vi "S4ICS 20240620.vi"() -> ()   [LabVIEW 2018]
uses:
  <vilib>/picture/picture.llb/imagedata.ctl
  MotorSim/MotorSim.lvclass
  StateManager/StateManager.lvclass
  Motor/Motor.lvclass
  StateManager/StateManager.lvclass/StateManager.ctl
  Messenger/Messenger.lvclass
  Motor/Motor.lvclass/Motor.ctl
  ICS/ICS.lvclass/ICS.ctl
  Message Queue/Message Cluster.ctl
  TCP-Server/TCP-Server.lvclass/TCP-Server.ctl
  TCP-Server/TCP-Server.lvclass
  ICS/ICS.lvclass
  Message Queue/Message Queue.lvlib
  MotorManager/MotorManager.lvclass
panel:
  out "version":string caption="vers."
  out "tab body":enum32{"Motors", "Config"}(tab)
  out "GFOC home":bool caption="Home"
  out "GFOC limit":bool caption="Limit"
  out "guider cam anime":picture
  out "gmir stat":T1
  out "ASEL Value":dbl
  out "CALW Value":dbl
  out "WPSEL Value":dbl
  out "GMIR Value":dbl
  out "WPROT Value":dbl
  out "GFOC Value":dbl
  out "calw stat":T1
  out "asel stat":T1
  out "wpsel stat":T1
  out "wprot stat":T1
  out "gfoc stat":T1
  out "asel lim on":bool caption="Limit ON"
  out "asel sec ON":bool caption="Sec. ON"
  out "asel lim off":bool caption="Limit OFF"
  out "asel sec off":bool caption="Sec. OFF"
  out "asel anime":picture
  out "asel background":picture
  out "wpsel sec/2":bool caption="Sec. L/4"
  out "wpsel sec/4":bool caption="Sec. L/2"
  out "wp home":bool caption="Home"
  out "wprot ctl":dbl(knob) scale=0.0..360.0
  out "wpsel lim/2":bool caption="Limit L/4"
  out "wpsel lim/4":bool caption="Limit L/2"
  out "wpsel anime":picture
  out "calw2":bool caption="CW 2"
  out "calw1":bool caption="CW 1"
  out "calw0":bool caption="CW 0"
  out "calw knob":cluster{dbl, dbl, dbl, dbl, dbl}(knob)={10.0, 82.0, 154.0, 226.0, 298.0} scale=0.0..360.0
  out "GMIR home":bool caption="Home"
  out "gmir knob":dbl(knob) scale=0.0..360.0
  out "asel image":T2
  in  "tips":T3(array[cluster])=[{"tip name"="login: server off", "PT"="Estado do servidor TCP/IP do S4ICS\npara clientes da rede (e.g. S4GUI).", "EN"="State of the S4ICS TCP/IP server\nfor network clients (e.g. S4GUI)."}, {"tip name"="login: exit", "PT"="Encerra a execução do programa\nS4ICS.", "EN"="Ends the execution of the S4ICS\nprogram."}, {"tip name"="login: language", "PT"="Seleciona a linguagem dos textos\nde ajuda e das dicas ou as ocultam.", "EN"="Select the language of the texts\nof help and tips or hide them."}, {"tip name"="login: user", "PT"="Nome cadastrado do usuário para\npermitir sua identificação.", "EN"="User's registered name to allow\nidentification."}, {"tip name"="login: password", "PT"="Senha cadastrada do usuário\n(digitada no 1o. acesso do usuário).", "EN"="User's registered password\n(entered on user's first login)."}, {"tip name"="login: help", "PT"="Descreve a função dos elementos\nmostrados no painel do S4ICS.", "EN"="Describes the function of elements\nshown on the S4ICS panel."}, {"tip name"="login: login", "PT"="Acesso ao S4ICS com a permissão\nestabelecida pelo administrador.", "EN"="Access to S4ICS according to\npermission set by administrator."}, {"tip name"="stopped: start srv", "PT"="Habilita o servidor TCP/IP do S4ICS\n(faz logout automaticamente).", "EN"="Enables S4ICS TCP/IP server\n(automatically logs out)."}, {"tip name"="stopped: exit", "PT"="Fecha o programa S4ICS.", "EN"="Ends S4ICS program execution."}, {"tip name"="stopped: assist", "PT"="Abre janela para testar e estacionar\nos mecanismos do instrumento.", "EN"="Opens window to test and park\ninstrument mechanisms."}, {"tip name"="stopped: setup", "PT"="Abre a janela de configuração do\ninstrumento (acesso restrito). ", "EN"="Opens the window of instrument\nconfiguration (restricted access)."}, {"tip name"="stopped: control", "PT"="Abre a janela para controlar os\nmecanismos (acesso restrito).", "EN"="Opens the window to control the\nmechanisms (restricted access)."}, {"tip name"="stopped: logout", "PT"="Libera o S4ICS para outro usuário.", "EN"="Release S4ICS for another user."}, {"tip name"="running: stop", "PT"="Desabilita o servidor\nTCP/IP doS4ICS.", "EN"="Disables S4ICS TCP/IP server."}, {"tip name"="running: logout", "PT"="Libera o S4ICS para outro usuário.", "EN"="Release S4ICS for another user."}, {"tip name"="setup: save", "PT"="Salva as alterações mantendo o\nnome do arquivo de  configuração.", "EN"="Save the changes keeping the\nname of the configuration file."}, {"tip name"="setup: save as", "PT"="Salva as alterações em um arquivo\nde  configuração com outro nome.", "EN"="Save changes to a file\nunder another name."}, {"tip name"="setup: help", "PT"="Descreve a função dos elementos\nmostrados no painel abaixo.", "EN"="Describes the function of elements\nshown on below panel."}, {"tip name"="setup: cfg file", "PT"="Nome do arquivo da\nconfiguração atual.\n", "EN"="File name of current configuration."}, {"tip name"="setup: cfg user", "PT"="Nome do usuário que salvou\na configuração atual.", "EN"="Username who saved\nthe current configuration."}, {"tip name"="setup: cfg date", "PT"="Data da configuração atual.", "EN"="Date of current configuration."}, {"tip name"="setup: return", "PT"="Retorna ao menu anterior.", "EN"="Return to previous menu."}, {"tip name"="assist: return", "PT"="Retorna ao menu anterior.", "EN"="Return to previous menu."}, {"tip name"="control: return", "PT"="Retorna ao menu anterior.", "EN"="Return to previous menu."}, {"tip name"="cfg: previous", "PT"="Mostra e seleciona\no usuário anterior.", "EN"="Show and select\nprevious user."}, {"tip name"="cfg: next", "PT"="Mostra e seleciona\no próximo usuário.", "EN"="Show and select\nthe next user."}, {"tip name"="cfg: delete", "PT"="Remove da lista o\nusuário selecionado.", "EN"="Remove from the list\nthe selected user."}, {"tip name"="cfg: name", "PT"="Nome do novo usuário\npara ser inserido na lista.", "EN"="New user name to be\ninserted into the list."}, {"tip name"="cfg: insert", "PT"="Insere na lista o novo usuário com\no nome e a permissão indicados.", "EN"="Insert the new user with the\ngiven name and permission."}, {"tip name"="cfg: permission", "PT"="Permissão do usuário. Restringir\nas atribuições Admin e Control.", "EN"="User permission. Restrict the\nAdmin and Control assignments."}, {"tip name"="cfg: change", "PT"="Atribui a atribuição ao lado\npara o usuário selecionado.", "EN"="Assign left assignment\nfor the selected user."}, {"tip name"="cfg: auto", "PT"="Tempo limite de inatividade para\nlogout automático do usuário.", "EN"="Inactivity timeout to\nautomatic user logout."}, {"tip name"="cfg: enable", "PT"="Permite o envio de e-mails\nde manutenção e configuração.", "EN"="Allows sending maintenance\nand configuration emails."}, {"tip name"="cfg: service", "PT"="Endereço IP e porta do\nservidor de e-mail.", "EN"="IP address and port\nof email server."}, {"tip name"="cfg: admin", "PT"="Endereço de e-mail que receberá\nnotificações de nova configuração.", "EN"="Email address that will receive\nnew configuration notifications."}, {"tip name"="cfg: maint", "PT"="Endereço de email que irá receber\nnotificações de erro e alarme.", "EN"="Email address that will receive\nerror and alarm notifications."}, {"tip name"="cfg: check", "PT"="Envia e-mail e confere recebimento\npara testar o servidor de e-mail.", "EN"="Send emails and check receipt\nto test the email server."}, {"tip name"="cfg: ok", "PT"="Resultado do teste do servidor de\ne-mail. Aguarde alguns segundos.", "EN"="Test result from email server test.\nPlease, wait a few seconds."}, {"tip name"="cfg: srv ip", "PT"="Endereço IP do servidor do S4ICS:\nlocalhost ou IP local (ver abaixo).", "EN"="S4ICS server IP address:\nlocalhost or local IP (see below)."}, {"tip name"="cfg: srv port", "PT"="Porta do servidor do S4ICS que\nserá usada pelos clientes (S4GUI).", "EN"="S4ICS server port used\nby clients (like S4GUI)."}, {"tip name"="cfg: srv timeout", "PT"="Tempo de espera pela conexão:\nmenor tempo exigido pelo servidor do S4ICS.", "EN"="Connection wait time: lower time\nrequired by S4ICS server."}, {"tip name"="cfg: IP1", "PT"="Porta IP ativa (com conexão)\nneste computador.", "EN"="Active IP port (with connection)\non this computer."}, {"tip name"="cfg: IP2", "PT"="Porta IP ativa (com conexão)\nneste computador.", "EN"="Active IP port (with connection)\non this computer."}]
  in  "pubTime0mq":i32=3000 caption="Pub Time*"
  in  "0mqEndpoint":string="tcp://*:54030" caption="PUB Socket (tcp://*:54030)*"
  in  "address":string="localhost" caption="Address"
  in  "runMinimized":bool
  in  "autoSS":bool
  in  "log help":bool
  in  "enabled log":string="012345" caption="LOG Enable"
  in  "WPSEL mode":string(combo)="Control" caption="Mechanism Mode"
  in  "CALW mode":string(combo)="Control" caption="Mechanism Mode"
  in  "GFOC mode":string(combo)="Control" caption="Mechanism Mode"
  in  "animation":bool
  in  "full init":bool
  in  "timeout":i32=100 caption="Timeout"
  in  "port":u16=54165 caption="Port"
  in  "pwrPM mains":bool=TRUE caption="Mains"
  in  "pwrPM password":string="ubnt" caption="Password"
  in  "pwrPM user":string="ubnt" caption="User"
  in  "pwrPM outlet":u16=5 caption="Outlet"
  in  "pwrPM port":u16=6080 caption="Port"
  in  "pwrPM ip":string="192.168.1.20" caption="IP"
  in  "pwrGD mains":bool=TRUE caption="Mains"
  in  "pwrGD password":string="ubnt" caption="Password"
  in  "pwrGD user":string="ubnt" caption="User"
  in  "pwrGD outlet":u16=6 caption="Outlet"
  in  "pwrGD port":u16=6080 caption="Port"
  in  "pwrGD ip":string="192.168.1.20" caption="IP"
  in  "GMIR disabled":bool
  in  "GMIR mode":string(combo)="Control" caption="Mechanism Mode"
  in  "GMIR ip":string="192.168.1.249" caption="ip"
  in  "GFOC positions":cluster{"pos_name":string, "pos_value":dbl}[](array[cluster])=[{"pos_name"="OFFSET", "pos_value"=0.0}] caption="GFOC" {"pos_value" min=-400.0 max=400.0 step=0.1}
  in  "GMIR positions":cluster{"pos_name":string, "pos_value":dbl}[](array[cluster])=[{"pos_name"="OFFSET", "pos_value"=0.0}] caption="GMIR" {"pos_value" min=-10.0 max=110.0 step=0.1}
  in  "WPSEL disabled":bool
  in  "WPROT disabled":bool
  in  "WPSEL ip":string="192.168.1.246" caption="ip"
  in  "WPROT mode":string(combo)="Control" caption="Mechanism Mode"
  in  "WPROT ip":string="192.168.1.245" caption="ip"
  in  "WPSEL positions":cluster{"pos_name":string, "pos_value":dbl}[](array[cluster])=[{"pos_name"="OFFSET", "pos_value"=0.0}, {"pos_name"="L/4", "pos_value"=0.0}, {"pos_name"="OFF", "pos_value"=400000.0}, {"pos_name"="L/2", "pos_value"=800000.0}] caption="WPSEL" {"pos_value" min=-400.0 max=400.0 step=0.1}
  in  "WPROT positions":cluster{"pos_name":string, "pos_value":dbl}[](array[cluster])=[{"pos_name"="OFFSET", "pos_value"=0.0}, {"pos_name"="WP1", "pos_value"=0.0}, {"pos_name"="WP2", "pos_value"=1875.0}, {"pos_name"="WP3", "pos_value"=3750.0}, {"pos_name"="WP4", "pos_value"=5625.0}, {"pos_name"="WP5", "pos_value"=7500.0}, {"pos_name"="WP6", "pos_value"=9375.0}, {"pos_name"="WP7", "pos_value"=11250.0}, {"pos_name"="WP8", "pos_value"=13125.0}, {"pos_name"="WP9", "pos_value"=15000.0}, {"pos_name"="WP10", "pos_value"=16875.0}, {"pos_name"="WP11", "pos_value"=18750.0}, {"pos_name"="WP12", "pos_value"=20625.0}, {"pos_name"="WP13", "pos_value"=22500.0}, {"pos_name"="WP14", "pos_value"=24375.0}, {"pos_name"="WP15", "pos_value"=26250.0}, {"pos_name"="WP16", "pos_value"=28125.0}] caption="WPROT" {"pos_value" min=-10.0 max=110.0 step=0.1}
  in  "CALW disabled":bool
  in  "ASEL disabled":bool
  in  "CALW ip":string="192.168.1.247" caption="ip"
  in  "ASEL mode":string(combo)="Control" caption="Mechanism Mode"
  in  "ASEL ip":string="192.168.1.248" caption="ip"
  in  "CALW positions":cluster{"pos_name":string, "pos_value":dbl}[](array[cluster])=[{"pos_name"="OFFSET", "pos_value"=0.0}, {"pos_name"="OFF", "pos_value"=0.0}, {"pos_name"="POLARIZER", "pos_value"=12000.0}, {"pos_name"="PINHOLE", "pos_value"=24000.0}, {"pos_name"="SHUTTER", "pos_value"=36000.0}, {"pos_name"="DEPOLARIZER", "pos_value"=48000.0}] caption="CALW" {"pos_value" min=-400.0 max=400.0 step=0.1}
  in  "ASEL positions":cluster{"pos_name":string, "pos_value":dbl}[](array[cluster])=[{"pos_name"="OFFSET", "pos_value"=0.0}, {"pos_name"="OFF", "pos_value"=0.0}, {"pos_name"="ON", "pos_value"=4800.0}] caption="ASEL" {"pos_value" min=-10.0 max=110.0 step=0.1}
  in  "S4ICS password":string="se4RFVgy&8"
  in  "S4ICS login":string="s4ics@lna.br"
  in  "S4ICS email":string="s4ics@lna.br" caption="S4ICS account"
  in  "auto logout":u32=200 caption="Auto Logout period" min=30 max=3000
  out "email ok":bool
  in  "check email":bool
  in  "maint. email":string="frodrigues@lna.br" caption="Maintenance"
  in  "admin email":string="nivaldo@lna.br" caption="Configuration"
  in  "email service":string="smtp.gmail.com:587" caption="Server IP:PORT"
  out "user list":T4(array[cluster]) caption="Name                 Permission        PW"
  in  "user delete":bool
  in  "user permission":string(combo)="Start / Stop" caption="Permission"
  in  "change permission":bool
  in  "user insert":bool
  in  "user name":string caption="New User"
  in  "user previous":bool
  in  "user next":bool
  in  "email enable":bool caption="Email service"
  in  "channel":T5(ring)=enum."Inner TCP/IP" caption="Channel"
  out "local IP 1":string
  out "local IP 2":string
  in  "comm help":bool
  out "tab menu":T6(tab)
  in  "login help":bool
  in  "loginPW":string caption="Password"
  in  "loginUser":string caption="User Name"
  in  "login":bool
  out "server":bool
  in  "exitLogin":bool
  in  "language":enum32{"PT", "EN", "NONE"}(radio)=enum."NONE"
  in  "stop server":bool
  in  "logout running":bool
  in  "exitStopped":bool
  in  "logout stopped":bool
  in  "start server":bool
  in  "control":bool
  in  "setup":bool
  in  "assist":bool
  in  "return assist":bool
  in  "save as":bool
  out "last cfg date":string caption="Date"
  out "last cfg user":string caption="User"
  in  "save config":bool
  in  "return setup":bool
  in  "config help":bool
  out "cfgFile":string caption="CONFIG FILE"
  out "control response":string caption="Response"
  in  "control instruction":string caption="Instruction"
  in  "control send":bool
  in  "control jump":bool caption="JUMP"
  in  "control position":dbl caption="Mech. Position"
  in  "return control":bool
  in  "control stop":bool
  in  "control motor sel":T7(radio) caption="Motor"
  # "GFOC - Guiding Focuser"
  # "GMIR - Guiding Mirror"
  # "CALW - Calibration Wheel"
  # "FOCUSER"
  # "CLEAR"
  # "GUIDING"
  # "CAMERA"
  # "POLARIZER"
  # "PINHOLE"
  # "SHUTTER"
  # "PATROL"
  # "MIRROR"
  # "DEPOLARIZER"
  # "WPROT - Waveplate Rotator"
  # "WPSEL - Waveplate Selector"
  # "ASEL - Analyser Selector"
  # "POLARIMETRIC MECHANISMS"
  # "SERVER COMMUNICATION"
  # "USER LIST"
  # "(*) Requires EXIT after SAVE\n      Exigido EXIT depois de SAVE"
  # "SIMULATION"
  # "ANIMATION"
  # "ON"
  # "FAST"
  # "FULL"
  # "OFF"
  # "s"
  # "EMAIL SETTINGS"
  # "GUIDING MECHANISMS"
  # "POWER"
  # "POWER"
  # "GMIR & GFOC"
  # "GFOC motor is driven by the GMIR cotroller."
  # "IDENTIFICATION"
  # "LAST CONFIGURATION"
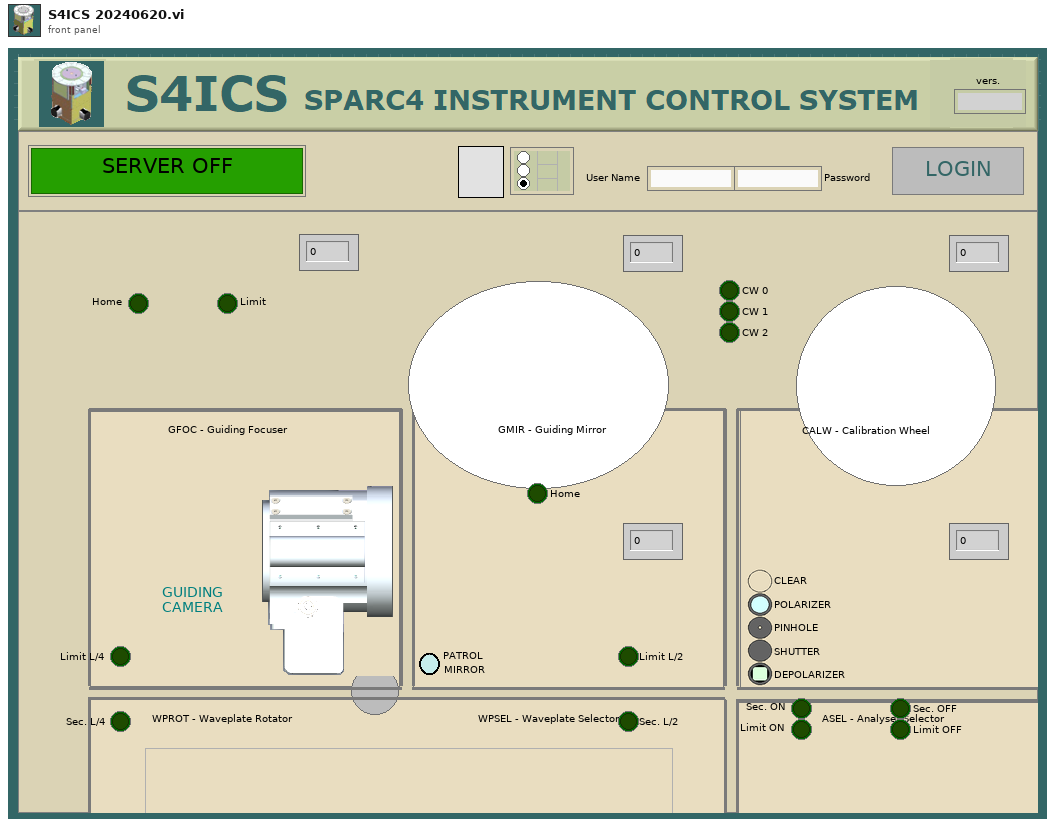
[diagram p1: front panel]
types:
  T1 = cluster{"mode":string, "condition":string, "position":string, "pos_name":string, "pos_id":string}
  T2 = typedef "imagedata.ctl" = cluster{"image type":i32, "image depth":i32, "image":u8[], "mask":u8[], "colors":u32[], "Rectangle":cluster{"left":i16, "top":i16, "right":i16, "bottom":i16}}
  T3 = cluster{"tip name":string, "PT":string, "EN":string}[]
  T4 = cluster{"name":string, "permission":string, "password":string}[]
  T5 = enum32{"Local Panel", "Inner TCP/IP", "Outer TCP/IP", "MQTT", "ZeroMQ"}
  T6 = enum32{"Login", "Running", "Stopped", "Assist", "Setup", "Control"}
  T7 = enum32{"No Selection", "control WPROT", "control WPSEL", "control ASEL", "control CALW", "control GFOC", "control GMIR"}
  T8 = cluster{"S4commandQueueName":string, "S4statusQueueName":string, "comm configuration":cluster{"channel":enum32{"Local Panel", "Inner TCP/IP", "Outer TCP/IP", "MQTT", "ZeroMQ"}, "address":string, "port":u16, "timeout":i32}}
  T9 = enum32{"Motors", "Config", "Status", "Anime", "Param"}
  T10 = cluster{"email service":string, "maint. email":string, "admin email":string, "S4ICS email":string, "S4ICS login":string, "S4ICS password":string, "email enabled":bool}
  T11 = cluster{"period":u32, "initial position (0)":i32, "translation (100)":i32, "forward":bool}[]
  T12 = enum8{"Enabled", "Disabled", "Disabled and Grayed Out"}
  T13 = enum32{"Invalid", "Standard", "Closed", "Hidden", "Minimized", "Maximized"}
  T14 = cluster{"left":i16, "top":i16, "right":i16, "bottom":i16}
  T15 = enum32{"Login", "Stopped", "Running", "Setup", "Assist", "Control"}
  T16 = enum16{"Wait", "ActiveInit", "ActiveGoto", "ActiveUpdate", "ActiveStop", "ActiveFinish", "SimInit", "SimGoto", "SimUptate", "SimFinish", "CyclicStart", "CyclicUpdate", "CyclicFinish"}
  T17 = cluster{"action":string, "param":string, "pos_name":string, "pos_idx":i32, "ack":bool, "stop":bool, "offset":bool, "immediate":bool, "instructions":string[]}
  T18 = typedef "Message Queue.lvlib/Message Cluster.ctl" = cluster{"Message":string, "Message Data":variant}
  T19 = cluster{"channel":enum32{"Local Panel", "Inner TCP/IP", "Outer TCP/IP", "MQTT", "ZeroMQ"}, "address":string, "port":u16, "timeout":i32}
  T20 = cluster{"name":string, "permission":string, "password":string}
  T21 = cluster{"[0]":dbl, "[1]":dbl, "[2]":dbl, "[3]":dbl, "[4]":dbl}
  T22 = enum32{"invalid app kind", "Development System", "Run Time System", "Student Edition", "Embedded LabVIEW", "Evaluation", "Custom"}
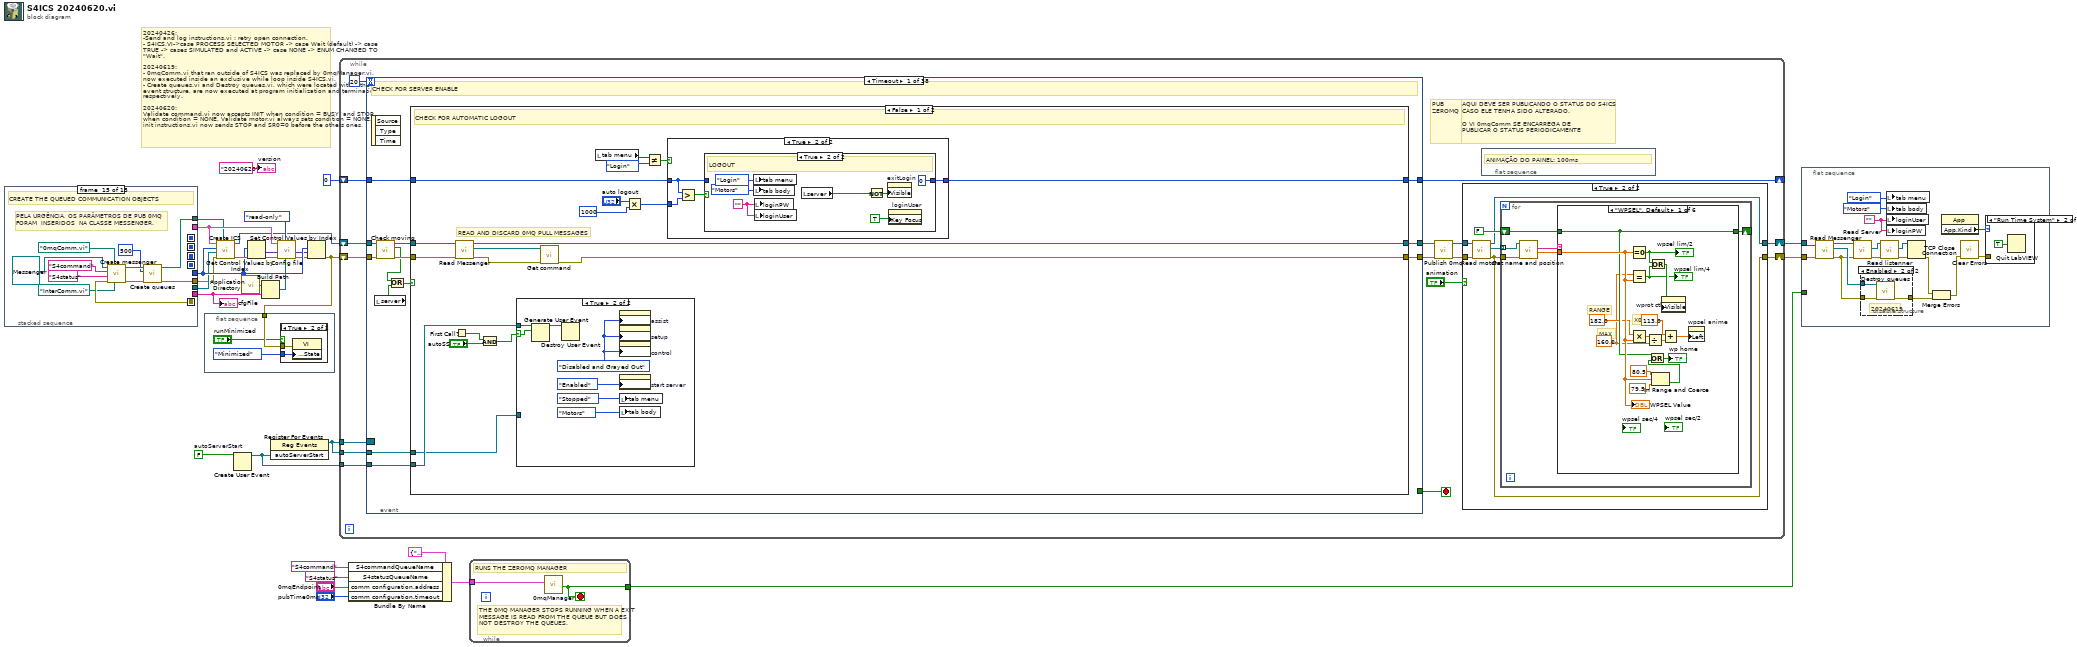
[diagram p0: block diagram]
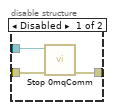
[diagram p3: hidden frame]
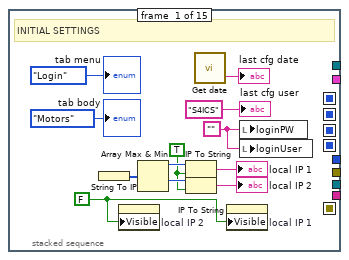
[diagram p5: hidden frame]
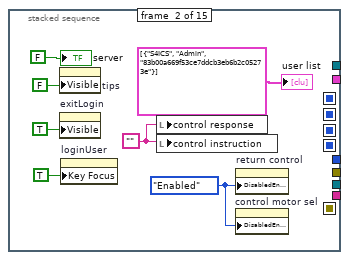
[diagram p6: hidden frame]
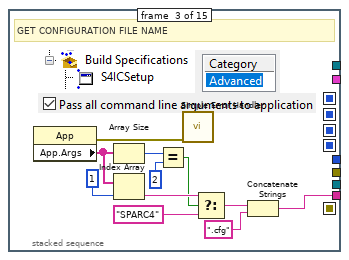
[diagram p7: hidden frame]
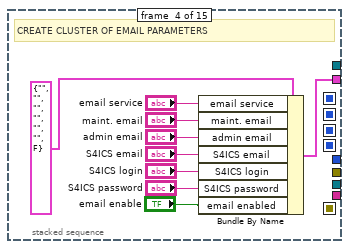
[diagram p8: hidden frame]
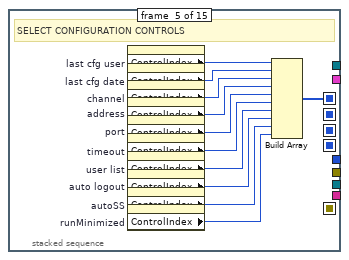
[diagram p9: hidden frame]
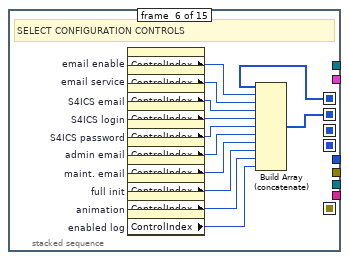
[diagram p10: hidden frame]
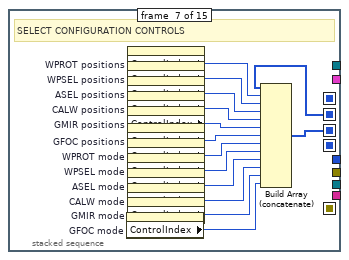
[diagram p11: hidden frame]
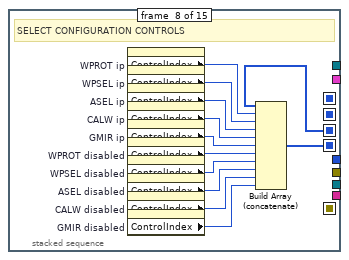
[diagram p12: hidden frame]
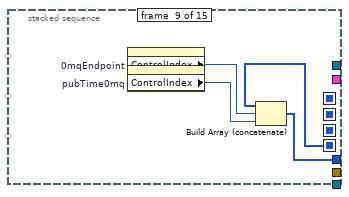
[diagram p13: hidden frame]
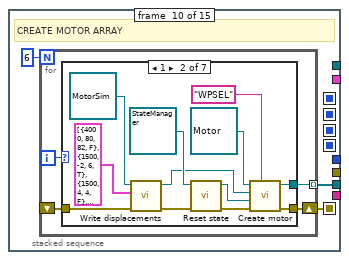
[diagram p14: hidden frame]
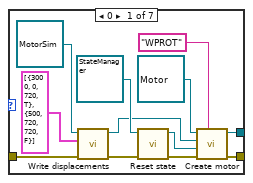
[diagram p15: hidden frame]
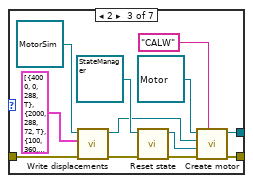
[diagram p16: hidden frame]
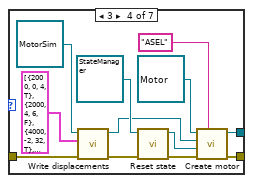
[diagram p17: hidden frame]
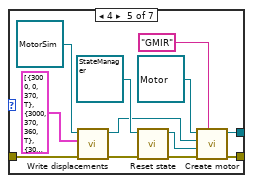
[diagram p18: hidden frame]
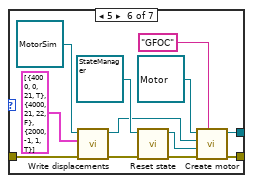
[diagram p19: hidden frame]
diagram:
  w12 = FALSE  # autoServerStart
  # "20240426:\n-Send and log instructions.vi : retry open connection.\n- S4ICS.VI->case PROCESS SELECTED MOTOR -> case Wait (default) -> case TRUE -> cases SIMULATED and ACTIVE -> case NONE -> ENUM CHANGED TO  \"Wait\".\n\n20240619:\n- 0mqComm.vi that ran outside of S4ICS was replaced by 0mqManager.vi, now executed inside an exclusive while loop inside S4ICS.vi.\n- Create queues.vi and Destroy queues.vi, which were located within the event structure, are now executed at program initialization and termination, respectively.\n\n20240620:\nValidate command.vi now accepts INIT when condition = BUSY, and STOP when condition = NONE. Validate motor.vi always sets condition = NONE. Get init instructions.vi now sends STOP and SR0=0 before the others ones."
  n1 = stacked-sequence {
    seq-local: [_ _ _ _ w78 _ _ _ _ _ _ _ _ _ _] -> [_ _ _ _ _ w92 _ _ _ _ _ _ _ _ _]
    seq-local: [_ _ _ _ _ w84 _ _ _ _ _ _ _ _ _] -> [_ _ _ _ _ _ w99 _ _ _ _ _ _ _ _]
    seq-local: [_ _ _ _ _ _ w98 _ _ _ _ _ _ _ _] -> [_ _ _ _ _ _ _ w118 _ _ _ _ _ _ _]
    seq-local: [_ _ _ _ _ _ _ _ _ w124 _ _ _ _ _] -> [_ _ _ _ _ _ _ _ _ _ _ _ _ _ w240]
    seq-local: [_ _ _ _ _ _ _ w107 _ _ _ _ _ _ _] -> [_ _ _ _ _ _ _ _ w122 _ _ _ _ _ _]
    tunnel: [_ _ w58 _ _ _ _ _ _ _ _ _ _ _ _] -> w27
    tunnel: [_ _ _ w61 _ _ _ _ _ _ _ _ _ _ _] -> w24
    tunnel: [_ _ _ _ _ _ _ _ w121 _ _ _ _ _ _] -> w26
    tunnel: [_ _ _ _ _ _ _ _ _ w125 _ _ _ _ _] -> w25
    tunnel: [_ _ _ _ _ _ _ _ _ _ _ _ _ _ w235] -> w15
    tunnel: [_ _ _ _ _ _ _ _ _ _ _ _ _ _ w234] -> w14
    frame #0 {
      w31 = FALSE
      w37 = TRUE
      w32 = ""
      # "INITIAL SETTINGS"
      n2 = String To IP() -> (0:w40:u32[])  [unwired: 1 in]
      n3 = property on="local IP 2" class="Str"("Visible"=w31) -> ()  [unwired: 2 in, 2 out]
      n4 = Array Max & Min(array=w40) -> (max value=w39:u32, min value=w38:u32)  [unwired: 2 out]
      n5 = IP To String(1:w37, 2:w39) -> (0:→"local IP 1":string)
      n6 = IP To String(1:w37, 2:w38) -> (0:→"local IP 2":string)
      n7 = call "Get date.vi"() -> ("date/time string"=→"last cfg date":string)  [unwired: 3 in]
      n8 = property on="local IP 1" class="Str"("Visible"=w31) -> ()  [unwired: 2 in, 2 out]
      n9 = local write "loginPW"(w32) -> ()
      n10 = local write "loginUser"(w32) -> ()
      "last cfg user" <- "S4ICS" ("last user")
      "tab menu" <- T6."Login" ("tab menu")
      "tab body" <- T9."Motors" ("tab body")
    }
    frame #1 {
      w43 = ""
      w44 = T12."Enabled" ("Disabled")
      n11 = property on="tips" class="Arr (strict)"("Visible"=FALSE) -> ()  [unwired: 2 in, 2 out]
      n12 = property on="exitLogin" class="Bool"("Visible"=TRUE) -> ()  [unwired: 2 in, 2 out]
      n13 = property on="loginUser" class="Str"("Key Focus"=TRUE) -> ()  [unwired: 2 in, 2 out]
      n14 = local write "control response"(w43) -> ()
      n15 = local write "control instruction"(w43) -> ()
      n16 = property on="return control" class="Bool"("DisabledEnum"=w44) -> ()  [unwired: 2 in, 2 out]
      n17 = property on="control motor sel" class="RadioBtnsControl (strict)"("DisabledEnum"=w44) -> ()  [unwired: 2 in, 2 out]
      "server" <- FALSE
      "user list" <- T4 [{"name"="S4ICS", "permission"="Admin", "password"="83b00a669f53ce7ddcb3eb6b2c05273e"}] ("users")
    }
    frame #2 {
      # "GET CONFIGURATION FILE NAME"
      n18 = property class="App"() -> (error out=w59:errorcluster, "App.Args"=w55:string[])  [unwired: 2 in, 1 out]
      n19 = Array Size(array=w55) -> (size(s)=w57:i32)
      n20 = Index Array(array=w55, index=1) -> (element=w54:string)
      n21 = Equal?(x=w57, y=2 ("x")) -> (x = y?=w50:bool)
      n22 = call <vilib>:"Simple Error Handler.vi"("error in (no error)"=w59) -> ()  [unwired: 4 in, 5 out]
      n23 = Select(t=w54, s=w50, f="SPARC4" ("string")) -> (s? t:f=w52:string)
      n24 = Concatenate Strings(w52, ".cfg" ("string")) -> (w58:string)
    }
    frame #3 {
      # "CREATE CLUSTER OF EMAIL PARAMETERS"
      n25 = Bundle By Name(cluster=T10 {"email service"="", "maint. email"="", "admin email"="", "S4ICS email"="", "S4ICS login"="", "S4ICS password"="", "email enabled"=FALSE} ("email cluster"), "email service"="email service", "maint. email"="maint. email", "admin email"="admin email", "S4ICS email"="S4ICS email", "S4ICS login"="S4ICS login", "S4ICS password"="S4ICS password", "email enabled"="email enable") -> (w61:T10)
    }
    frame #4 {
      # "SELECT CONFIGURATION CONTROLS"
      n26 = property on="last cfg user" class="Str"() -> ("ControlIndex"=w79:i32)  [unwired: 2 in, 2 out]
      n27 = property on="last cfg date" class="Str"() -> ("ControlIndex"=w80:i32)  [unwired: 2 in, 2 out]
      n28 = property on="channel" class="Enum (strict)"() -> ("ControlIndex"=w72:i32)  [unwired: 2 in, 2 out]
      n29 = property on="address" class="Str"() -> ("ControlIndex"=w73:i32)  [unwired: 2 in, 2 out]
      n30 = property on="port" class="DigNum (strict)"() -> ("ControlIndex"=w74:i32)  [unwired: 2 in, 2 out]
      n31 = property on="timeout" class="DigNum (strict)"() -> ("ControlIndex"=w75:i32)  [unwired: 2 in, 2 out]
      n32 = property on="user list" class="Arr (strict)"() -> ("ControlIndex"=w76:i32)  [unwired: 2 in, 2 out]
      n33 = property on="auto logout" class="DigNum (strict)"() -> ("ControlIndex"=w77:i32)  [unwired: 2 in, 2 out]
      n34 = property on="autoSS" class="Bool (strict)"() -> ("ControlIndex"=w71:i32)  [unwired: 2 in, 2 out]
      n35 = property on="runMinimized" class="Bool (strict)"() -> ("ControlIndex"=w70:i32)  [unwired: 2 in, 2 out]
      n36 = Build Array(w79, w80, w72, w73, w74, w75, w76, w77, w71, w70) -> (w78:i32[])
    }
    frame #5 {
      # "SELECT CONFIGURATION CONTROLS"
      n37 = property on="email enable" class="Bool (strict)"() -> ("ControlIndex"=w88:i32)  [unwired: 2 in, 2 out]
      n38 = property on="email service" class="Str"() -> ("ControlIndex"=w89:i32)  [unwired: 2 in, 2 out]
      n39 = property on="S4ICS email" class="Str"() -> ("ControlIndex"=w90:i32)  [unwired: 2 in, 2 out]
      n40 = property on="S4ICS login" class="Str"() -> ("ControlIndex"=w91:i32)  [unwired: 2 in, 2 out]
      n41 = property on="S4ICS password" class="Str"() -> ("ControlIndex"=w87:i32)  [unwired: 2 in, 2 out]
      n42 = property on="admin email" class="Str"() -> ("ControlIndex"=w86:i32)  [unwired: 2 in, 2 out]
      n43 = property on="maint. email" class="Str"() -> ("ControlIndex"=w85:i32)  [unwired: 2 in, 2 out]
      n44 = property on="full init" class="Bool (strict)"() -> ("ControlIndex"=w83:i32)  [unwired: 2 in, 2 out]
      n45 = property on="animation" class="Bool (strict)"() -> ("ControlIndex"=w82:i32)  [unwired: 2 in, 2 out]
      n46 = property on="enabled log" class="Str"() -> ("ControlIndex"=w81:i32)  [unwired: 2 in, 2 out]
      n47 = Build Array (concatenate)(w92, w88, w89, w90, w91, w87, w86, w85, w83, w82, w81) -> (w84:i32[])
    }
    frame #6 {
      # "SELECT CONFIGURATION CONTROLS"
      n48 = property on="GFOC mode" class="CmbBox"() -> ("ControlIndex"=w97:i32)  [unwired: 2 in, 2 out]
      n49 = property on="WPROT positions" class="Arr (strict)"() -> ("ControlIndex"=w102:i32)  [unwired: 2 in, 2 out]
      n50 = property on="WPSEL positions" class="Arr (strict)"() -> ("ControlIndex"=w103:i32)  [unwired: 2 in, 2 out]
      n51 = property on="ASEL positions" class="Arr (strict)"() -> ("ControlIndex"=w104:i32)  [unwired: 2 in, 2 out]
      n52 = property on="CALW positions" class="Arr (strict)"() -> ("ControlIndex"=w105:i32)  [unwired: 2 in, 2 out]
      n53 = property on="GMIR positions" class="Arr (strict)"() -> ("ControlIndex"=w106:i32)  [unwired: 2 in, 2 out]
      n54 = property on="GFOC positions" class="Arr (strict)"() -> ("ControlIndex"=w101:i32)  [unwired: 2 in, 2 out]
      n55 = property on="WPROT mode" class="CmbBox"() -> ("ControlIndex"=w100:i32)  [unwired: 2 in, 2 out]
      n56 = property on="WPSEL mode" class="CmbBox"() -> ("ControlIndex"=w93:i32)  [unwired: 2 in, 2 out]
      n57 = property on="ASEL mode" class="CmbBox"() -> ("ControlIndex"=w94:i32)  [unwired: 2 in, 2 out]
      n58 = property on="CALW mode" class="CmbBox"() -> ("ControlIndex"=w95:i32)  [unwired: 2 in, 2 out]
      n59 = property on="GMIR mode" class="CmbBox"() -> ("ControlIndex"=w96:i32)  [unwired: 2 in, 2 out]
      n60 = Build Array (concatenate)(w99, w102, w103, w104, w105, w106, w101, w100, w93, w94, w95, w96, w97) -> (w98:i32[])
    }
    frame #7 {
      # "SELECT CONFIGURATION CONTROLS"
      n61 = property on="WPROT ip" class="Str"() -> ("ControlIndex"=w117:i32)  [unwired: 2 in, 2 out]
      n62 = property on="WPSEL ip" class="Str"() -> ("ControlIndex"=w116:i32)  [unwired: 2 in, 2 out]
      n63 = property on="ASEL ip" class="Str"() -> ("ControlIndex"=w115:i32)  [unwired: 2 in, 2 out]
      n64 = property on="CALW ip" class="Str"() -> ("ControlIndex"=w114:i32)  [unwired: 2 in, 2 out]
      n65 = property on="GMIR ip" class="Str"() -> ("ControlIndex"=w113:i32)  [unwired: 2 in, 2 out]
      n66 = property on="WPROT disabled" class="Bool (strict)"() -> ("ControlIndex"=w112:i32)  [unwired: 2 in, 2 out]
      n67 = property on="WPSEL disabled" class="Bool (strict)"() -> ("ControlIndex"=w111:i32)  [unwired: 2 in, 2 out]
      n68 = property on="ASEL disabled" class="Bool (strict)"() -> ("ControlIndex"=w110:i32)  [unwired: 2 in, 2 out]
      n69 = property on="CALW disabled" class="Bool (strict)"() -> ("ControlIndex"=w109:i32)  [unwired: 2 in, 2 out]
      n70 = property on="GMIR disabled" class="Bool (strict)"() -> ("ControlIndex"=w108:i32)  [unwired: 2 in, 2 out]
      n71 = Build Array (concatenate)(w118, w117, w116, w115, w114, w113, w112, w111, w110, w109, w108) -> (w107:i32[])
    }
    frame #8 {
      n72 = property on="0mqEndpoint" class="Str"() -> ("ControlIndex"=w120:i32)  [unwired: 2 in, 2 out]
      n73 = property on="pubTime0mq" class="DigNum (strict)"() -> ("ControlIndex"=w119:i32)  [unwired: 2 in, 2 out]
      n74 = Build Array (concatenate)(w122, w120, w119) -> (w121:i32[])
    }
    frame #9 {
      # "CREATE MOTOR ARRAY"
      n75 = for {
        N: 6 -> [_]
        shift-right: [w129] -> w124
        shift-left: _ -> [w128]
        tunnel: [w127] -> w125 mode=indexing
        i -> [w126]
        n76 = case shown="1" w126 {
          tunnel: [w141 w153 w165 w177 w189 w201 w202] -> w129
          tunnel: w128 -> [w140 w152 w164 w176 w188 w200 w202]
          tunnel: [w134 w146 w158 w170 w182 w194 _] -> w127
          frame 0 {
            n77 = call-dynamic "Write displacements.vi"("error in (no error)"=w140, "displacements"=T11 [{"period"=3000, "initial position (0)"=0, "translation (100)"=720, "forward"=TRUE}, {"period"=500, "initial position (0)"=720, "translation (100)"=720, "forward"=FALSE}] ("WPROT moves"), "MotorSim in"=refnum<class "MotorSim.lvclass"> refnum ("MotorSim.lvclass")) -> ("error out"=w135:errorcluster, "MotorSim out"=w132:refnum<class "MotorSim.lvclass">)  [unwired: 7 in]
            n78 = call "Reset state.vi"("error in (no error)"=w135, "StateManager in"=refnum<class "StateManager.lvclass"> refnum ("StateManager.lvclass")) -> ("error out"=w139:errorcluster, "StateManager out"=w133:refnum<class "StateManager.lvclass">)  [unwired: 8 in]
            n79 = call-dynamic "Create motor.vi"("name"="WPROT", "error in (no error)"=w139, "StateManager"=w133, "MotorSim"=w132, "Motor in"=refnum<class "Motor.lvclass"> refnum ("Motor.lvclass")) -> ("error out"=w141:errorcluster, "Motor out"=w134:refnum<class "Motor.lvclass">)  [unwired: 5 in]
          }
          frame 1 {
            n80 = call-dynamic "Write displacements.vi"("error in (no error)"=w152, "displacements"=T11 [{"period"=4000, "initial position (0)"=80, "translation (100)"=82, "forward"=FALSE}, {"period"=1500, "initial position (0)"=-2, "translation (100)"=6, "forward"=TRUE}, {"period"=1500, "initial position (0)"=4, "translation (100)"=4, "forward"=FALSE}, {"period"=6000, "initial position (0)"=0, "translation (100)"=80, "forward"=TRUE}, {"period"=6000, "initial position (0)"=80, "translation (100)"=82, "forward"=TRUE}, {"period"=2000, "initial position (0)"=162, "translation (100)"=6, "forward"=FALSE}, {"period"=2000, "initial position (0)"=156, "translation (100)"=156, "forward"=FALSE}] ("WPSEL moves"), "MotorSim in"=refnum<class "MotorSim.lvclass"> refnum ("MotorSim.lvclass")) -> ("error out"=w147:errorcluster, "MotorSim out"=w144:refnum<class "MotorSim.lvclass">)  [unwired: 7 in]
            n81 = call "Reset state.vi"("error in (no error)"=w147, "StateManager in"=refnum<class "StateManager.lvclass"> refnum ("StateManager.lvclass")) -> ("error out"=w151:errorcluster, "StateManager out"=w145:refnum<class "StateManager.lvclass">)  [unwired: 8 in]
            n82 = call-dynamic "Create motor.vi"("name"="WPSEL", "error in (no error)"=w151, "StateManager"=w145, "MotorSim"=w144, "Motor in"=refnum<class "Motor.lvclass"> refnum ("Motor.lvclass")) -> ("error out"=w153:errorcluster, "Motor out"=w146:refnum<class "Motor.lvclass">)  [unwired: 5 in]
          }
          frame 2 {
            n83 = call-dynamic "Write displacements.vi"("error in (no error)"=w164, "displacements"=T11 [{"period"=4000, "initial position (0)"=0, "translation (100)"=288, "forward"=TRUE}, {"period"=2000, "initial position (0)"=288, "translation (100)"=72, "forward"=TRUE}, {"period"=100, "initial position (0)"=360, "translation (100)"=360, "forward"=FALSE}, {"period"=1200, "initial position (0)"=0, "translation (100)"=72, "forward"=TRUE}, {"period"=1200, "initial position (0)"=72, "translation (100)"=72, "forward"=TRUE}, {"period"=1200, "initial position (0)"=144, "translation (100)"=72, "forward"=TRUE}, {"period"=1200, "initial position (0)"=216, "translation (100)"=72, "forward"=TRUE}, {"period"=1200, "initial position (0)"=288, "translation (100)"=72, "forward"=TRUE}, {"period"=100, "initial position (0)"=360, "translation (100)"=360, "forward"=FALSE}] ("CALW moves"), "MotorSim in"=refnum<class "MotorSim.lvclass"> refnum ("MotorSim.lvclass")) -> ("error out"=w159:errorcluster, "MotorSim out"=w156:refnum<class "MotorSim.lvclass">)  [unwired: 7 in]
            n84 = call "Reset state.vi"("error in (no error)"=w159, "StateManager in"=refnum<class "StateManager.lvclass"> refnum ("StateManager.lvclass")) -> ("error out"=w163:errorcluster, "StateManager out"=w157:refnum<class "StateManager.lvclass">)  [unwired: 8 in]
            n85 = call-dynamic "Create motor.vi"("name"="CALW", "error in (no error)"=w163, "StateManager"=w157, "MotorSim"=w156, "Motor in"=refnum<class "Motor.lvclass"> refnum ("Motor.lvclass")) -> ("error out"=w165:errorcluster, "Motor out"=w158:refnum<class "Motor.lvclass">)  [unwired: 5 in]
          }
          frame 3 {
            n86 = call-dynamic "Write displacements.vi"("error in (no error)"=w176, "displacements"=T11 [{"period"=2000, "initial position (0)"=0, "translation (100)"=4, "forward"=TRUE}, {"period"=2000, "initial position (0)"=4, "translation (100)"=6, "forward"=FALSE}, {"period"=4000, "initial position (0)"=-2, "translation (100)"=32, "forward"=TRUE}, {"period"=2000, "initial position (0)"=30, "translation (100)"=2, "forward"=FALSE}, {"period"=4000, "initial position (0)"=28, "translation (100)"=28, "forward"=FALSE}] ("ASEL moves"), "MotorSim in"=refnum<class "MotorSim.lvclass"> refnum ("MotorSim.lvclass")) -> ("error out"=w171:errorcluster, "MotorSim out"=w168:refnum<class "MotorSim.lvclass">)  [unwired: 7 in]
            n87 = call "Reset state.vi"("error in (no error)"=w171, "StateManager in"=refnum<class "StateManager.lvclass"> refnum ("StateManager.lvclass")) -> ("error out"=w175:errorcluster, "StateManager out"=w169:refnum<class "StateManager.lvclass">)  [unwired: 8 in]
            n88 = call-dynamic "Create motor.vi"("name"="ASEL", "error in (no error)"=w175, "StateManager"=w169, "MotorSim"=w168, "Motor in"=refnum<class "Motor.lvclass"> refnum ("Motor.lvclass")) -> ("error out"=w177:errorcluster, "Motor out"=w170:refnum<class "Motor.lvclass">)  [unwired: 5 in]
          }
          frame 4 {
            n89 = call-dynamic "Write displacements.vi"("error in (no error)"=w188, "displacements"=T11 [{"period"=3000, "initial position (0)"=0, "translation (100)"=370, "forward"=TRUE}, {"period"=3000, "initial position (0)"=370, "translation (100)"=360, "forward"=TRUE}, {"period"=3000, "initial position (0)"=710, "translation (100)"=350, "forward"=TRUE}, {"period"=100, "initial position (0)"=0, "translation (100)"=0, "forward"=TRUE}] ("WPROT moves"), "MotorSim in"=refnum<class "MotorSim.lvclass"> refnum ("MotorSim.lvclass")) -> ("error out"=w183:errorcluster, "MotorSim out"=w180:refnum<class "MotorSim.lvclass">)  [unwired: 7 in]
            n90 = call "Reset state.vi"("error in (no error)"=w183, "StateManager in"=refnum<class "StateManager.lvclass"> refnum ("StateManager.lvclass")) -> ("error out"=w187:errorcluster, "StateManager out"=w181:refnum<class "StateManager.lvclass">)  [unwired: 8 in]
            n91 = call-dynamic "Create motor.vi"("name"="GMIR", "error in (no error)"=w187, "StateManager"=w181, "MotorSim"=w180, "Motor in"=refnum<class "Motor.lvclass"> refnum ("Motor.lvclass")) -> ("error out"=w189:errorcluster, "Motor out"=w182:refnum<class "Motor.lvclass">)  [unwired: 5 in]
          }
          frame 5 {
            n92 = call-dynamic "Write displacements.vi"("error in (no error)"=w200, "displacements"=T11 [{"period"=4000, "initial position (0)"=0, "translation (100)"=21, "forward"=TRUE}, {"period"=4000, "initial position (0)"=21, "translation (100)"=22, "forward"=FALSE}, {"period"=2000, "initial position (0)"=-1, "translation (100)"=1, "forward"=TRUE}] ("GFOC moves"), "MotorSim in"=refnum<class "MotorSim.lvclass"> refnum ("MotorSim.lvclass")) -> ("error out"=w195:errorcluster, "MotorSim out"=w192:refnum<class "MotorSim.lvclass">)  [unwired: 7 in]
            n93 = call "Reset state.vi"("error in (no error)"=w195, "StateManager in"=refnum<class "StateManager.lvclass"> refnum ("StateManager.lvclass")) -> ("error out"=w199:errorcluster, "StateManager out"=w193:refnum<class "StateManager.lvclass">)  [unwired: 8 in]
            n94 = call-dynamic "Create motor.vi"("name"="GFOC", "error in (no error)"=w199, "StateManager"=w193, "MotorSim"=w192, "Motor in"=refnum<class "Motor.lvclass"> refnum ("Motor.lvclass")) -> ("error out"=w201:errorcluster, "Motor out"=w194:refnum<class "Motor.lvclass">)  [unwired: 5 in]
          }
          frame 6, Default {
            # "Useless case: just to take \n\"Default\" from others."
          }
        }
      }
    }
    frame #10 {
      # "CONTROLS WAITING FOR IMPLEMENTATION"
    }
    frame #11 {
      w203 = sgl 0.5 ("Zoom Factor")
      # "ANIMATION: GFOC, GMIR, AND CALW"
      n95 = call <vilib>:"Application Directory.vi"() -> ("Application Directory"=w211:path)
      n96 = property on="calw knob" class="Knob (strict)"("Scale.Visible"=FALSE) -> ()  [unwired: 2 in, 2 out]
      n97 = property on="gmir knob" class="Knob (strict)"("Scale.Visible"=FALSE) -> ()  [unwired: 2 in, 2 out]
      n98 = Build Path(base path=w211, name or relative path="Custom\\Luca transparent.png") -> (appended path=w212:path)
      n99 = call <vilib>:"Read PNG File.vi"("path to PNG file"=w212) -> ("image data"=w209:T2)  [unwired: 8 in, 2 out]
      n100 = call <vilib>:"Draw Flattened Pixmap.vi"("image data"=w209, "picture"=picture data[5B]) -> ("new picture"=→"guider cam anime":picture)  [unwired: 7 in]
      n101 = property on="asel background" class="Pict"("ZoomFactor"=w203) -> ()  [unwired: 2 in, 2 out]
      n102 = property on="asel anime" class="Pict"("ZoomFactor"=w203) -> ()  [unwired: 2 in, 2 out]
      "calw knob" <- cluster{dbl, dbl, dbl, dbl, dbl} {0.0, 72.0, 144.0, 216.0, 288.0} ("Knob")
    }
    frame #12 {
      # "ANIMATION: WPROT, WPSEL, AND ASEL"
      n103 = call <vilib>:"Application Directory.vi"() -> ("Application Directory"=w228:path)
      n104 = call <vilib>:"Application Directory.vi"() -> ("Application Directory"=w218:path)
      n105 = call <vilib>:"Application Directory.vi"() -> ("Application Directory"=w222:path)
      n106 = Build Path(base path=w228, name or relative path="Custom\\wpsel transparent.png") -> (appended path=w229:path)
      n107 = Build Path(base path=w218, name or relative path="Custom\\asel transparent.png") -> (appended path=w217:path)
      n108 = Build Path(base path=w222, name or relative path="Custom\\asel background.png") -> (appended path=w223:path)
      n109 = call <vilib>:"Read PNG File.vi"("path to PNG file"=w229) -> ("image data"=w226:T2)  [unwired: 8 in, 2 out]
      n110 = call <vilib>:"Read PNG File.vi"("path to PNG file"=w223) -> ("image data"=w221:T2)  [unwired: 8 in, 2 out]
      n111 = call <vilib>:"Draw Flattened Pixmap.vi"("image data"=w226, "picture"=picture data[5B]) -> ("new picture"=→"wpsel anime":picture)  [unwired: 7 in]
      n112 = call <vilib>:"Read PNG File.vi"("path to PNG file"=w217) -> ("image data"=→"asel image":T2)  [unwired: 8 in, 2 out]
      n113 = call <vilib>:"Draw Flattened Pixmap.vi"("image data"=w221, "picture"=picture data[5B]) -> ("new picture"=→"asel background":picture)  [unwired: 7 in]
      n114 = property on="asel image" class="Clust (strict)"("Visible"=FALSE) -> ()  [unwired: 2 in, 2 out]
    }
    frame #13 {
      w230 = TRUE
      w231 = FALSE
      # "MECHANISM STATUS DISPLAY"
      n115 = property on="wprot stat" class="Clust (strict)"("Visible"=w231) -> ()  [unwired: 2 in, 2 out]
      n116 = property on="wpsel stat" class="Clust (strict)"("Visible"=w231) -> ()  [unwired: 2 in, 2 out]
      n117 = property on="GFOC Value" class="DigNum (strict)"("Visible"=w230) -> ()  [unwired: 2 in, 2 out]
      n118 = property on="WPROT Value" class="DigNum (strict)"("Visible"=w230) -> ()  [unwired: 2 in, 2 out]
      n119 = property on="asel stat" class="Clust (strict)"("Visible"=w231) -> ()  [unwired: 2 in, 2 out]
      n120 = property on="calw stat" class="Clust (strict)"("Visible"=w231) -> ()  [unwired: 2 in, 2 out]
      n121 = property on="GMIR Value" class="DigNum (strict)"("Visible"=w230) -> ()  [unwired: 2 in, 2 out]
      n122 = property on="WPSEL Value" class="DigNum (strict)"("Visible"=w230) -> ()  [unwired: 2 in, 2 out]
      n123 = property on="gmir stat" class="Clust (strict)"("Visible"=w231) -> ()  [unwired: 2 in, 2 out]
      n124 = property on="gfoc stat" class="Clust (strict)"("Visible"=w231) -> ()  [unwired: 2 in, 2 out]
      n125 = property on="CALW Value" class="DigNum (strict)"("Visible"=w230) -> ()  [unwired: 2 in, 2 out]
      n126 = property on="ASEL Value" class="DigNum (strict)"("Visible"=w230) -> ()  [unwired: 2 in, 2 out]
    }
    frame #14 {
      # "PELA URGÊNCIA, OS PARÂMETROS DE PUB 0MQ\nFORAM  INSERIDOS  NA CLASSE MESSENGER."
      # "CREATE THE QUEUED COMMUNICATION OBJECTS"
      n127 = call-dynamic "Create messenger.vi"("InterComm path"=path "InterComm.vi", "0mqComm path"=path "0mqComm.vi" ("InterComm path"), "error in (no error)"=w240, "S4statusQueueName"="S4status", "S4commandQueueName"="S4command", "Messenger in"=refnum<class "Messenger.lvclass"> refnum) -> ("error out"=w236:errorcluster, "Messenger out"=w233:refnum<class "Messenger.lvclass">)  [unwired: 4 in]
      n128 = call-dynamic "Create queues.vi"("error in (no error)"=w236, "timeout"=500, "Messenger in"=w233) -> ("error out"=w235:errorcluster, "Messenger out"=w234:refnum<class "Messenger.lvclass">)  [unwired: 7 in]
    }
  }
  "cfgFile" <- w27
  n129 = flat-sequence {
    tunnel: w9 -> [w245]
    frame #0 {
      n130 = case shown="True" "runMinimized" {
        tunnel: w245 -> [_ w247]
        tunnel: T13."Minimized" ("Front Panel Window:State") -> [_ w246]
        frame False {
        }
        frame True {
          n131 = property class="VI"(error in=w247, "Front Panel Window:State"=w246) -> ()  [unwired: 1 in, 2 out]
        }
      }
    }
  }
  n132 = call "Create ICS.vi"("Messenger"=w14, "error in (no error)"=w15, "motors"=w25, "control indices"=w26, "email settings"=w24) -> ("error out"=w29:errorcluster, "ICS out"=w16:refnum<class "ICS.lvclass">)  [unwired: 5 in]
  n133 = Create User Event(user event datatype=w12) -> (user event=w11:refnum<user-event>)  [unwired: 1 in, 1 out]
  n134 = call <vilib>:"Application Directory.vi"() -> ("Application Directory"=w23:path)
  n135 = Get Control Values by Index(1:w26, 3:w29) -> (10:w18:variant[], 11:w22:errorcluster)  [unwired: 1 in]
  n136 = Build Path(base path=w23, name or relative path=w27) -> (appended path=w20:path)
  n137 = register-events(w11) -> (reference out=w8:refnum<event-registration>)  [unwired: 2 in, 1 out]
  n138 = call "Config file.vi"("path"=w20, "access (0:read/write)"=enum16{"read/write", "read-only", "write-only"}."read-only", "error in (no error)"=w22, "data values"=w18, "email settings"=w24) -> ("error out"=w21:errorcluster, "data out"=w17:variant[])  [unwired: 5 in]
  n139 = Set Control Values by Index(1:w26, 2:w17, 3:w21) -> (11:w9:errorcluster)  [unwired: 1 in]
  n140 = while {
    shift-right: [w258] -> w30
    shift-left: w16 -> [w261]
    shift-right: [w257] -> w10
    shift-left: w9 -> [w262]
    shift-right: [w259] -> _
    shift-left: 0 -> [w260]
    tunnel: w8 -> [w255]
    tunnel: w11 -> [w254]
    tunnel: w8 -> [w253]
    stop <- w248 stop-if-true
    # "PUB\nZEROMQ"
    # "AQUI DEVE SER PUBLICANDO O STATUS DO S4ICS\nCASO ELE TENHA SIDO ALTERADO.\n\nO VI 0mqComm SE ENCARREGA DE \nPUBLICAR O STATUS PERIODICAMENTE"
    n141 = event shown="[0] Timeout" {
      selector: w255 -> [_ _ _ _ _ _ _ _ _ _ _ _ _ _ _ _ _ _ _ _ _ _ _ _ _ _ _ _ _ _ _ _ _ _ _ _ _ _]
      dyn-events: _ -> [_ _ _ _ _ _ _ _ _ _ _ _ _ _ _ _ _ _ _ _ _ _ _ _ _ _ _ _ _ _ _ _ _ _ _ _ _ _]
      timeout: 20 -> [_ _ _ _ _ _ _ _ _ _ _ _ _ _ _ _ _ _ _ _ _ _ _ _ _ _ _ _ _ _ _ _ _ _ _ _ _ _]
      tunnel: w261 -> [w391 w1628 w1686 w1697 w1699 w1774 w1782 w1823 w1898 w2063 w2089 w2093 w2097 w2102 w2131 w2194 w2256 w2258 w2259 w2262 w2264 w2266 w2267 w2276 w2285 w2303 w2351 w2393 w2436 w2452 w2458 w2480 w2495 w2506 w2523 w2556 w2605 w2628]
      tunnel: w262 -> [w401 w1627 w1685 w1696 w1698 w1773 w1781 w1822 w1897 w2062 w2088 w2092 w2098 w2101 w2132 w2195 w2255 w2257 w2260 w2261 w2263 w2265 w2268 w2275 w2284 w2304 w2352 w2392 w2433 w2451 w2457 w2468 w2494 w2505 w2524 w2553 w2602 w2629]
      tunnel: [w398 w1627 w1685 w1696 w1716 w1773 w1781 w1807 w1916 w2061 w2077 w2092 w2096 w2101 w2122 w2192 w2255 w2257 w2260 w2261 w2263 w2265 w2268 w2275 w2284 w2305 w2350 w2392 w2435 w2451 w2457 w2474 w2494 w2504 w2527 w2552 w2601 w2626] -> w251
      tunnel: [w397 w1628 w1686 w1697 w1717 w1774 w1782 w1806 w1917 w2060 w2076 w2093 w2095 w2102 w2129 w2193 w2256 w2258 w2259 w2262 w2264 w2266 w2267 w2276 w2285 w2301 w2348 w2393 w2434 w2452 w2458 w2473 w2495 w2503 w2521 w2556 w2605 w2627] -> w252
      tunnel: w260 -> [w394 _ _ _ _ _ _ _ _ _ _ _ _ _ _ _ _ _ _ _ _ _ _ _ _ _ _ _ _ _ _ _ _ _ _ _ _ _]
      tunnel: [w393 _ _ _ _ _ _ _ _ _ _ _ _ _ _ _ _ _ _ _ _ _ _ _ _ _ _ _ _ _ _ _ _ _ _ _ _ _] -> w259
      tunnel: w254 -> [w390 _ _ _ _ _ _ _ _ _ _ _ _ _ _ _ _ _ _ _ _ _ _ _ _ _ _ _ _ _ _ _ _ _ _ _ _ _]
      tunnel: w253 -> [w389 _ _ _ _ _ _ _ _ _ _ _ _ _ _ _ _ _ _ _ _ _ _ _ _ _ _ _ _ _ _ _ _ _ _ _ _ _]
      tunnel: [_ _ _ _ _ _ _ _ FALSE TRUE TRUE _ _ _ _ _ _ _ _ _ _ _ _ _ _ _ _ _ _ _ _ _ _ _ _ _ _ _] -> w248
      event Timeout {
        # "CHECK FOR SERVER ENABLE"
        n142 = event-data() -> ()  [unwired: 1 in, 3 out]
        n143 = local read "server"() -> (w396:bool)
        n144 = call-dynamic "Check moving.vi"("error in (no error)"=w401, "ICS in"=w391) -> ("error out"=w400:errorcluster, "in motion"=w392:bool, "ICS out"=w399:refnum<class "ICS.lvclass">)  [unwired: 7 in]
        n145 = Or(x=w392, y=w396) -> (x .or. y?=w395:bool)
        n146 = case shown="False" w395 {
          tunnel: w400 -> [w406 w459]
          tunnel: w399 -> [w407 w457]
          tunnel: [w403 w461] -> w398
          tunnel: [w402 w460] -> w397
          tunnel: w394 -> [w420 _]
          tunnel: [w417 _] -> w393
          tunnel: w390 -> [w412 _]
          tunnel: w389 -> [w408 w446]
          frame False {
            # "READ AND DISCARD 0MQ PULL MESSAGES"
            # "CHECK FOR AUTOMATIC LOGOUT"
            n147 = First Call?() -> (First Call?: T/F=w411:bool)
            n148 = call-dynamic "Read Messenger.vi"("error in (no error)"=w406, "ICS in"=w407) -> ("error out"=w404:errorcluster, "Messenger.lvclass"=w405:refnum<class "Messenger.lvclass">, "ICS out"=w402:refnum<class "ICS.lvclass">)  [unwired: 7 in]
            n149 = And(x=w411, y="autoSS") -> (x .and. y?=w409:bool)
            n150 = case shown="True" w409 {
              selector: w409 -> [_ w422]
              tunnel: w412 -> [_ w427]
              tunnel: w408 -> [_ _]
              frame False {
              }
              frame True {
                w426 = T12."Disabled and Grayed Out" ("Disabled")
                n151 = Generate User Event(user event=w427, event data cluster=w422) -> (user event out=w421:refnum<user-event>)  [unwired: 2 in, 1 out]
                n152 = Destroy User Event(user event=w421) -> ()  [unwired: 1 in, 1 out]
                n153 = property on="assist" class="Bool"("DisabledEnum"=w426) -> ()  [unwired: 2 in, 2 out]
                n154 = property on="setup" class="Bool"("DisabledEnum"=w426) -> ()  [unwired: 2 in, 2 out]
                n155 = property on="control" class="Bool"("DisabledEnum"=w426) -> ()  [unwired: 2 in, 2 out]
                n156 = property on="start server" class="Bool"("DisabledEnum"=T12."Enabled" ("Disabled")) -> ()  [unwired: 2 in, 2 out]
                n157 = local write "tab menu"(T6."Stopped" ("tab menu")) -> ()
                n158 = local write "tab body"(enum32{"Motors", "Config"}."Motors" ("tab body")) -> ()
              }
            }
            n159 = call-dynamic "Get command.vi"("error in (no error)"=w404, "Messenger in"=w405) -> ("error out"=w403:errorcluster)  [unwired: 6 in, 3 out]
            n160 = local read "tab menu"() -> (w418:T6)
            n161 = Multiply(x="auto logout", y=1000 ("f")) -> (x*y=w413:u32)
            n162 = Not Equal?(x=w418, y=T15."Login" ("tab menu")) -> (x != y?=w416:bool)
            n163 = case shown="True" w416 {
              tunnel: w420 -> [_ w431]
              tunnel: [0 w432] -> w417
              tunnel: w413 -> [_ w429]
              frame False {
              }
              frame True {
                n164 = Greater?(x=w431, y=w429) -> (0:w430:bool)
                n165 = case shown="True" w430 {
                  tunnel: w431 -> [w435 _]
                  tunnel: [w433 0] -> w432
                  frame False {
                    # "KEEP COUNTING"
                    n166 = Add(x=w435, y=5) -> (x+y=w433:i32)
                  }
                  frame True {
                    w441 = ""
                    # "LOGOUT"
                    n167 = local write "tab menu"(T6."Login" ("tab menu")) -> ()
                    n168 = local write "tab body"(enum32{"Motors", "Config"}."Motors" ("tab body")) -> ()
                    n169 = local write "loginPW"(w441) -> ()
                    n170 = local write "loginUser"(w441) -> ()
                    n171 = local read "server"() -> (w436:bool)
                    n172 = Not(x=w436) -> (.not. x?=w442:bool)
                    n173 = property on="exitLogin" class="Bool"("Visible"=w442) -> ()  [unwired: 2 in, 2 out]
                    n174 = property on="loginUser" class="Str"("Key Focus"=TRUE) -> ()  [unwired: 2 in, 2 out]
                  }
                }
              }
            }
          }
          frame True {
            # "CHECK FOR INCOMMING MESSAGES FROM CLIENTS"
            n175 = local read "channel"() -> (w456:T5)
            n176 = call-dynamic "Read motors.vi"("ICS in"=w457) -> ("motors"=w454:refnum<class "Motor.lvclass">[])  [unwired: 8 in, 2 out]
            n177 = First Call?() -> (First Call?: T/F=w445:bool)
            n178 = Equal?(x=w456, y=T5."Inner TCP/IP" ("channel")) -> (x = y?=w444:bool)
            n179 = case shown="True" w444 {
              tunnel: w459 -> [w479 w498]
              tunnel: [w478 w497] -> w458
              tunnel: w457 -> [w477 w499]
              tunnel: [w476 w496] -> w449
              tunnel: [w475 w495] -> w447
              tunnel: [w474 w494] -> w453
              tunnel: [FALSE w493] -> w443
              frame False {
                # "READ CLIENT COMMAND\nUSING INTERCOMM VI"
                n180 = disable-structure shown="Enabled" {
                  disable-tunnel: w479 -> [w490 w492]
                  disable-tunnel: [w483 w491] -> w478
                  disable-tunnel: w477 -> [w489 w491]
                  disable-tunnel: [w488 _] -> w476
                  disable-tunnel: [w487 _] -> w475
                  disable-tunnel: [w480 w492] -> w474
                  frame Enabled {
                    n181 = call-dynamic "Read Messenger.vi"("error in (no error)"=w490, "ICS in"=w489) -> ("error out"=w486:errorcluster, "Messenger.lvclass"=w485:refnum<class "Messenger.lvclass">, "ICS out"=w484:refnum<class "ICS.lvclass">)  [unwired: 7 in]
                    n182 = call-dynamic "Get command.vi"("error in (no error)"=w486, "Messenger in"=w485) -> ("error out"=w481:errorcluster, "isAcommand"=w487:bool, "command"=w488:string, "Messenger out"=w482:refnum<class "Messenger.lvclass">)  [unwired: 6 in]
                    n183 = call-dynamic "Write Messenger.vi"("error in (no error)"=w481, "Messenger.lvclass"=w482, "ICS in"=w484) -> ("error out"=w480:errorcluster, "ICS out"=w483:refnum<class "ICS.lvclass">)  [unwired: 7 in]
                  }
                  frame Disabled {
                  }
                }
              }
              frame True {
                # "READ CLIENT COMMAND\nUSING INNER TCP/IP CONNECTION\nAND/OR ZEROMQ PULL"
                n184 = disable-structure shown="Enabled" {
                  disable-tunnel: w499 -> [w510 w525]
                  disable-tunnel: w498 -> [w509 w526]
                  disable-tunnel: [w506 w524] -> w497
                  disable-tunnel: [w502 w523] -> w496
                  disable-tunnel: [w501 w522] -> w495
                  disable-tunnel: [w500 w527] -> w494
                  disable-tunnel: [_ w521] -> w493
                  frame Disabled {
                    n185 = call "Read Server.vi"("error in (no error)"=w509, "ICS in"=w510) -> ("error out"=w508:errorcluster, "Server"=w511:refnum<class "TCP-Server.lvclass">, "ICS out"=w507:refnum<class "ICS.lvclass">)  [unwired: 7 in]
                    n186 = call-dynamic "Wait on listenner.vi"("error in (no error)"=w508, "Server in"=w511) -> ("error out"=w504:errorcluster, "Server out"=w505:refnum<class "TCP-Server.lvclass">)  [unwired: 8 in]
                    n187 = call "Write Server.vi"("error in (no error)"=w504, "Server"=w505, "ICS in"=w507) -> ("error out"=w503:errorcluster, "ICS out"=w506:refnum<class "ICS.lvclass">)  [unwired: 7 in]
                    n188 = case shown="Error" w503 {
                      selector: w503 -> [w516 w519]
                      tunnel: w505 -> [w512 _]
                      tunnel: [w515 w518] -> w500
                      tunnel: [w513 FALSE] -> w501
                      tunnel: [w514 _] -> w502
                      frame No Error {
                        n189 = call-dynamic "Receive message.vi"("error in (no error)"=w516, "Server in"=w512) -> ("error out"=w515:errorcluster, "isAcommand"=w513:bool, "message"=w514:string)  [unwired: 6 in, 1 out]
                      }
                      frame Error {
                        n190 = call <vilib>:"Clear Errors.vi"("error in (no error)"=w519, "specific error code to clear (0: all)"=56) -> ("error out"=w518:errorcluster)  [unwired: 4 in, 1 out]
                      }
                    }
                  }
                  frame Enabled {
                    n191 = call-dynamic "Read 0mq-Tcp command.vi"("error in (no error)"=w526, "ICS in"=w525) -> ("error out"=w527:errorcluster, "isAcommand"=w522:bool, "command"=w523:string, "ICS out"=w524:refnum<class "ICS.lvclass">, "rec0mq"=w521:bool)  [unwired: 5 in]
                  }
                }
              }
            }
            n192 = for {
              tunnel: w454 -> [w464] mode=indexing
              # "UPDATE STATUS DISPLAY"
              n193 = call-dynamic "Read status.vi"("Motor in"=w464) -> ("name"=w466:string, "status"=w465:T1)  [unwired: 7 in, 2 out]
              n194 = case shown="\"ASEL\"" w466 {
                tunnel: w465 -> [w467 w468 w469 w470 w471 w472]
                frame "Default", Default {
                  "gfoc stat" <- w467
                }
                frame "WPROT" {
                  "wprot stat" <- w468
                }
                frame "WPSEL" {
                  "wpsel stat" <- w469
                }
                frame "ASEL" {
                  "asel stat" <- w470
                }
                frame "CALW" {
                  "calw stat" <- w471
                }
                frame "GMIR" {
                  "gmir stat" <- w472
                }
              }
            }
            n195 = case shown="True" w445 {
              tunnel: w446 -> [_ w463]
              frame False {
              }
              frame True {
                n196 = Unregister For Events(event registration refnum=w463) -> (error out=w462:errorcluster)  [unwired: 1 in]
                n197 = call <vilib>:"Clear Errors.vi"("error in (no error)"=w462) -> ()  [unwired: 5 in, 2 out]
              }
            }
            n198 = call "Check message.vi"("error in (no error)"=w453, "isAcommand"=w447, "message in"=w449) -> ("error out"=w452:errorcluster, "valid"=w451:bool, "message"=w450:string, "not empty"=w448:bool)  [unwired: 5 in]
            n199 = case shown="True" w451 {
              tunnel: [w529 w1492] -> w461
              tunnel: w458 -> [w535 w1499]
              tunnel: [w530 w1493] -> w460
              tunnel: w450 -> [_ w1473]
              tunnel: w452 -> [w528 w1500]
              tunnel: w448 -> [_ w1495]
              tunnel: w444 -> [_ w1461]
              tunnel: w443 -> [_ w1460]
              frame False {
                # "NO CLIENT CONNECTION: TAKE CARE OF MECHANISMS"
                n200 = call-dynamic "Select motor.vi"("error in (no error)"=w528, "ICS in"=w535) -> ("error out"=w531:errorcluster, "valid"=w534:bool, "selected motor"=w533:refnum<class "Motor.lvclass">, "ICS out"=w532:refnum<class "ICS.lvclass">)  [unwired: 6 in]
                n201 = case shown="True" w534 {
                  tunnel: w533 -> [_ w613]
                  tunnel: [w537 w601] -> w529
                  tunnel: w532 -> [w538 w593]
                  tunnel: w531 -> [w539 w612]
                  tunnel: [w536 w604] -> w530
                  frame False {
                    # "NO MOTOR SELECTED, GET UPDATED MOTOR INFORMATION"
                    n202 = disable-structure shown="Disabled" {
                      disable-tunnel: w539 -> [w559 w590]
                      disable-tunnel: w538 -> [w558 w589]
                      disable-tunnel: [w542 w590] -> w537
                      disable-tunnel: [w541 w589] -> w536
                      frame Disabled {
                        # "DEPOIS DE TESTAR O FUNCIONAMENTO,\nCRIAR UM VI PARA SELECIONAR UM MOTOR\nQUE ESTEJA HABILITADO E NO MODO CONTROL"
                        n203 = call-dynamic "Read motors.vi"("error in (no error)"=w559, "ICS in"=w558) -> ("error out"=w556:errorcluster, "motors"=w543:refnum<class "Motor.lvclass">[], "ICS out"=w557:refnum<class "ICS.lvclass">)  [unwired: 7 in]
                        n204 = call-dynamic "Read MotorManager.vi"("error in (no error)"=w556, "ICS in"=w557) -> ("error out"=w561:errorcluster, "MotorManager.lvclass"=w560:refnum<class "MotorManager.lvclass">, "ICS out"=w544:refnum<class "ICS.lvclass">)  [unwired: 7 in]
                        n205 = Build Array("GS0", "V31") -> (w551:string[])
                        n206 = call-dynamic "Read current state.vi"("error in (no error)"=w561, "StateManager in"=w560) -> ("error out"=w555:errorcluster, "currentState"=w545:u32, "StateManager out"=w546:refnum<class "MotorManager.lvclass">)  [unwired: 7 in]
                        n207 = Index Array(array=w543, index=w545) -> (element=w554:refnum<class "Motor.lvclass">)
                        n208 = Wait (ms)(milliseconds to wait=u32 50) -> ()  [unwired: 1 out]
                        n209 = call-dynamic "Send instructions.vi"("error in (no error)"=w555, "instructions"=w551, "Motor in"=w554) -> ("error out"=w548:errorcluster, "error"=w549:bool, "replies"=w550:string[], "Motor out"=w547:refnum<class "Motor.lvclass">)  [unwired: 4 in, 1 out]
                        n210 = case shown="False" w549 {
                          tunnel: w550 -> [w586 _]
                          tunnel: w548 -> [w585 w588]
                          tunnel: w547 -> [w584 _]
                          tunnel: w546 -> [w567 _]
                          tunnel: w545 -> [w574 _]
                          tunnel: w544 -> [w570 w587]
                          tunnel: w543 -> [w575 _]
                          tunnel: [w563 w588] -> w542
                          tunnel: [w562 w587] -> w541
                          frame False {
                            # "STORE MOTOR INFO AND SELECT ANOTHER MOTOR FOR NEXT READING"
                            n211 = Increment(x=w574) -> (x+1=w577:u32)
                            n212 = Index Array(array=w586, index=1) -> (element=w583:string)
                            n213 = Decimal String To Number(string=w583, default (0L)=u32 0 ("default (0 I32)")) -> (number=w582:u32)  [unwired: 1 in, 1 out]
                            n214 = Greater Or Equal?(x=w577, y=u32 5) -> (x >= y?=w578:bool)
                            n215 = call-dynamic "Write motor info.vi"("error in (no error)"=w585, "motor info"=w582, "Motor in"=w584) -> ("error out"=w572:errorcluster, "Motor out"=w573:refnum<class "Motor.lvclass">)  [unwired: 7 in]
                            n216 = Select(t=u32 0 ("y"), s=w578, f=w577) -> (s? t:f=w568:u32)
                            n217 = Replace Array Subset(array=w575, new element=w573, index=w574) -> (w571:refnum<class "Motor.lvclass">[])
                            n218 = call-dynamic "Write motors.vi"("error in (no error)"=w572, "motors"=w571, "ICS in"=w570) -> ("error out"=w569:errorcluster, "ICS out"=w565:refnum<class "ICS.lvclass">)  [unwired: 7 in]
                            n219 = call-dynamic "Write current state.vi"("error in (no error)"=w569, "currentState"=w568, "StateManager in"=w567) -> ("error out"=w566:errorcluster, "StateManager out"=w564:refnum<class "MotorManager.lvclass">)  [unwired: 7 in]
                            n220 = call-dynamic "Write MotorManager.vi"("error in (no error)"=w566, "MotorManager.lvclass"=w564, "ICS in"=w565) -> ("error out"=w563:errorcluster, "ICS out"=w562:refnum<class "ICS.lvclass">)  [unwired: 7 in]
                          }
                          frame True {
                            # "NO RESPONSE FROM MOTOR"
                          }
                        }
                      }
                      frame Enabled {
                      }
                    }
                  }
                  frame True {
                    # "PROCESS SELECTED MOTOR"
                    n221 = call-dynamic "Read StateManager.vi"("error in (no error)"=w612, "Motor in"=w613) -> ("error out"=w610:errorcluster, "StateManager"=w611:refnum<class "StateManager.lvclass">, "Motor out"=w598:refnum<class "Motor.lvclass">, "stateEnum"=w607:T16)  [unwired: 5 in, 1 out]
                    n222 = call-dynamic "Read current state.vi"("error in (no error)"=w610, "StateManager in"=w611) -> ("error out"=w609:errorcluster, "currentState"=w608:u32, "StateManager out"=w592:refnum<class "StateManager.lvclass">)  [unwired: 7 in]
                    n223 = Variant To Data(error in=w609, type=w607, Variant=w608) -> (data=w600:T16, error out=w599:errorcluster)
                    n224 = case shown="\"Wait\", Default" w600 {
                      tunnel: w599 -> [w617 w671 w724 w787 w817 w911 w979 w1062 w1110 w1215 w1286 w1336 w1389]
                      tunnel: w598 -> [w619 w670 w725 w788 w818 w910 w978 w1061 w1109 w1214 w1287 w1337 w1390]
                      tunnel: [w620 w678 w734 w790 w811 w882 w974 w1057 w1103 w1193 w1289 w1340 w1375] -> w597
                      tunnel: [w615 w674 w729 w784 w803 w881 w975 w1059 w1107 w1212 w1271 w1330 w1391] -> w596
                      tunnel: [w618 w677 w733 w789 w810 w909 w973 w1056 w1102 w1211 w1288 w1339 w1374] -> w595
                      tunnel: [w616 w675 w730 w781 w804 w877 w976 w1060 w1108 w1213 w1270 w1329 w1373] -> w594
                      tunnel: w593 -> [w620 w678 w734 w790 w811 w899 w974 w1057 w1103 w1194 w1289 w1340 w1375]
                      tunnel: w592 -> [w618 w677 w733 w789 w810 w909 w973 w1056 w1102 w1211 w1288 w1339 w1374]
                      tunnel: [w614 w673 w728 T16."ActiveFinish" ("stateEnum") w802 T16."Wait" ("stateEnum") T16."SimUptate" ("stateEnum") T16."SimUptate" ("stateEnum") w1106 T16."Wait" ("stateEnum") w1290 w1318 w1371] -> w591
                      frame "Wait", Default {
                        # "CHECK FOR RECEIVED COMMAND (ACK = TRUE) - MOTOR STATE MACHINE"
                        n225 = call-dynamic "Read ack flag.vi"("error in (no error)"=w617, "Motor in"=w619) -> ("error out"=w626:errorcluster, "ack"=w629:bool, "Motor out"=w627:refnum<class "Motor.lvclass">)  [unwired: 6 in, 1 out]
                        n226 = call "Read mode.vi"("error in (no error)"=w626, "Motor in"=w627) -> ("error out"=w624:errorcluster, "mode"=w628:string, "Motor out"=w625:refnum<class "Motor.lvclass">)  [unwired: 7 in]
                        n227 = call-dynamic "Read action-param.vi"("error in (no error)"=w624, "Motor in"=w625) -> ("error out"=w621:errorcluster, "action"=w623:string, "Motor out"=w622:refnum<class "Motor.lvclass">)  [unwired: 6 in, 1 out]
                        n228 = case shown="True" w629 {
                          tunnel: w628 -> [_ w641]
                          tunnel: w623 -> [_ w640]
                          tunnel: [T16."Wait" ("stateEnum") w634] -> w614
                          tunnel: w622 -> [w631 w638]
                          tunnel: w621 -> [w632 w637]
                          tunnel: [w631 w636] -> w615
                          tunnel: [w632 w635] -> w616
                          frame False {
                            # "NO COMMAND WAS RECEIVED"
                          }
                          frame True {
                            # "COMMAND RECEIVED, SET NEXT STATE"
                            n229 = case shown="\"SIMULATED\"" w641 {
                              tunnel: w640 -> [_ w650 w657]
                              tunnel: [T16."Wait" ("stateEnum") w649 w656] -> w634
                              frame "NONE", Default {
                              }
                              frame "ACTIVE" {
                                n230 = case shown="\"NONE\", Default" w650 {
                                tunnel: [T16."ActiveInit" ("stateEnum") T16."ActiveGoto" ("stateEnum") T16."CyclicStart" ("stateEnum") T16."ActiveStop" ("stateEnum") T16."Wait" ("stateEnum")] -> w649
                                frame "INIT" {
                                }
                                frame "GOTO" {
                                }
                                frame "CYCLIC" {
                                }
                                frame "STOP" {
                                }
                                frame "NONE", Default {
                                }
                                }
                              }
                              frame "SIMULATED" {
                                n231 = case shown="\"NONE\", Default" w657 {
                                tunnel: [T16."SimInit" ("stateEnum") T16."SimGoto" ("stateEnum") T16."SimFinish" ("stateEnum") T16."Wait" ("stateEnum")] -> w656
                                frame "INIT" {
                                }
                                frame "GOTO" {
                                }
                                frame "STOP" {
                                }
                                frame "NONE", Default {
                                }
                                }
                              }
                            }
                            n232 = Equal?(x=T16."Wait" ("stateEnum"), y=w634) -> (x = y?=w639:bool)
                            n233 = case shown="True" w639 {
                              tunnel: w638 -> [w643 w647]
                              tunnel: w637 -> [w642 w646]
                              tunnel: [w642 w645] -> w635
                              tunnel: [w643 w644] -> w636
                              frame False {
                              }
                              frame True {
                                n234 = call-dynamic "Clear ack flag.vi"("error in (no error)"=w646, "Motor in"=w647) -> ("error out"=w645:errorcluster, "Motor out"=w644:refnum<class "Motor.lvclass">)  [unwired: 8 in]
                              }
                            }
                          }
                        }
                      }
                      frame "ActiveInit" {
                        # "SEND INIT INSTRUCTIONS TO MOTOR"
                        n235 = call-dynamic "Get init instructions.vi"("error in (no error)"=w671, "Motor in"=w670) -> ("error out"=w672:errorcluster, "name"=w664:string, "init instructions"=w665:string[], "Motor out"=w669:refnum<class "Motor.lvclass">)  [unwired: 6 in]
                        n236 = local read "enabled log"() -> (w663:string)
                        n237 = call-dynamic "Send and log instructions.vi"("prefix"=w664, "current code"="2" ("current priority"), "enabled codes"=w663, "error in (no error)"=w672, "instructions"=w665, "Motor in"=w669) -> ("error out"=w667:errorcluster, "replies"=w666:string[], "Motor out"=w668:refnum<class "Motor.lvclass">, "ok"=w676:bool)  [unwired: 1 in, 1 out]
                        n238 = case shown="True" w676 {
                          tunnel: w667 -> [w687 w711]
                          tunnel: w668 -> [w688 w710]
                          tunnel: [w699 w705] -> w674
                          tunnel: [w698 w707] -> w675
                          tunnel: [T16."Wait" ("stateEnum") T16."ActiveUpdate" ("stateEnum")] -> w673
                          tunnel: w666 -> [w684 _]
                          tunnel: w665 -> [w683 _]
                          tunnel: w663 -> [w682 _]
                          frame False {
                            w681 = "TIMEOUT" ("x")
                            w694 = ""
                            # "ERROR: CLEAR ACK FLAG IN ORDER TO ENABLE COMMANDS"
                            n239 = call-dynamic "Read name.vi"("error in (no error)"=w687, "Motor in"=w688) -> ("error out"=w693:errorcluster, "name"=w690:string, "Motor out"=w685:refnum<class "Motor.lvclass">)  [unwired: 7 in]
                            n240 = Concatenate Strings("ActiveInit ", w690, ": ", w681) -> (w689:string)
                            n241 = call "Write log to file.vi"("current priority"="2", "enabled priority"=w682, "error in"=w693, "resp array"=w684, "send array"=w683, "prefix"=w689) -> ("error out"=w686:errorcluster)  [unwired: 3 in, 2 out]
                            n242 = Bundle By Name(cluster=T1 {"mode"="", "condition"="", "position"="", "pos_name"="", "pos_id"=""} ("status"), "mode"=w694, "condition"=w681, "position"=w694, "pos_name"=w694, "pos_id"=w694) -> (w695:T1)
                            n243 = call-dynamic "Write command in.vi"("error in (no error)"=w686, "command in"=T17 {"action"="", "param"="", "pos_name"="", "pos_idx"=0, "ack"=FALSE, "stop"=FALSE, "offset"=FALSE, "immediate"=FALSE, "instructions"=[]}, "Motor in"=w685) -> ("error out"=w696:errorcluster, "Motor out"=w697:refnum<class "Motor.lvclass">)  [unwired: 7 in]
                            n244 = call-dynamic "Write status.vi"("hold if empty"=TRUE, "error in (no error)"=w696, "status"=w695, "Motor in"=w697) -> ("error out"=w698:errorcluster, "Motor out"=w699:refnum<class "Motor.lvclass">)  [unwired: 6 in]
                          }
                          frame True {
                            w713 = ""
                            # "MOTOR RECEIVED INSTRUCTIONS: SET BUSY CONDITION"
                            n245 = Bundle By Name(cluster=T1 {"mode"="", "condition"="", "position"="", "pos_name"="", "pos_id"=""} ("status"), "mode"=w713, "condition"="BUSY" ("string"), "position"=w713, "pos_name"="NONE", "pos_id"="-1") -> (w714:T1)
                            n246 = call-dynamic "Write status.vi"("hold if empty"=TRUE, "error in (no error)"=w711, "status"=w714, "Motor in"=w710) -> ("error out"=w708:errorcluster, "Motor out"=w706:refnum<class "Motor.lvclass">)  [unwired: 6 in]
                            n247 = call-dynamic "Write moving flag.vi"("error in (no error)"=w708, "moving"=TRUE, "Motor in"=w706) -> ("error out"=w707:errorcluster, "Motor out"=w705:refnum<class "Motor.lvclass">)  [unwired: 7 in]
                          }
                        }
                      }
                      frame "ActiveGoto" {
                        # "SEND GOTO INSTRUCTIONS TO MOTOR"
                        n248 = call-dynamic "Get goto instructions.vi"("error in (no error)"=w724, "Motor in"=w725) -> ("error out"=w726:errorcluster, "name"=w719:string, "goto instructions"=w721:string[], "Motor out"=w727:refnum<class "Motor.lvclass">)  [unwired: 6 in]
                        n249 = local read "enabled log"() -> (w718:string)
                        n250 = call-dynamic "Send and log instructions.vi"("prefix"=w719, "current code"="2" ("current priority"), "enabled codes"=w718, "error in (no error)"=w726, "instructions"=w721, "Motor in"=w727) -> ("error out"=w723:errorcluster, "replies"=w722:string[], "Motor out"=w731:refnum<class "Motor.lvclass">, "ok"=w732:bool)  [unwired: 1 in, 1 out]
                        n251 = case shown="False" w732 {
                          tunnel: w723 -> [w749 w760]
                          tunnel: w731 -> [w748 w761]
                          tunnel: [w751 w765] -> w729
                          tunnel: [w750 w764] -> w730
                          tunnel: [T16."Wait" ("stateEnum") T16."ActiveUpdate" ("stateEnum")] -> w728
                          tunnel: w718 -> [w744 _]
                          tunnel: w722 -> [w742 _]
                          tunnel: w721 -> [w741 _]
                          frame False {
                            w736 = "TIMEOUT" ("x")
                            w753 = ""
                            # "ERROR: CLEAR ACK FLAG IN ORDER TO ENABLE COMMANDS"
                            n252 = call-dynamic "Read name.vi"("error in (no error)"=w749, "Motor in"=w748) -> ("error out"=w746:errorcluster, "name"=w739:string, "Motor out"=w747:refnum<class "Motor.lvclass">)  [unwired: 7 in]
                            n253 = Concatenate Strings("ActiveGoto ", w739, ": ", w736) -> (w738:string)
                            n254 = call "Write log to file.vi"("current priority"="0", "enabled priority"=w744, "error in"=w746, "resp array"=w742, "send array"=w741, "prefix"=w738) -> ("error out"=w745:errorcluster)  [unwired: 3 in, 2 out]
                            n255 = Bundle By Name(cluster=T1 {"mode"="", "condition"="", "position"="", "pos_name"="", "pos_id"=""} ("status"), "mode"=w753, "condition"=w736, "position"=w753, "pos_name"=w753, "pos_id"=w753) -> (w754:T1)
                            n256 = call-dynamic "Write command in.vi"("error in (no error)"=w745, "command in"=T17 {"action"="", "param"="", "pos_name"="", "pos_idx"=0, "ack"=FALSE, "stop"=FALSE, "offset"=FALSE, "immediate"=FALSE, "instructions"=[]}, "Motor in"=w747) -> ("error out"=w755:errorcluster, "Motor out"=w756:refnum<class "Motor.lvclass">)  [unwired: 7 in]
                            n257 = call-dynamic "Write status.vi"("hold if empty"=TRUE, "error in (no error)"=w755, "status"=w754, "Motor in"=w756) -> ("error out"=w750:errorcluster, "Motor out"=w751:refnum<class "Motor.lvclass">)  [unwired: 6 in]
                          }
                          frame True {
                            w762 = TRUE ("hold if empty")
                            w768 = ""
                            # "MOTOR RECEIVED INSTRUCTIONS: SET BUSY CONDITION"
                            n258 = Bundle By Name(cluster=T1 {"mode"="", "condition"="", "position"="", "pos_name"="", "pos_id"=""} ("status"), "mode"=w768, "condition"="BUSY" ("string"), "position"=w768, "pos_name"="NONE", "pos_id"="-1") -> (w769:T1)
                            n259 = call-dynamic "Write status.vi"("hold if empty"=w762, "error in (no error)"=w760, "status"=w769, "Motor in"=w761) -> ("error out"=w763:errorcluster, "Motor out"=w766:refnum<class "Motor.lvclass">)  [unwired: 6 in]
                            n260 = call-dynamic "Write moving flag.vi"("error in (no error)"=w763, "moving"=w762, "Motor in"=w766) -> ("error out"=w764:errorcluster, "Motor out"=w765:refnum<class "Motor.lvclass">)  [unwired: 7 in]
                          }
                        }
                      }
                      frame "ActiveStop" {
                        n261 = call-dynamic "Read stop flag.vi"("error in (no error)"=w787, "Motor in"=w788) -> ("error out"=w777:errorcluster, "stop"=w786:bool, "Motor out"=w779:refnum<class "Motor.lvclass">)  [unwired: 7 in]
                        n262 = case shown="True" w786 {
                          tunnel: string[] ["STOP", "SR0=0"] ("instructions") -> [w793 w794]
                          tunnel: [w792 w794] -> w780
                          tunnel: "V46=251" -> [w791 _]
                          frame False {
                            # "STOP CMD WHILE\nMOTOR MOVING"
                            n263 = Insert Into Array(array=w793, new element=w791) -> (w792:string[])  [unwired: 1 in]
                          }
                          frame True {
                            # "STOP CMD WHILE\nMOTOR STATIC"
                          }
                        }
                        n264 = local read "enabled log"() -> (w774:string)
                        n265 = call-dynamic "Read name.vi"("error in (no error)"=w777, "Motor in"=w779) -> ("error out"=w776:errorcluster, "name"=w773:string, "Motor out"=w778:refnum<class "Motor.lvclass">)  [unwired: 7 in]
                        n266 = call-dynamic "Send and log instructions.vi"("prefix"=w773, "current code"="2" ("current priority"), "enabled codes"=w774, "error in (no error)"=w776, "instructions"=w780, "Motor in"=w778) -> ("error out"=w781:errorcluster, "Motor out"=w784:refnum<class "Motor.lvclass">)  [unwired: 1 in, 3 out]
                      }
                      frame "ActiveUpdate" {
                        n267 = call-dynamic "Get update instructions.vi"("error in (no error)"=w817, "only position"=FALSE, "Motor in"=w818) -> ("error out"=w813:errorcluster, "name"=w797:string, "read instructions"=w798:string[], "Motor out"=w812:refnum<class "Motor.lvclass">)  [unwired: 5 in]
                        n268 = local read "enabled log"() -> (w795:string)
                        n269 = call-dynamic "Send and log instructions.vi"("prefix"=w797, "current code"="5" ("current priority"), "enabled codes"=w795, "error in (no error)"=w813, "instructions"=w798, "Motor in"=w812) -> ("error out"=w814:errorcluster, "error"=w809:bool, "replies"=w816:string[], "Motor out"=w815:refnum<class "Motor.lvclass">)  [unwired: 1 in, 1 out]
                        n270 = case shown="False" w809 {
                          tunnel: w816 -> [w833 w864]
                          tunnel: w815 -> [w840 w867]
                          tunnel: w814 -> [w842 w863]
                          tunnel: [w847 w862] -> w808
                          tunnel: [w846 T16."ActiveUpdate" ("stateEnum")] -> w801
                          tunnel: [w843 w867] -> w800
                          tunnel: w798 -> [w832 w865]
                          tunnel: w797 -> [w831 w859]
                          tunnel: w795 -> [w827 _]
                          frame False {
                            # "PROCESS MOTOR RESPONSES"
                            n271 = Index Array(array=w833, index=1) -> (element=w841:string)
                            n272 = Index Array(array=w833, index=0) -> (element=w845:string)
                            n273 = call-dynamic "Encoder to mechanism position.vi"("error in (no error)"=w842, "motor position"=w841, "Motor in"=w840) -> ("error out"=w838:errorcluster, "mechanism position"=w830:string, "Motor out"=w839:refnum<class "Motor.lvclass">)  [unwired: 6 in]
                            n274 = call-dynamic "Write status position.vi"("error in (no error)"=w838, "status position"=w830, "Motor in"=w839) -> ("error out"=w851:errorcluster, "Motor out"=w850:refnum<class "Motor.lvclass">)  [unwired: 7 in]
                            n275 = Concatenate Strings(w831, "=" ("current priority"), w830) -> (w828:string)
                            n276 = call-dynamic "Track movement.vi"("error in (no error)"=w851, "tracking code"=w845, "Motor in"=w850) -> ("error out"=w847:errorcluster, "error"=w835:bool, "moving"=w844:bool, "Motor out"=w843:refnum<class "Motor.lvclass">)  [unwired: 5 in]
                            n277 = call "Write log to file.vi"("current priority"="5", "enabled priority"=w827, "prefix"=w828) -> ()  [unwired: 6 in, 3 out]
                            n278 = Select(t=T16."ActiveUpdate" ("stateEnum"), s=w844, f=T16."ActiveFinish" ("stateEnum")) -> (s? t:f=w846:T16)
                            n279 = case shown="False" w835 {
                              tunnel: w827 -> [_ w856]
                              tunnel: w831 -> [_ w855]
                              tunnel: w832 -> [_ w854]
                              tunnel: w833 -> [_ w853]
                              frame False {
                              }
                              frame True {
                                n280 = call "Write log to file.vi"("current priority"="0", "enabled priority"=w856, "resp array"=w853, "send array"=w854, "prefix"=w855) -> ()  [unwired: 4 in, 3 out]
                              }
                            }
                          }
                          frame True {
                            # "ERROR ON COMMUNICATION: TRY AGAIN"
                            n281 = local read "enabled log"() -> (w861:string)
                            n282 = Concatenate Strings("ActiveUpdate: ", w859) -> (w857:string)
                            n283 = call "Write log to file.vi"("current priority"="2", "enabled priority"=w861, "error in"=w863, "resp array"=w864, "send array"=w865, "prefix"=w857) -> ("error out"=w862:errorcluster)  [unwired: 3 in, 2 out]
                          }
                        }
                        n284 = call-dynamic "Read stop flag.vi"("error in (no error)"=w808, "Motor in"=w800) -> ("error out"=w805:errorcluster, "stop"=w807:bool, "Motor out"=w806:refnum<class "Motor.lvclass">)  [unwired: 7 in]
                        n285 = case shown="False" w807 {
                          tunnel: w806 -> [w821 w825]
                          tunnel: w805 -> [w820 w826]
                          tunnel: [w820 w824] -> w804
                          tunnel: [w821 w823] -> w803
                          tunnel: [w819 T16."ActiveStop" ("stateEnum")] -> w802
                          tunnel: w801 -> [w819 _]
                          frame False {
                          }
                          frame True {
                            n286 = call-dynamic "Clear stop flag.vi"("error in (no error)"=w826, "Motor in"=w825) -> ("error out"=w824:errorcluster, "Motor out"=w823:refnum<class "Motor.lvclass">)  [unwired: 8 in]
                          }
                        }
                      }
                      frame "ActiveFinish" {
                        w918 = ""
                        # "TODO O CASE DEDERIA SER UM VI DA CLASSE MOTOR"
                        n287 = call-dynamic "Read command in.vi"("error in (no error)"=w911, "Motor in"=w910) -> ("error out"=w874:errorcluster, "command in"=w920:T17, "Motor out"=w875:refnum<class "Motor.lvclass">)  [unwired: 6 in, 1 out]
                        n288 = call-dynamic "Read name.vi"("error in (no error)"=w874, "Motor in"=w875) -> ("error out"=w872:errorcluster, "name"=w889:string, "Motor out"=w873:refnum<class "Motor.lvclass">)  [unwired: 7 in]
                        n289 = call-dynamic "Read tracking code.vi"("error in (no error)"=w872, "Motor in"=w873) -> ("error out"=w870:errorcluster, "tracking code"=w871:string, "Motor out"=w868:refnum<class "Motor.lvclass">)  [unwired: 7 in]
                        n290 = Unbundle By Name(w920) -> ("action"=w907:string, "pos_name"=w897:string, "pos_idx"=w917:i32, "stop"=w919:bool)  [unwired: 2 out]
                        n291 = Equal?(x="INIT", y=w907) -> (x = y?=w905:bool)
                        n292 = Search and Replace String(input string=w897, search string="L/" ("replace string (\"\")")) -> (offset past replacement=w896:i32)  [unwired: 6 in, 3 out]
                        n293 = Equal?(x=w889, y="WPSEL" ("x")) -> (x = y?=w894:bool)
                        n294 = Greater Or Equal To 0?(x=w896) -> (x >= 0?=w895:bool)
                        n295 = Number To Decimal String(number=w917) -> (decimal integer string=w916:string)  [unwired: 1 in]
                        n296 = Not Equal?(x="0", y=w871) -> (x != y?=w887:bool)
                        n297 = Select(t="NONE" ("condition"), s=w905, f="TIMEOUT" ("condition")) -> (s? t:f=w901:string)
                        n298 = And(x=w894, y=w895) -> (x .and. y?=w893:bool)
                        n299 = case shown="True" w919 {
                          tunnel: [w942 "-1"] -> w921
                          tunnel: [w941 "NONE" ("pos_name")] -> w922
                          tunnel: w897 -> [w944 _]
                          tunnel: [w945 w967] -> w884
                          tunnel: w916 -> [w943 _]
                          tunnel: w887 -> [w940 _]
                          tunnel: w901 -> [w939 w967]
                          tunnel: [w938 w969] -> w886
                          tunnel: w899 -> [w937 w969]
                          tunnel: w870 -> [w936 w968]
                          tunnel: [w935 w968] -> w885
                          tunnel: w893 -> [w934 _]
                          frame False {
                            # "END OF MOVEMENT"
                            n300 = case shown="True" w940 {
                              tunnel: [w946 w966] -> w945
                              tunnel: w944 -> [w952 _]
                              tunnel: w943 -> [w953 _]
                              tunnel: [w953 "-1" ("t")] -> w942
                              tunnel: [w952 "NONE" ("condition")] -> w941
                              tunnel: w939 -> [_ w966]
                              tunnel: [w948 w963] -> w938
                              tunnel: w937 -> [w951 w963]
                              tunnel: w936 -> [w950 w962]
                              tunnel: [w947 w962] -> w935
                              tunnel: w934 -> [w949 _]
                              frame False {
                                # "NORMAL END"
                                n301 = case shown="True" w949 {
                                tunnel: [w956 w961] -> w948
                                tunnel: w951 -> [w956 w960]
                                tunnel: w950 -> [w955 w959]
                                tunnel: [w955 w958] -> w947
                                tunnel: ["READY" ("condition") ""] -> w946
                                frame False {
                                }
                                frame True {
                                n302 = call-dynamic "Add wprot init.vi"("error in (no error)"=w959, "ICS in"=w960) -> ("error out"=w958:errorcluster, "ICS out"=w961:refnum<class "ICS.lvclass">)  [unwired: 8 in]
                                }
                                }
                              }
                              frame True {
                                # "END WITH ERROR"
                              }
                            }
                          }
                          frame True {
                            # "FINISHED BY STOP COMMAND"
                          }
                        }
                        n303 = Equal?(x=w889, y="WPROT" ("x")) -> (x = y?=w883:bool)
                        n304 = case shown="True" w883 {
                          tunnel: [w928 w933] -> w882
                          tunnel: w886 -> [w928 w932]
                          tunnel: w885 -> [w927 w931]
                          tunnel: w884 -> [w926 w929]
                          tunnel: [w927 w930] -> w869
                          tunnel: [w926 w929] -> w880
                          frame False {
                          }
                          frame True {
                            n305 = call-dynamic "Set wpsel ready.vi"("error in (no error)"=w931, "ICS in"=w932) -> ("error out"=w930:errorcluster, "ICS out"=w933:refnum<class "ICS.lvclass">)  [unwired: 8 in]
                          }
                        }
                        n306 = call-dynamic "Write commPriority.vi"("error in (no error)"=w869, "commPriority"=FALSE ("moving"), "Motor in"=w868) -> ("error out"=w891:errorcluster, "Motor out"=w892:refnum<class "Motor.lvclass">)  [unwired: 7 in]
                        n307 = call-dynamic "Write moving flag.vi"("error in (no error)"=w891, "moving"=FALSE, "Motor in"=w892) -> ("error out"=w878:errorcluster, "Motor out"=w879:refnum<class "Motor.lvclass">)  [unwired: 7 in]
                        n308 = call-dynamic "Write command in.vi"("error in (no error)"=w878, "Motor in"=w879) -> ("error out"=w924:errorcluster, "Motor out"=w923:refnum<class "Motor.lvclass">)  [unwired: 8 in]
                        n309 = call-dynamic "Clear ack flag.vi"("error in (no error)"=w924, "Motor in"=w923) -> ("error out"=w914:errorcluster, "Motor out"=w915:refnum<class "Motor.lvclass">)  [unwired: 8 in]
                        n310 = Bundle By Name(cluster=T1 {"mode"="", "condition"="", "position"="", "pos_name"="", "pos_id"=""} ("status"), "mode"=w918, "condition"=w880, "position"=w918, "pos_name"=w922, "pos_id"=w921) -> (w913:T1)
                        n311 = call-dynamic "Write status.vi"("hold if empty"=TRUE, "error in (no error)"=w914, "status"=w913, "Motor in"=w915) -> ("error out"=w877:errorcluster, "Motor out"=w881:refnum<class "Motor.lvclass">)  [unwired: 6 in]
                      }
                      frame "SimInit" {
                        w986 = ""
                        n312 = local read "full init"() -> (w977:bool)
                        n313 = case shown="False" w977 {
                          tunnel: w978 -> [w1006 w1034]
                          tunnel: w979 -> [w1007 w1033]
                          tunnel: [w1011 w1027] -> w991
                          tunnel: [w1010 w1026] -> w990
                          tunnel: [w1009 w1024] -> w989
                          frame True {
                            w996 = 0 ("move index")
                            # "FULL INIT: SIMULATE ALL MOVEMENTS OF MECHANISM"
                            n314 = call-dynamic "Write moving flag.vi"("error in (no error)"=w1007, "moving"=TRUE, "Motor in"=w1006) -> ("error out"=w1005:errorcluster, "Motor out"=w1004:refnum<class "Motor.lvclass">)  [unwired: 7 in]
                            n315 = call <vilib>:"Space Constant.vi"() -> ("String"=w1014:string)
                            n316 = call-dynamic "Read MotorSim.vi"("error in (no error)"=w1005, "Motor in"=w1004) -> ("error out"=w999:errorcluster, "MotorSim"=w1002:refnum<class "MotorSim.lvclass">, "Motor out"=w1011:refnum<class "Motor.lvclass">)  [unwired: 7 in]
                            n317 = Concatenate Strings("INIT" ("string"), w1014, "NONE" ("string")) -> (w1003:string)
                            n318 = call-dynamic "Write move index.vi"("error in (no error)"=w999, "move index"=w996, "MotorSim in"=w1002) -> ("error out"=w998:errorcluster, "MotorSim out"=w1001:refnum<class "MotorSim.lvclass">)  [unwired: 7 in]
                            n319 = call-dynamic "Read movements.vi"("error in (no error)"=w998, "index"=w996, "MotorSim in"=w1001) -> ("error out"=w997:errorcluster, "period"=w994:u32, "initial position (0)"=w995:i32, "MotorSim out"=w1000:refnum<class "MotorSim.lvclass">, "translation (100)"=w993:i32, "forward"=w992:bool)  [unwired: 3 in]
                            n320 = call-dynamic "Start movement.vi"("motor instructions"=w1003, "translation (100)"=w993, "forward"=w992, "error in (no error)"=w997, "period"=w994, "initial position (0)"=w995, "MotorSim in"=w1000) -> ("error out"=w1009:errorcluster, "MotorSim out"=w1010:refnum<class "MotorSim.lvclass">)  [unwired: 3 in]
                          }
                          frame False {
                            # "FAST INIT: ONE DELAY ONLY IS DONE"
                            n321 = call-dynamic "Read max value.vi"("error in (no error)"=w1033, "Motor in"=w1034) -> ("error out"=w1022:errorcluster, "max value"=w1030:string, "Motor out"=w1021:refnum<class "Motor.lvclass">)  [unwired: 6 in, 1 out]
                            n322 = call <vilib>:"Space Constant.vi"() -> ("String"=w1035:string)
                            n323 = Fract/Exp String To Number(string=w1030) -> (number=w1015:dbl)  [unwired: 3 in, 1 out]
                            n324 = Random Number (0-1)() -> (number: 0 to 1=w1042:dbl)
                            n325 = Concatenate Strings("INIT" ("string"), w1035, "NONE" ("string")) -> (w1016:string)
                            n326 = call-dynamic "Write moving flag.vi"("error in (no error)"=w1022, "moving"=TRUE, "Motor in"=w1021) -> ("error out"=w1020:errorcluster, "Motor out"=w1019:refnum<class "Motor.lvclass">)  [unwired: 7 in]
                            n327 = Add(x=w1042, y=0.3) -> (x+y=w1040:dbl)
                            n328 = Divide(x=w1040, y=2.0) -> (x/y=w1036:dbl)
                            n329 = call-dynamic "Read MotorSim.vi"("error in (no error)"=w1020, "Motor in"=w1019) -> ("error out"=w1025:errorcluster, "MotorSim"=w1028:refnum<class "MotorSim.lvclass">, "Motor out"=w1027:refnum<class "Motor.lvclass">)  [unwired: 7 in]
                            n330 = Multiply(x=w1036, y=u32 12000 ("loopLimite")) -> (x*y=w1038:dbl)
                            n331 = Multiply(x=w1015, y=w1036) -> (x*y=w1043:dbl)
                            n332 = To Unsigned Long Integer(number=w1038) -> (unsigned 32bit integer=w1018:u32)
                            n333 = To Long Integer(number=w1043) -> (32bit integer=w1017:i32)
                            n334 = call-dynamic "Start movement.vi"("motor instructions"=w1016, "translation (100)"=w1017, "forward"=FALSE, "error in (no error)"=w1025, "period"=w1018, "initial position (0)"=w1017, "MotorSim in"=w1028) -> ("error out"=w1024:errorcluster, "MotorSim out"=w1026:refnum<class "MotorSim.lvclass">)  [unwired: 3 in]
                          }
                        }
                        n335 = call-dynamic "Write MotorSim.vi"("error in (no error)"=w989, "MotorSim"=w990, "Motor in"=w991) -> ("error out"=w985:errorcluster, "Motor out"=w983:refnum<class "Motor.lvclass">)  [unwired: 7 in]
                        n336 = Bundle By Name(cluster=T1 {"mode"="", "condition"="", "position"="", "pos_name"="", "pos_id"=""} ("status"), "mode"=w986, "condition"="BUSY" ("string"), "position"=w986, "pos_name"="NONE", "pos_id"="-1") -> (w981:T1)
                        n337 = call-dynamic "Write status.vi"("hold if empty"=TRUE, "error in (no error)"=w985, "status"=w981, "Motor in"=w983) -> ("error out"=w976:errorcluster, "Motor out"=w975:refnum<class "Motor.lvclass">)  [unwired: 6 in]
                      }
                      frame "SimGoto" {
                        w1065 = ""
                        n338 = call-dynamic "Read command in.vi"("error in (no error)"=w1062, "Motor in"=w1061) -> ("error out"=w1052:errorcluster, "command in"=w1084:T17, "Motor out"=w1055:refnum<class "Motor.lvclass">)  [unwired: 6 in, 1 out]
                        n339 = Unbundle By Name(w1084) -> ("action"=w1083:string, "param"=w1051:string)
                        n340 = Fract/Exp String To Number(string=w1051) -> (number=w1050:dbl)  [unwired: 3 in, 1 out]
                        n341 = call-dynamic "Unit conversion.vi"("error in (no error)"=w1052, "To(T) or From(F) Encoder"=FALSE ("hold if empty"), "value in"=w1050, "Motor in"=w1055) -> ("error out"=w1053:errorcluster, "value out"=w1049:dbl, "Motor out"=w1054:refnum<class "Motor.lvclass">)  [unwired: 5 in]
                        n342 = call-dynamic "Read max value.vi"("error in (no error)"=w1053, "Motor in"=w1054) -> ("error out"=w1069:errorcluster, "max value"=w1098:string, "position"=w1082:string, "Motor out"=w1068:refnum<class "Motor.lvclass">)  [unwired: 6 in]
                        n343 = Fract/Exp String To Number(string=w1082, default (0 dbl)=0 ("default (0 DBL)")) -> (number=w1047:i32)  [unwired: 2 in, 1 out]
                        n344 = Fract/Exp String To Number(string=w1082) -> (number=w1080:dbl)  [unwired: 3 in, 1 out]
                        n345 = Fract/Exp String To Number(string=w1098) -> (number=w1079:dbl)  [unwired: 3 in, 1 out]
                        n346 = call <vilib>:"Space Constant.vi"() -> ("String"=w1087:string)
                        n347 = Subtract(x=w1080, y=w1049) -> (x-y=w1097:dbl)
                        n348 = Concatenate Strings(w1083, w1087, w1051) -> (w1075:string)
                        n349 = Divide(x=w1097, y=w1079) -> (x/y=w1096:dbl)
                        n350 = call-dynamic "Write moving flag.vi"("error in (no error)"=w1069, "moving"=TRUE, "Motor in"=w1068) -> ("error out"=w1067:errorcluster, "Motor out"=w1066:refnum<class "Motor.lvclass">)  [unwired: 7 in]
                        n351 = Absolute Value(x=w1097) -> (abs(x)=w1090:dbl)
                        n352 = Less Than 0?(x=w1097) -> (x < 0?=w1078:bool)
                        n353 = Multiply(x=w1096, y=u32 12000 ("loopLimite")) -> (x*y=w1093:dbl)
                        n354 = Absolute Value(x=w1093) -> (abs(x)=w1091:dbl)
                        n355 = To Long Integer(number=w1090) -> (32bit integer=w1046:i32)
                        n356 = call-dynamic "Read MotorSim.vi"("error in (no error)"=w1067, "Motor in"=w1066) -> ("error out"=w1076:errorcluster, "MotorSim"=w1077:refnum<class "MotorSim.lvclass">, "Motor out"=w1074:refnum<class "Motor.lvclass">)  [unwired: 7 in]
                        n357 = To Unsigned Long Integer(number=w1091) -> (unsigned 32bit integer=w1092:u32)
                        n358 = Add(x=u32 1000 ("loopLimite"), y=w1092) -> (x+y=w1045:u32)
                        n359 = call-dynamic "Start movement.vi"("motor instructions"=w1075, "translation (100)"=w1046, "forward"=w1078, "error in (no error)"=w1076, "period"=w1045, "initial position (0)"=w1047, "MotorSim in"=w1077) -> ("error out"=w1072:errorcluster, "MotorSim out"=w1073:refnum<class "MotorSim.lvclass">)  [unwired: 3 in]
                        n360 = call-dynamic "Write MotorSim.vi"("error in (no error)"=w1072, "MotorSim"=w1073, "Motor in"=w1074) -> ("error out"=w1085:errorcluster, "Motor out"=w1086:refnum<class "Motor.lvclass">)  [unwired: 7 in]
                        n361 = Bundle By Name(cluster=T1 {"mode"="", "condition"="", "position"="", "pos_name"="", "pos_id"=""} ("status"), "mode"=w1065, "condition"="BUSY" ("string"), "position"=w1065, "pos_name"="NONE", "pos_id"="-1") -> (w1071:T1)
                        n362 = call-dynamic "Write status.vi"("hold if empty"=TRUE, "error in (no error)"=w1085, "status"=w1071, "Motor in"=w1086) -> ("error out"=w1060:errorcluster, "Motor out"=w1059:refnum<class "Motor.lvclass">)  [unwired: 6 in]
                      }
                      frame "SimUptate" {
                        w1100 = T16."SimFinish" ("stateEnum")
                        n363 = call-dynamic "Read command in.vi"("error in (no error)"=w1110, "Motor in"=w1109) -> ("error out"=w1122:errorcluster, "command in"=w1121:T17, "Motor out"=w1123:refnum<class "Motor.lvclass">)  [unwired: 6 in, 1 out]
                        n364 = Unbundle By Name(w1121) -> ("stop"=w1120:bool)
                        n365 = call-dynamic "Read MotorSim.vi"("error in (no error)"=w1122, "Motor in"=w1123) -> ("error out"=w1127:errorcluster, "MotorSim"=w1128:refnum<class "MotorSim.lvclass">, "Motor out"=w1119:refnum<class "Motor.lvclass">)  [unwired: 7 in]
                        n366 = Select(t=w1100, s=w1120, f=T16."SimUptate" ("stateEnum")) -> (s? t:f=w1112:T16)
                        n367 = local read "full init"() -> (w1101:bool)
                        n368 = call-dynamic "Get position.vi"("error in (no error)"=w1127, "MotorSim in"=w1128) -> ("error out"=w1115:errorcluster, "end"=w1118:bool, "MotorSim out"=w1117:refnum<class "MotorSim.lvclass">, "current position"=w1116:string)  [unwired: 5 in, 1 out]
                        n369 = case shown="True" w1118 {
                          tunnel: w1117 -> [w1132 w1142]
                          tunnel: w1116 -> [w1130 w1140]
                          tunnel: w1115 -> [w1131 w1141]
                          tunnel: w1100 -> [_ w1137]
                          tunnel: [w1129 w1135] -> w1106
                          tunnel: [w1130 w1139] -> w1114
                          tunnel: [w1132 w1138] -> w1113
                          tunnel: [w1131 w1134] -> w1111
                          tunnel: w1112 -> [w1129 w1136]
                          tunnel: w1101 -> [_ w1133]
                          frame False {
                          }
                          frame True {
                            n370 = case shown="True" w1133 {
                              tunnel: w1142 -> [w1144 w1163]
                              tunnel: w1141 -> [w1145 w1150]
                              tunnel: w1140 -> [w1146 w1153]
                              tunnel: [w1146 w1152] -> w1139
                              tunnel: [w1145 w1147] -> w1134
                              tunnel: [w1144 w1154] -> w1138
                              tunnel: w1137 -> [w1143 w1151]
                              tunnel: w1136 -> [_ w1155]
                              tunnel: [w1143 w1156] -> w1135
                              frame False {
                              }
                              frame True {
                                n371 = call-dynamic "Read displacements.vi"("error in (no error)"=w1150, "MotorSim in"=w1163) -> ("error out"=w1149:errorcluster, "displacements"=w1161:T11, "MotorSim out"=w1162:refnum<class "MotorSim.lvclass">)  [unwired: 7 in]
                                n372 = call-dynamic "Read move index.vi"("error in (no error)"=w1149, "MotorSim in"=w1162) -> ("error out"=w1148:errorcluster, "move index"=w1160:i32, "MotorSim out"=w1164:refnum<class "MotorSim.lvclass">)  [unwired: 7 in]
                                n373 = Increment(x=w1160) -> (x+1=w1158:i32)
                                n374 = Array Size(array=w1161) -> (size(s)=w1159:i32)
                                n375 = Equal?(x=w1158, y=w1159) -> (x = y?=w1157:bool)
                                n376 = case shown="False" w1157 {
                                tunnel: w1148 -> [w1167 w1183]
                                tunnel: w1164 -> [w1180 w1184]
                                tunnel: w1158 -> [w1177 _]
                                tunnel: [T16."SimUptate" ("stateEnum") w1181] -> w1156
                                tunnel: w1155 -> [_ _]
                                tunnel: [w1173 w1184] -> w1154
                                tunnel: [w1175 w1183] -> w1147
                                tunnel: w1153 -> [_ w1182]
                                tunnel: [w1168 w1182] -> w1152
                                tunnel: w1151 -> [_ w1181]
                                frame False {
                                n377 = call-dynamic "Write move index.vi"("error in (no error)"=w1167, "move index"=w1177, "MotorSim in"=w1180) -> ("error out"=w1178:errorcluster, "MotorSim out"=w1179:refnum<class "MotorSim.lvclass">)  [unwired: 7 in]
                                n378 = call-dynamic "Read movements.vi"("error in (no error)"=w1178, "index"=w1177, "MotorSim in"=w1179) -> ("error out"=w1176:errorcluster, "period"=w1171:u32, "initial position (0)"=w1169:i32, "MotorSim out"=w1174:refnum<class "MotorSim.lvclass">, "translation (100)"=w1170:i32, "forward"=w1172:bool)  [unwired: 3 in]
                                n379 = call-dynamic "Start movement.vi"("translation (100)"=w1170, "forward"=w1172, "error in (no error)"=w1176, "period"=w1171, "initial position (0)"=w1169, "MotorSim in"=w1174) -> ("error out"=w1175:errorcluster, "MotorSim out"=w1173:refnum<class "MotorSim.lvclass">)  [unwired: 4 in]
                                n380 = Number To Fractional String(number=w1169, precision (6)=i16 3) -> (F-format string=w1168:string)  [unwired: 2 in]
                                }
                                frame True {
                                }
                                }
                              }
                            }
                          }
                        }
                        n381 = Bundle By Name(cluster=T1 {"mode"="", "condition"="", "position"="", "pos_name"="", "pos_id"=""} ("status"), "position"=w1114) -> (w1124:T1)
                        n382 = call-dynamic "Write MotorSim.vi"("error in (no error)"=w1111, "MotorSim"=w1113, "Motor in"=w1119) -> ("error out"=w1125:errorcluster, "Motor out"=w1126:refnum<class "Motor.lvclass">)  [unwired: 7 in]
                        n383 = call-dynamic "Write status.vi"("hold if empty"=TRUE, "error in (no error)"=w1125, "status"=w1124, "Motor in"=w1126) -> ("error out"=w1108:errorcluster, "Motor out"=w1107:refnum<class "Motor.lvclass">)  [unwired: 6 in]
                      }
                      frame "SimFinish" {
                        n384 = call-dynamic "Read command in.vi"("error in (no error)"=w1215, "Motor in"=w1214) -> ("error out"=w1198:errorcluster, "command in"=w1229:T17, "Motor out"=w1200:refnum<class "Motor.lvclass">)  [unwired: 6 in, 1 out]
                        n385 = Unbundle By Name(w1229) -> ("param"=w1202:string, "pos_name"=w1191:string, "pos_idx"=w1209:i32, "stop"=w1216:bool)  [unwired: 2 out]
                        n386 = call-dynamic "Read name.vi"("error in (no error)"=w1198, "Motor in"=w1200) -> ("error out"=w1189:errorcluster, "name"=w1197:string, "Motor out"=w1199:refnum<class "Motor.lvclass">)  [unwired: 7 in]
                        n387 = Equal?(x=w1197, y="WPSEL") -> (x = y?=w1195:bool)
                        n388 = call-dynamic "Encoder to mechanism position.vi"("error in (no error)"=w1189, "motor position"=w1202, "Motor in"=w1199) -> ("error out"=w1204:errorcluster, "mechanism position"=w1201:string, "Motor out"=w1203:refnum<class "Motor.lvclass">)  [unwired: 6 in]
                        n389 = Search and Replace String(input string=w1191, search string="L/" ("replace string (\"\")")) -> (offset past replacement=w1190:i32)  [unwired: 6 in, 3 out]
                        n390 = case shown="False" w1216 {
                          tunnel: [w1248 "-1"] -> w1221
                          tunnel: [w1242 "NONE" ("pos_name")] -> w1207
                          tunnel: w1209 -> [w1247 _]
                          tunnel: w1191 -> [w1242 _]
                          tunnel: [w1244 ""] -> w1206
                          tunnel: ["READY" ("condition") "TIMEOUT" ("pos_name")] -> w1205
                          tunnel: w1201 -> [w1245 _]
                          tunnel: w1195 -> [w1241 _]
                          tunnel: w1194 -> [w1237 w1256]
                          tunnel: [w1236 w1256] -> w1193
                          tunnel: w1190 -> [w1239 _]
                          tunnel: [w1235 w1255] -> w1188
                          tunnel: w1189 -> [w1234 w1255]
                          frame False {
                            # "END OF MOVEMENT"
                            n391 = Greater Or Equal To 0?(x=w1239) -> (x >= 0?=w1240:bool)
                            n392 = Search and Replace String(input string=w1245, search string="-") -> (result string=w1244:string)  [unwired: 6 in, 3 out]
                            n393 = Number To Decimal String(number=w1247) -> (decimal integer string=w1248:string)  [unwired: 1 in]
                            n394 = And(x=w1241, y=w1240) -> (x .and. y?=w1238:bool)
                            n395 = case shown="True" w1238 {
                              tunnel: w1237 -> [w1250 w1254]
                              tunnel: [w1250 w1253] -> w1236
                              tunnel: w1234 -> [w1249 w1252]
                              tunnel: [w1249 w1251] -> w1235
                              frame False {
                              }
                              frame True {
                                n396 = call-dynamic "Add wprot init.vi"("error in (no error)"=w1252, "ICS in"=w1254) -> ("error out"=w1251:errorcluster, "ICS out"=w1253:refnum<class "ICS.lvclass">)  [unwired: 8 in]
                              }
                            }
                          }
                          frame True {
                            # "FINISHED BY STOP COMMAND"
                          }
                        }
                        n397 = call-dynamic "Write moving flag.vi"("error in (no error)"=w1204, "moving"=FALSE, "Motor in"=w1203) -> ("error out"=w1223:errorcluster, "Motor out"=w1226:refnum<class "Motor.lvclass">)  [unwired: 7 in]
                        n398 = call-dynamic "Write command in.vi"("error in (no error)"=w1223, "Motor in"=w1226) -> ("error out"=w1224:errorcluster, "Motor out"=w1225:refnum<class "Motor.lvclass">)  [unwired: 8 in]
                        n399 = call-dynamic "Read MotorSim.vi"("error in (no error)"=w1224, "Motor in"=w1225) -> ("error out"=w1187:errorcluster, "MotorSim"=w1233:refnum<class "MotorSim.lvclass">, "Motor out"=w1232:refnum<class "Motor.lvclass">)  [unwired: 7 in]
                        n400 = Merge Errors(w1187, w1188) -> (w1186:errorcluster)
                        n401 = call-dynamic "Get position.vi"("error in (no error)"=w1186, "MotorSim in"=w1233) -> ("error out"=w1230:errorcluster, "MotorSim out"=w1231:refnum<class "MotorSim.lvclass">)  [unwired: 5 in, 3 out]
                        n402 = Bundle By Name(cluster=T1 {"mode"="", "condition"="", "position"="", "pos_name"="", "pos_id"=""} ("status"), "mode"="", "condition"=w1205, "position"=w1206, "pos_name"=w1207, "pos_id"=w1221) -> (w1228:T1)
                        n403 = call-dynamic "Write MotorSim.vi"("error in (no error)"=w1230, "MotorSim"=w1231, "Motor in"=w1232) -> ("error out"=w1220:errorcluster, "Motor out"=w1217:refnum<class "Motor.lvclass">)  [unwired: 7 in]
                        n404 = call-dynamic "Clear ack flag.vi"("error in (no error)"=w1220, "Motor in"=w1217) -> ("error out"=w1219:errorcluster, "Motor out"=w1218:refnum<class "Motor.lvclass">)  [unwired: 8 in]
                        n405 = call-dynamic "Write status.vi"("hold if empty"=TRUE, "error in (no error)"=w1219, "status"=w1228, "Motor in"=w1218) -> ("error out"=w1213:errorcluster, "Motor out"=w1212:refnum<class "Motor.lvclass">)  [unwired: 6 in]
                      }
                      frame "CyclicStart" {
                        w1277 = ""
                        n406 = call-dynamic "Read action-param.vi"("error in (no error)"=w1286, "Motor in"=w1287) -> ("error out"=w1285:errorcluster, "param"=w1283:string, "Motor out"=w1284:refnum<class "Motor.lvclass">)  [unwired: 6 in, 1 out]
                        n407 = local read "enabled log"() -> (w1263:string)
                        n408 = call-dynamic "Get cyclic instructions.vi"("error in (no error)"=w1285, "cyclic parameter"=w1283, "Motor in"=w1284) -> ("error out"=w1291:errorcluster, "start"=w1279:bool, "cyclic instructions"=w1265:string[], "Motor out"=w1292:refnum<class "Motor.lvclass">)  [unwired: 5 in]
                        n409 = Select(t=T16."CyclicUpdate" ("stateEnum"), s=w1279, f=T16."CyclicFinish" ("stateEnum")) -> (s? t:f=w1282:T16)
                        n410 = call-dynamic "Send instructions.vi"("error in (no error)"=w1291, "instructions"=w1265, "Motor in"=w1292) -> ("error out"=w1268:errorcluster, "replies"=w1266:string[], "Motor out"=w1293:refnum<class "Motor.lvclass">, "ok"=w1294:bool)  [unwired: 4 in, 1 out]
                        n411 = call "Write log to file.vi"("current priority"="1", "enabled priority"=w1263, "error in"=w1268, "resp array"=w1266, "send array"=w1265, "prefix"="<Cyclic Start> ") -> ("error out"=w1267:errorcluster)  [unwired: 3 in, 2 out]
                        n412 = case shown="True" w1294 {
                          tunnel: w1267 -> [w1301 w1310]
                          tunnel: w1293 -> [w1302 w1311]
                          tunnel: [w1298 w1314] -> w1273
                          tunnel: [w1297 w1313] -> w1272
                          tunnel: [T16."Wait" ("stateEnum") w1307] -> w1290
                          tunnel: w1282 -> [_ w1307]
                          tunnel: w1279 -> [_ w1306]
                          tunnel: [w1295 w1305] -> w1276
                          tunnel: [w1295 w1304] -> w1275
                          tunnel: ["TIMEOUT" ("string") "BUSY"] -> w1274
                          frame False {
                            w1295 = ""
                            # "ERROR: CLEAR COMMAND INPUT"
                            n413 = call-dynamic "Write command in.vi"("error in (no error)"=w1301, "command in"=T17 {"action"="", "param"="", "pos_name"="", "pos_idx"=0, "ack"=FALSE, "stop"=FALSE, "offset"=FALSE, "immediate"=FALSE, "instructions"=[]}, "Motor in"=w1302) -> ("error out"=w1297:errorcluster, "Motor out"=w1298:refnum<class "Motor.lvclass">)  [unwired: 7 in]
                          }
                          frame True {
                            # "MOTOR RECEIVED INSTRUCTIONS: SET BUSY CONDITION"
                            n414 = case shown="False" w1306 {
                              tunnel: [w1315 "NONE"] -> w1305
                              tunnel: [w1315 "-1"] -> w1304
                              frame False {
                                w1315 = ""
                              }
                              frame True {
                              }
                            }
                            n415 = call-dynamic "Write cyclic flag.vi"("error in (no error)"=w1310, "cyclic"=w1306, "Motor in"=w1311) -> ("error out"=w1308:errorcluster, "Motor out"=w1309:refnum<class "Motor.lvclass">)  [unwired: 7 in]
                            n416 = call-dynamic "Write moving flag.vi"("error in (no error)"=w1308, "moving"=TRUE ("hold if empty"), "Motor in"=w1309) -> ("error out"=w1313:errorcluster, "Motor out"=w1314:refnum<class "Motor.lvclass">)  [unwired: 7 in]
                          }
                        }
                        n417 = Bundle By Name(cluster=T1 {"mode"="", "condition"="", "position"="", "pos_name"="", "pos_id"=""} ("status"), "mode"=w1277, "condition"=w1274, "position"=w1277, "pos_name"=w1276, "pos_id"=w1275) -> (w1269:T1)
                        n418 = call-dynamic "Write status.vi"("hold if empty"=TRUE, "error in (no error)"=w1272, "status"=w1269, "Motor in"=w1273) -> ("error out"=w1270:errorcluster, "Motor out"=w1271:refnum<class "Motor.lvclass">)  [unwired: 6 in]
                      }
                      frame "CyclicUpdate" {
                        # "TO STOP PRG1 WITHOUT ANY WP MOVEMENT, ICS MUST WRITE V42=0 AND THEN INVERT AND RESTORE THE POLARITY OF DI2 INPUT (POL=2064 / POL=16)."
                        n419 = call-dynamic "Read stop flag.vi"("error in (no error)"=w1336, "Motor in"=w1337) -> ("error out"=w1326:errorcluster, "stop"=w1324:bool, "Motor out"=w1327:refnum<class "Motor.lvclass">)  [unwired: 7 in]
                        n420 = call-dynamic "Clear stop flag.vi"("error in (no error)"=w1326, "Motor in"=w1327) -> ("error out"=w1325:errorcluster, "Motor out"=w1328:refnum<class "Motor.lvclass">)  [unwired: 8 in]
                        n421 = disable-structure shown="Enabled" {
                          disable-tunnel: ["LTEX" "V31"] -> w1338
                          frame Disabled {
                          }
                          frame Enabled {
                          }
                        }
                        n422 = Build Array("V42=0", "POL=2064", "POL=16") -> (w1331:string[])
                        n423 = Build Array(w1338) -> (w1335:string[])
                        n424 = Select(t=w1331, s=w1324, f=w1335) -> (s? t:f=w1320:string[])
                        n425 = Select(t=T16."CyclicFinish" ("stateEnum"), s=w1324, f=T16."CyclicUpdate" ("stateEnum")) -> (s? t:f=w1319:T16)
                        n426 = call-dynamic "Send instructions.vi"("error in (no error)"=w1325, "instructions"=w1320, "Motor in"=w1328) -> ("error out"=w1341:errorcluster, "replies"=w1343:string[], "Motor out"=w1342:refnum<class "Motor.lvclass">, "ok"=w1321:bool)  [unwired: 4 in, 1 out]
                        n427 = case shown="True" w1321 {
                          tunnel: w1343 -> [w1348 _]
                          tunnel: w1342 -> [w1354 w1367]
                          tunnel: w1341 -> [w1352 w1366]
                          tunnel: [w1353 w1357] -> w1329
                          tunnel: [w1354 w1356] -> w1330
                          tunnel: w1320 -> [w1349 w1369]
                          tunnel: w1319 -> [_ w1355]
                          tunnel: [T16."CyclicUpdate" ("stateEnum") w1355] -> w1318
                          frame False {
                            # "COMMUNICATION ERROR"
                            n428 = local read "enabled log"() -> (w1351:string)
                            n429 = call "Write log to file.vi"("current priority"="1", "enabled priority"=w1351, "error in"=w1352, "resp array"=w1348, "send array"=w1349, "prefix"="<Cyclic Update> ") -> ("error out"=w1353:errorcluster)  [unwired: 3 in, 2 out]
                          }
                          frame True {
                            w1362 = ""
                            # "CORRECTION HAS NOT YET BEEN IMPLEMENTED."
                            # "CHECK AND CORRECT CYCLIC POSITION"
                            n430 = Index Array(array=w1369, index=0) -> (element=w1365:string)
                            n431 = call-dynamic "Read predef by index.vi"("error in (no error)"=w1366, "index"=w1365, "Motor in"=w1367) -> ("error out"=w1359:errorcluster, "pos_name"=w1364:string, "pos_value"=w1363:string, "Motor out"=w1360:refnum<class "Motor.lvclass">)  [unwired: 5 in]
                            n432 = Bundle By Name(cluster=T1 {"mode"="", "condition"="", "position"="", "pos_name"="", "pos_id"=""} ("status"), "mode"=w1362, "condition"=w1362, "position"=w1363, "pos_name"=w1364, "pos_id"=w1365) -> (w1358:T1)
                            n433 = call-dynamic "Write status.vi"("hold if empty"=TRUE, "error in (no error)"=w1359, "status"=w1358, "Motor in"=w1360) -> ("error out"=w1357:errorcluster, "Motor out"=w1356:refnum<class "Motor.lvclass">)  [unwired: 6 in]
                          }
                        }
                      }
                      frame "CyclicFinish" {
                        n434 = call-dynamic "Read cyclic flag.vi"("error in (no error)"=w1389, "Motor in"=w1390) -> ("error out"=w1387:errorcluster, "cyclic"=w1386:bool, "Motor out"=w1388:refnum<class "Motor.lvclass">)  [unwired: 7 in]
                        n435 = Build Array("V31", "SR1=0") -> (w1392:string[])
                        n436 = case shown="True" w1386 {
                          tunnel: w1392 -> [_ w1409]
                          tunnel: w1388 -> [w1399 w1414]
                          tunnel: w1387 -> [w1398 w1413]
                          tunnel: [w1399 w1412] -> w1378
                          tunnel: [w1398 w1407] -> w1377
                          tunnel: [w1397 w1411] -> w1376
                          tunnel: [T16."Wait" ("stateEnum") w1401] -> w1371
                          frame False {
                            w1396 = ""
                            # "SINGLE OR SEVERAL OR U16 CYCLIC COMMAND WAS EXECUTED"
                            n437 = Bundle By Name(cluster=T1 {"mode"="", "condition"="", "position"="", "pos_name"="", "pos_id"=""} ("status"), "mode"=w1396, "condition"="READY", "position"=w1396, "pos_name"=w1396, "pos_id"=w1396) -> (w1397:T1)
                          }
                          frame True {
                            # "CYCLE ENABLED"
                            n438 = local read "enabled log"() -> (w1406:string)
                            n439 = call-dynamic "Send instructions.vi"("error in (no error)"=w1413, "instructions"=w1409, "Motor in"=w1414) -> ("error out"=w1404:errorcluster, "error"=w1410:bool, "replies"=w1408:string[], "Motor out"=w1415:refnum<class "Motor.lvclass">)  [unwired: 4 in, 1 out]
                            n440 = call "Write log to file.vi"("current priority"="1", "enabled priority"=w1406, "error in"=w1404, "resp array"=w1408, "send array"=w1409, "prefix"="<Cyclic Finish> ") -> ("error out"=w1403:errorcluster)  [unwired: 3 in, 2 out]
                            n441 = case shown="False" w1410 {
                              tunnel: w1415 -> [w1432 w1457]
                              tunnel: w1403 -> [w1431 w1458]
                              tunnel: [w1418 w1458] -> w1407
                              tunnel: [w1417 w1457] -> w1412
                              tunnel: w1408 -> [w1429 _]
                              tunnel: [w1430 w1456] -> w1411
                              tunnel: [T16."Wait" ("stateEnum") T16."CyclicFinish" ("stateEnum")] -> w1401
                              frame False {
                                # "UPDATE WPROT STATUS"
                                n442 = Index Array(array=w1429, index=0) -> (element=w1423:string)
                                n443 = call-dynamic "Read predef by index.vi"("error in (no error)"=w1431, "index"=w1423, "Motor in"=w1432) -> ("error out"=w1419:errorcluster, "pos_name"=w1422:string, "pos_value"=w1427:string, "Motor out"=w1420:refnum<class "Motor.lvclass">)  [unwired: 5 in]
                                n444 = disable-structure shown="Enabled" {
                                disable-tunnel: [w1441 "READY" ("condition")] -> w1428
                                disable-tunnel: w1427 -> [w1436 w1452]
                                disable-tunnel: [_ w1452] -> w1426
                                disable-tunnel: [w1440 w1451] -> w1425
                                disable-tunnel: [w1439 w1450] -> w1424
                                disable-tunnel: w1423 -> [w1438 w1450]
                                disable-tunnel: w1422 -> [w1437 w1451]
                                frame Disabled {
                                n445 = case shown="False" {
                                selector: _ -> [_ _]
                                tunnel: w1436 -> [_ w1448]
                                tunnel: w1437 -> [_ w1449]
                                tunnel: ["NONE" ("x") w1449] -> w1440
                                tunnel: ["" w1448] -> _
                                tunnel: ["-1" ("x") w1447] -> w1439
                                tunnel: w1438 -> [_ w1447]
                                tunnel: ["TIMEOUT" ("x") "READY" ("condition")] -> w1441
                                frame False {
                                # "FAIL"
                                }
                                frame True {
                                # "OK"
                                }
                                }
                                }
                                frame Enabled {
                                }
                                }
                                n446 = Bundle By Name(cluster=T1 {"mode"="", "condition"="", "position"="", "pos_name"="", "pos_id"=""} ("status"), "mode"="", "condition"=w1428, "position"=w1426, "pos_name"=w1425, "pos_id"=w1424) -> (w1430:T1)
                                n447 = call-dynamic "Write cyclic flag.vi"("error in (no error)"=w1419, "cyclic"=FALSE, "Motor in"=w1420) -> ("error out"=w1418:errorcluster, "Motor out"=w1417:refnum<class "Motor.lvclass">)  [unwired: 7 in]
                              }
                              frame True {
                                w1454 = ""
                                # "RETRY"
                                n448 = Bundle By Name(cluster=T1 {"mode"="", "condition"="", "position"="", "pos_name"="", "pos_id"=""} ("status"), "mode"=w1454, "condition"=w1454, "position"=w1454, "pos_name"=w1454, "pos_id"=w1454) -> (w1456:T1)
                              }
                            }
                          }
                        }
                        n449 = call-dynamic "Write status.vi"("hold if empty"=TRUE, "error in (no error)"=w1377, "status"=w1376, "Motor in"=w1378) -> ("error out"=w1385:errorcluster, "Motor out"=w1384:refnum<class "Motor.lvclass">)  [unwired: 6 in]
                        n450 = call-dynamic "Write moving flag.vi"("error in (no error)"=w1385, "moving"=FALSE, "Motor in"=w1384) -> ("error out"=w1380:errorcluster, "Motor out"=w1381:refnum<class "Motor.lvclass">)  [unwired: 7 in]
                        n451 = call-dynamic "Write command in.vi"("error in (no error)"=w1380, "command in"=T17 {"action"="", "param"="", "pos_name"="", "pos_idx"=0, "ack"=FALSE, "stop"=FALSE, "offset"=FALSE, "immediate"=FALSE, "instructions"=[]}, "Motor in"=w1381) -> ("error out"=w1373:errorcluster, "Motor out"=w1391:refnum<class "Motor.lvclass">)  [unwired: 7 in]
                      }
                    }
                    n452 = call-dynamic "Write current state.vi"("error in (no error)"=w594, "currentState"=w591, "StateManager in"=w595) -> ("error out"=w605:errorcluster, "StateManager out"=w606:refnum<class "StateManager.lvclass">)  [unwired: 7 in]
                    n453 = call-dynamic "Write StateManager.vi"("error in (no error)"=w605, "StateManager"=w606, "Motor in"=w596) -> ("error out"=w603:errorcluster, "Motor out"=w602:refnum<class "Motor.lvclass">)  [unwired: 7 in]
                    n454 = call-dynamic "Write selected motor.vi"("error in (no error)"=w603, "Motor.lvclass"=w602, "ICS in"=w597) -> ("error out"=w601:errorcluster, "ICS out"=w604:refnum<class "ICS.lvclass">)  [unwired: 7 in]
                  }
                }
              }
              frame True {
                w1479 = "WPROT"
                # "VALID MESSAGE RECEIVED FROM CLIENT: VALIDATE & REPLY COMMAND"
                n455 = call-dynamic "Read motors.vi"("error in (no error)"=w1500, "ICS in"=w1499) -> ("error out"=w1497:errorcluster, "motors"=w1496:refnum<class "Motor.lvclass">[], "ICS out"=w1498:refnum<class "ICS.lvclass">)  [unwired: 7 in]
                n456 = case shown="True" w1495 {
                  tunnel: [w1598 w1607] -> w1501
                  tunnel: [w1599 w1606] -> w1490
                  tunnel: w1498 -> [w1599 w1606]
                  tunnel: w1497 -> [w1598 w1603]
                  tunnel: w1496 -> [w1600 w1604]
                  tunnel: [w1600 w1605] -> w1494
                  tunnel: [bool[] [] w1602] -> w1475
                  tunnel: w1473 -> [_ w1601]
                  frame False {
                  }
                  frame True {
                    n457 = for {
                      tunnel: w1604 -> [w1612] mode=indexing
                      tunnel: w1601 -> [w1611]
                      tunnel: w1603 -> [w1613]
                      tunnel: [w1610] -> w1607
                      tunnel: [w1609] -> w1605 mode=indexing
                      tunnel: [w1608] -> w1602 mode=indexing
                      n458 = call-dynamic "Validate command.vi"("error in (no error)"=w1613, "message"=w1611, "Motor in"=w1612) -> ("error out"=w1610:errorcluster, "ack"=w1608:bool, "Motor out"=w1609:refnum<class "Motor.lvclass">)  [unwired: 6 in]
                    }
                  }
                }
                n459 = for {
                  tunnel: w1494 -> [w1625] mode=indexing
                  shift-right: [w1617] -> w1469
                  shift-left: "" -> [w1616]
                  shift-right: [w1615] -> w1491
                  shift-left: w1501 -> [w1626]
                  tunnel: [w1614] -> w1489 mode=indexing
                  i -> [w1624]
                  # "CREATE STATUS MESSAGE"
                  n460 = Equal?(x=5, y=w1624) -> (x = y?=w1622:bool)
                  n461 = call-dynamic "Get status.vi"("error in (no error)"=w1626, "Motor in"=w1625) -> ("error out"=w1615:errorcluster, "status string"=w1618:string, "Motor out"=w1614:refnum<class "Motor.lvclass">)  [unwired: 7 in]
                  n462 = Select(t="\r\n", s=w1622, f=", ") -> (s? t:f=w1619:string)
                  n463 = Concatenate Strings(w1616, w1618, w1619) -> (w1617:string)
                }
                n464 = Boolean Array To Number(Boolean array=w1475) -> (number=w1474:u32)
                n465 = Not Equal To 0?(x=w1474) -> (x != 0?=w1468:bool)
                n466 = call-dynamic "Write motors.vi"("error in (no error)"=w1491, "motors"=w1489, "ICS in"=w1490) -> ("error out"=w1464:errorcluster, "ICS out"=w1462:refnum<class "ICS.lvclass">)  [unwired: 7 in]
                n467 = case shown="False" w1460 {
                  tunnel: [w1508 w1539] -> w1488
                  tunnel: [w1507 w1538] -> w1471
                  tunnel: w1469 -> [w1506 _]
                  tunnel: w1464 -> [w1505 w1538]
                  tunnel: w1462 -> [w1504 w1539]
                  tunnel: w1461 -> [w1503 _]
                  frame False {
                    # "NO COMMAND AT 0MQ PULL"
                    n468 = case shown="False" w1503 {
                      tunnel: [w1513 w1533] -> w1507
                      tunnel: w1505 -> [w1512 w1529]
                      tunnel: w1506 -> [w1511 w1537]
                      tunnel: [w1510 w1531] -> w1508
                      tunnel: w1504 -> [w1509 w1527]
                      frame False {
                        # "SEND STATUS TO CLIENT\nUSING INTERCOMM VI"
                        n469 = disable-structure shown="Enabled" {
                          disable-tunnel: [w1523 w1524] -> w1513
                          disable-tunnel: w1512 -> [w1518 w1524]
                          disable-tunnel: w1511 -> [w1522 _]
                          disable-tunnel: [w1521 w1525] -> w1510
                          disable-tunnel: w1509 -> [w1516 w1525]
                          frame Enabled {
                            n470 = call-dynamic "Read Messenger.vi"("error in (no error)"=w1518, "ICS in"=w1516) -> ("error out"=w1517:errorcluster, "Messenger.lvclass"=w1515:refnum<class "Messenger.lvclass">, "ICS out"=w1514:refnum<class "ICS.lvclass">)  [unwired: 7 in]
                            n471 = call-dynamic "Send status.vi"("error in (no error)"=w1517, "status"=w1522, "Messenger in"=w1515) -> ("error out"=w1520:errorcluster, "Messenger out"=w1519:refnum<class "Messenger.lvclass">)  [unwired: 7 in]
                            n472 = call-dynamic "Write Messenger.vi"("error in (no error)"=w1520, "Messenger.lvclass"=w1519, "ICS in"=w1514) -> ("error out"=w1523:errorcluster, "ICS out"=w1521:refnum<class "ICS.lvclass">)  [unwired: 7 in]
                          }
                          frame Disabled {
                          }
                        }
                      }
                      frame True {
                        # "SEND STATUS TO CLIENT\nUSING INNER TCP/IP CONNECTION"
                        n473 = call "Read Server.vi"("error in (no error)"=w1529, "ICS in"=w1527) -> ("error out"=w1528:errorcluster, "Server"=w1530:refnum<class "TCP-Server.lvclass">, "ICS out"=w1526:refnum<class "ICS.lvclass">)  [unwired: 7 in]
                        n474 = call-dynamic "Send message.vi"("error in (no error)"=w1528, "message"=w1537, "Server in"=w1530) -> ("error out"=w1536:errorcluster, "Server out"=w1535:refnum<class "TCP-Server.lvclass">)  [unwired: 7 in]
                        n475 = call-dynamic "Close connection.vi"("error in (no error)"=w1536, "Server in"=w1535) -> ("error out"=w1534:errorcluster, "Server out"=w1532:refnum<class "TCP-Server.lvclass">)  [unwired: 8 in]
                        n476 = call "Write Server.vi"("error in (no error)"=w1534, "Server"=w1532, "ICS in"=w1526) -> ("error out"=w1533:errorcluster, "ICS out"=w1531:refnum<class "ICS.lvclass">)  [unwired: 7 in]
                      }
                    }
                  }
                  frame True {
                    # "DO NOT SEND STATUS TO\nCLIENTS CONNECTED USING\nTCP/IP OR INTERCOMM.VI\n(NO CONNECTION TO THEM)"
                    # "THE COMMAND COMES FROM 0MQ PULL"
                  }
                }
                n477 = case shown="True" w1468 {
                  tunnel: w1469 -> [_ w1547]
                  tunnel: w1473 -> [_ w1548]
                  tunnel: w1464 -> [w1540 w1543]
                  tunnel: [w1540 w1541] -> w1463
                  frame False {
                  }
                  frame True {
                    # "WRITE STATUS  & LOG CMD"
                    n478 = call "Write log to file.vi"("current priority"="3", "enabled priority"="enabled log", "error in"=w1543, "prefix"=w1548) -> ("error out"=w1542:errorcluster)  [unwired: 5 in, 2 out]
                    n479 = call "Write log to file.vi"("current priority"="4", "enabled priority"="enabled log", "error in"=w1542, "prefix"=w1547) -> ("error out"=w1541:errorcluster)  [unwired: 5 in, 2 out]
                  }
                }
                n480 = call-dynamic "Read motor by name.vi"("error in (no error)"=w1471, "motor name"=w1479, "ICS in"=w1488) -> ("error out"=w1487:errorcluster, "Motor.lvclass"=w1486:refnum<class "Motor.lvclass">, "ICS out"=w1470:refnum<class "ICS.lvclass">)  [unwired: 5 in, 1 out]
                n481 = local read "enabled log"() -> (w1466:string)
                n482 = call-dynamic "Read command in.vi"("error in (no error)"=w1487, "Motor in"=w1486) -> ("error out"=w1482:errorcluster, "command in"=w1485:T17, "Motor out"=w1481:refnum<class "Motor.lvclass">)  [unwired: 6 in, 1 out]
                n483 = Unbundle By Name(w1485) -> ("immediate"=w1484:bool, "instructions"=w1483:string[], "action"=w1478:string)
                n484 = Equal?(x=w1478, y="CYCLIC") -> (x = y?=w1476:bool)
                n485 = case shown="True" w1484 {
                  tunnel: w1483 -> [_ w1558]
                  tunnel: w1482 -> [w1549 w1568]
                  tunnel: w1481 -> [w1551 w1569]
                  tunnel: [w1549 w1557] -> w1465
                  tunnel: [w1551 w1564] -> w1480
                  tunnel: w1476 -> [_ w1559]
                  tunnel: [w1550 w1556] -> w1472
                  tunnel: w1470 -> [w1550 w1556]
                  tunnel: "<Immediate> " ("current priority") -> [_ w1553]
                  tunnel: w1466 -> [_ w1552]
                  tunnel: w1463 -> [_ _]
                  frame False {
                  }
                  frame True {
                    n486 = call-dynamic "Send and log instructions.vi"("prefix"=w1553, "current code"="2" ("current priority"), "enabled codes"=w1552, "error in (no error)"=w1568, "instructions"=w1558, "Motor in"=w1569) -> ("error out"=w1555:errorcluster, "error"=w1567:bool, "Motor out"=w1566:refnum<class "Motor.lvclass">)  [unwired: 1 in, 2 out]
                    n487 = Select(t=T16."CyclicUpdate" ("stateEnum"), s=w1559, f=T16."ActiveUpdate" ("stateEnum")) -> (s? t:f=w1560:T16)
                    n488 = case shown="False" w1567 {
                      tunnel: w1555 -> [w1590 w1596]
                      tunnel: w1566 -> [w1589 w1595]
                      tunnel: [w1572 w1596] -> w1565
                      tunnel: [w1574 w1595] -> w1563
                      tunnel: w1560 -> [w1576 _]
                      tunnel: w1559 -> [w1571 _]
                      frame False {
                        w1586 = ""
                        # "MANTER POS_NAME\nE POS_ID EM CYCLIC?"
                        n489 = call-dynamic "Read StateManager.vi"("error in (no error)"=w1590, "Motor in"=w1589) -> ("error out"=w1592:errorcluster, "StateManager"=w1591:refnum<class "StateManager.lvclass">, "Motor out"=w1588:refnum<class "Motor.lvclass">)  [unwired: 5 in, 2 out]
                        n490 = Bundle By Name(cluster=T1 {"mode"="", "condition"="", "position"="", "pos_name"="", "pos_id"=""} ("status"), "mode"=w1586, "condition"="BUSY" ("string"), "position"=w1586, "pos_name"="NONE", "pos_id"="-1") -> (w1579:T1)
                        n491 = call-dynamic "Write current state.vi"("error in (no error)"=w1592, "currentState"=w1576, "StateManager in"=w1591) -> ("error out"=w1593:errorcluster, "StateManager out"=w1594:refnum<class "StateManager.lvclass">)  [unwired: 7 in]
                        n492 = call-dynamic "Write StateManager.vi"("error in (no error)"=w1593, "StateManager"=w1594, "Motor in"=w1588) -> ("error out"=w1577:errorcluster, "Motor out"=w1578:refnum<class "Motor.lvclass">)  [unwired: 7 in]
                        n493 = call-dynamic "Write status.vi"("hold if empty"=TRUE, "error in (no error)"=w1577, "status"=w1579, "Motor in"=w1578) -> ("error out"=w1583:errorcluster, "Motor out"=w1582:refnum<class "Motor.lvclass">)  [unwired: 6 in]
                        n494 = call-dynamic "Write moving flag.vi"("error in (no error)"=w1583, "moving"=TRUE, "Motor in"=w1582) -> ("error out"=w1573:errorcluster, "Motor out"=w1575:refnum<class "Motor.lvclass">)  [unwired: 7 in]
                        n495 = call-dynamic "Write cyclic flag.vi"("error in (no error)"=w1573, "cyclic"=w1571, "Motor in"=w1575) -> ("error out"=w1572:errorcluster, "Motor out"=w1574:refnum<class "Motor.lvclass">)  [unwired: 7 in]
                      }
                      frame True {
                      }
                    }
                    n496 = call-dynamic "Clear immediate flag.vi"("error in (no error)"=w1565, "Motor in"=w1563) -> ("error out"=w1557:errorcluster, "Motor out"=w1564:refnum<class "Motor.lvclass">)  [unwired: 8 in]
                  }
                }
                n497 = call-dynamic "Write motor by name.vi"("error in (no error)"=w1465, "name"=w1479, "motor"=w1480, "ICS in"=w1472) -> ("error out"=w1492:errorcluster, "ICS out"=w1493:refnum<class "ICS.lvclass">)  [unwired: 6 in]
              }
            }
          }
        }
      }
      event "login help": Value Change {
        n498 = event-data() -> ()  [unwired: 1 in, 6 out]
        n499 = call "Help login.vi"() -> ()  [unwired: 12 in]
      }
      event "language": Value Change {
        n500 = event-data() -> ()  [unwired: 1 in, 6 out]
        n501 = control-ref of="check email"() -> (w1639:refnum<vi>)
        n502 = control-ref of="email ok"() -> (w1638:refnum<vi>)
        n503 = control-ref of="port"() -> (w1642:refnum<vi>)
        n504 = control-ref of="timeout"() -> (w1629:refnum<vi>)
        n505 = control-ref of="address"() -> (w1637:refnum<vi>)
        n506 = control-ref of="local IP 1"() -> (w1636:refnum<vi>)
        n507 = control-ref of="local IP 2"() -> (w1635:refnum<vi>)
        n508 = control-ref of="language"() -> (w1682:refnum<vi>)
        n509 = Build Array(w1639, w1638, w1637, w1642, w1629, w1636, w1635) -> (w1643:refnum<vi>[])
        n510 = control-ref of="server"() -> (w1684:refnum<vi>)
        n511 = control-ref of="exitLogin"() -> (w1683:refnum<vi>)
        n512 = control-ref of="login help"() -> (w1679:refnum<vi>)
        n513 = control-ref of="login"() -> (w1678:refnum<vi>)
        n514 = control-ref of="start server"() -> (w1675:refnum<vi>)
        n515 = control-ref of="exitStopped"() -> (w1674:refnum<vi>)
        n516 = control-ref of="assist"() -> (w1673:refnum<vi>)
        n517 = control-ref of="setup"() -> (w1672:refnum<vi>)
        n518 = control-ref of="control"() -> (w1671:refnum<vi>)
        n519 = control-ref of="loginUser"() -> (w1681:refnum<vi>)
        n520 = control-ref of="loginPW"() -> (w1680:refnum<vi>)
        n521 = Build Array(w1684, w1683, w1682, w1681, w1680, w1679, w1678, w1675, w1674, w1673, w1672, w1671) -> (w1677:refnum<vi>[])
        n522 = control-ref of="return assist"() -> (w1659:refnum<vi>)
        n523 = control-ref of="return control"() -> (w1658:refnum<vi>)
        n524 = control-ref of="logout stopped"() -> (w1670:refnum<vi>)
        n525 = control-ref of="stop server"() -> (w1669:refnum<vi>)
        n526 = control-ref of="logout running"() -> (w1668:refnum<vi>)
        n527 = control-ref of="save config"() -> (w1667:refnum<vi>)
        n528 = control-ref of="save as"() -> (w1666:refnum<vi>)
        n529 = control-ref of="config help"() -> (w1665:refnum<vi>)
        n530 = control-ref of="return setup"() -> (w1661:refnum<vi>)
        n531 = control-ref of="cfgFile"() -> (w1664:refnum<vi>)
        n532 = control-ref of="last cfg user"() -> (w1663:refnum<vi>)
        n533 = control-ref of="last cfg date"() -> (w1662:refnum<vi>)
        n534 = Build Array(w1670, w1669, w1668, w1667, w1666, w1665, w1664, w1663, w1662, w1661, w1659, w1658) -> (w1660:refnum<vi>[])
        n535 = Insert Into Array(array=w1677, new element=w1660) -> (w1644:refnum<vi>[])  [unwired: 1 in]
        n536 = Equal?(x="language", y=enum32{"PT", "EN", "NONE"}."NONE" ("language")) -> (x = y?=w1631:bool)
        n537 = Equal?(x="language", y=enum32{"PT", "EN", "NONE"}."PT" ("language")) -> (x = y?=w1630:bool)
        n538 = control-ref of="user permission"() -> (w1649:refnum<vi>)
        n539 = control-ref of="user previous"() -> (w1656:refnum<vi>)
        n540 = control-ref of="user next"() -> (w1645:refnum<vi>)
        n541 = control-ref of="user delete"() -> (w1646:refnum<vi>)
        n542 = control-ref of="user insert"() -> (w1648:refnum<vi>)
        n543 = control-ref of="change permission"() -> (w1650:refnum<vi>)
        n544 = control-ref of="email enable"() -> (w1652:refnum<vi>)
        n545 = control-ref of="auto logout"() -> (w1651:refnum<vi>)
        n546 = control-ref of="user name"() -> (w1647:refnum<vi>)
        n547 = control-ref of="email service"() -> (w1653:refnum<vi>)
        n548 = control-ref of="admin email"() -> (w1654:refnum<vi>)
        n549 = control-ref of="maint. email"() -> (w1655:refnum<vi>)
        n550 = Build Array(w1656, w1645, w1646, w1647, w1648, w1649, w1650, w1651, w1652, w1653, w1654, w1655) -> (w1657:refnum<vi>[])
        n551 = Insert Into Array(array=w1644, new element=w1657) -> (w1641:refnum<vi>[])  [unwired: 1 in]
        n552 = Insert Into Array(array=w1641, new element=w1643) -> (w1640:refnum<vi>[])  [unwired: 1 in]
        n553 = for {
          tunnel: w1640 -> [w1695] mode=indexing
          tunnel: "tips" -> [w1694] mode=indexing
          tunnel: w1630 -> [w1692]
          tunnel: w1631 -> [w1689]
          n554 = Unbundle By Name(w1694) -> ("PT"=w1691:string, "EN"=w1693:string)
          n555 = Select(t=w1691, s=w1692, f=w1693) -> (s? t:f=w1687:string)
          n556 = Select(t="", s=w1689, f=w1687) -> (s? t:f=w1690:string)
          n557 = property class="Ctl"(reference=w1695, "TipStrip"=w1690) -> ()  [unwired: 1 in, 2 out]
        }
      }
      event "comm help": Value Change {
        n558 = event-data() -> ()  [unwired: 1 in, 6 out]
        n559 = call "Help communication.vi"() -> ()  [unwired: 12 in]
      }
      event "login": Value Change {
        # "DO NOT OPEN\nPOPUP WHEN\nSERVER IS ON."
        n560 = event-data() -> ()  [unwired: 1 in, 3 out]
        n561 = local read "user list"() -> (w1707:T4)
        n562 = local read "server"() -> (w1704:bool)
        n563 = Not(x=w1704) -> (.not. x?=w1703:bool)
        n564 = call "Check id.vi"("password"="loginPW", "user name"="loginUser", "users in"=w1707) -> ("id ok"=w1711:bool, "first access"=w1702:bool, "users out"=w1700:T4, "permission"=w1715:string)  [unwired: 5 in]
        n565 = And(x=w1702, y=w1703) -> (x .and. y?=w1701:bool)
        n566 = case shown="False" w1701 {
          selector: w1701 -> [w1735 _]
          tunnel: "CONTINUE?" -> [_ w1739]
          tunnel: "Esta será sua senha\npermanente.\n\nYour password will\nbecome permanent." -> [_ w1738]
          tunnel: [w1736 w1737] -> w1710
          tunnel: w1711 -> [w1736 _]
          tunnel: [w1735 w1737] -> w1709
          frame False {
          }
          frame True {
            n567 = Two Button Dialog(message=w1738, 2:w1739) -> (T button?=w1737:bool)  [unwired: 1 in]
          }
        }
        n568 = case shown="True" w1709 {
          tunnel: w1699 -> [w1719 w1731]
          tunnel: [w1719 w1728] -> w1713
          tunnel: [w1718 w1727] -> w1712
          tunnel: w1698 -> [w1718 w1723]
          tunnel: w1700 -> [_ w1720]
          frame False {
            # "USER ALREADY HAS PASSWORD"
          }
          frame True {
            # "1st USER ACCESS: SAVE PASSWORD"
            n569 = local read "cfgFile"() -> (w1725:string)
            n570 = local write "user list"(w1720) -> ()
            n571 = call "Get attributes.vi"("error in (no error)"=w1723, "ICS in"=w1731) -> ("error out"=w1729:errorcluster, "email settings"=w1722:T10, "control indices"=w1730:i32[], "ICS out"=w1728:refnum<class "ICS.lvclass">)  [unwired: 6 in]
            n572 = call "Get date.vi"() -> ("date/time string"=w1721:string)  [unwired: 3 in]
            n573 = call <vilib>:"Application Directory.vi"() -> ("Application Directory"=w1726:path)
            n574 = Get Control Values by Index(1:w1730, 3:w1729) -> (10:w1732:variant[], 11:w1734:errorcluster)  [unwired: 1 in]
            n575 = Build Path(base path=w1726, name or relative path=w1725) -> (appended path=w1724:path)
            n576 = local write "last cfg date"(w1721) -> ()
            n577 = call "Config file.vi"("path"=w1724, "access (0:read/write)"=enum16{"read/write", "read-only", "write-only"}."write-only", "error in (no error)"=w1734, "data values"=w1732, "email settings"=w1722) -> ("error out"=w1727:errorcluster)  [unwired: 5 in, 1 out]
          }
        }
        n578 = case shown="True" w1710 {
          tunnel: w1715 -> [_ w1751]
          tunnel: w1713 -> [w1740 w1743]
          tunnel: [w1741 w1745] -> w1716
          tunnel: w1712 -> [w1741 w1746]
          tunnel: [w1740 w1744] -> w1717
          tunnel: "loginUser" -> [_ w1742]
          frame False {
            n579 = call <vilib>:"Beep.vi"() -> ()  [unwired: 12 in]
          }
          frame True {
            w1753 = T12."Disabled and Grayed Out" ("Disabled")
            w1754 = T12."Enabled" ("Disabled")
            # "USER CREDENTIALS ARE CORRECT"
            n580 = local read "server"() -> (w1764:bool)
            n581 = Equal?(x="Control", y=w1751) -> (x = y?=w1757:bool)
            n582 = Not Equal?(x=w1742, y="S4ICS") -> (x != y?=w1756:bool)
            n583 = Select(t=T6."Running" ("tab menu"), s=w1764, f=T6."Stopped" ("tab menu")) -> (s? t:f=w1761:T6)
            n584 = Equal?(x="Admin", y=w1751) -> (x = y?=w1765:bool)
            n585 = And(x=w1757, y=w1756) -> (x .and. y?=w1755:bool)
            n586 = call "Write current user.vi"("error in (no error)"=w1746, "current user"=w1742, "ICS in"=w1743) -> ("error out"=w1745:errorcluster, "ICS out"=w1744:refnum<class "ICS.lvclass">)  [unwired: 7 in]
            n587 = local write "tab menu"(w1761) -> ()
            n588 = local write "tab body"(enum32{"Motors", "Config"}."Motors" ("tab body")) -> ()
            n589 = Select(t=w1754, s=w1755, f=w1753) -> (s? t:f=w1766:T12)
            n590 = Select(t=w1754, s=w1765, f=w1753) -> (s? t:f=w1759:T12)
            n591 = Select(t=w1754, s=w1756, f=w1753) -> (s? t:f=w1758:T12)
            n592 = Build Array(0) -> (w1762:i32[])
            n593 = property on="setup" class="Bool"("DisabledEnum"=w1759) -> ()  [unwired: 2 in, 2 out]
            n594 = property on="control" class="Bool"("DisabledEnum"=w1766) -> ()  [unwired: 2 in, 2 out]
            n595 = property on="start server" class="Bool"("DisabledEnum"=w1758) -> ()  [unwired: 2 in, 2 out]
            n596 = property on="assist" class="Bool"("DisabledEnum"=w1758) -> ()  [unwired: 2 in, 2 out]
            n597 = property on="user list" class="Arr (strict)"("Index Values"=w1762) -> ()  [unwired: 2 in, 2 out]
          }
        }
      }
      event "logout running": Value Change {
        w1772 = ""
        n598 = event-data() -> ()  [unwired: 1 in, 6 out]
        n599 = local read "server"() -> (w1767:bool)
        n600 = local write "tab menu"(T6."Login" ("tab menu")) -> ()
        n601 = local write "tab body"(enum32{"Motors", "Config"}."Motors" ("tab body")) -> ()
        n602 = local write "loginPW"(w1772) -> ()
        n603 = local write "loginUser"(w1772) -> ()
        n604 = Not(x=w1767) -> (.not. x?=w1771:bool)
        n605 = property on="exitLogin" class="Bool"("Visible"=w1771) -> ()  [unwired: 2 in, 2 out]
        n606 = property on="loginUser" class="Str"("Key Focus"=TRUE) -> ()  [unwired: 2 in, 2 out]
      }
      event "logout stopped": Value Change {
        w1780 = ""
        n607 = event-data() -> ()  [unwired: 1 in, 6 out]
        n608 = local read "server"() -> (w1775:bool)
        n609 = local write "tab menu"(T6."Login" ("tab menu")) -> ()
        n610 = local write "tab body"(enum32{"Motors", "Config"}."Motors" ("tab body")) -> ()
        n611 = local write "loginPW"(w1780) -> ()
        n612 = local write "loginUser"(w1780) -> ()
        n613 = Not(x=w1775) -> (.not. x?=w1779:bool)
        n614 = property on="exitLogin" class="Bool"("Visible"=w1779) -> ()  [unwired: 2 in, 2 out]
        n615 = property on="loginUser" class="Str"("Key Focus"=TRUE) -> ()  [unwired: 2 in, 2 out]
      }
      event "stop server": Value Change {
        w1814 = FALSE
        w1813 = TRUE
        # "IF FIRST USER ACCESS (NO PASSWORD), RETURN TO LOGIN INSTEAD OF STOPPED MENU PAGE."
        n616 = event-data() -> ()  [unwired: 1 in, 1 out]
        n617 = local read "user list"() -> (w1821:T4)
        n618 = call "Read current user.vi"("error in (no error)"=w1822, "ICS in"=w1823) -> ("error out"=w1797:errorcluster, "current user"=w1820:string, "ICS out"=w1796:refnum<class "ICS.lvclass">)  [unwired: 7 in]
        n619 = property on="GFOC Value" class="DigNum (strict)"("Visible"=w1813) -> ()  [unwired: 2 in, 2 out]
        n620 = property on="WPROT Value" class="DigNum (strict)"("Visible"=w1813) -> ()  [unwired: 2 in, 2 out]
        n621 = property on="wprot stat" class="Clust (strict)"("Visible"=w1814) -> ()  [unwired: 2 in, 2 out]
        n622 = property on="wpsel stat" class="Clust (strict)"("Visible"=w1814) -> ()  [unwired: 2 in, 2 out]
        n623 = for {
          tunnel: w1821 -> [w1878] mode=indexing
          tunnel: w1820 -> [w1876]
          tunnel: [w1873] -> w1818
          stop <- w1872 stop-if-true
          n624 = Unbundle By Name(w1878) -> ("name"=w1877:string, "password"=w1875:string)  [unwired: 1 out]
          n625 = Equal?(x=w1877, y=w1876) -> (x = y?=w1872:bool)
          n626 = Empty String/Path?(string/path=w1875) -> (empty?=w1874:bool)
          n627 = And(x=w1874, y=w1872) -> (x .and. y?=w1873:bool)
        }
        n628 = property on="asel stat" class="Clust (strict)"("Visible"=w1814) -> ()  [unwired: 2 in, 2 out]
        n629 = property on="calw stat" class="Clust (strict)"("Visible"=w1814) -> ()  [unwired: 2 in, 2 out]
        n630 = property on="GMIR Value" class="DigNum (strict)"("Visible"=w1813) -> ()  [unwired: 2 in, 2 out]
        n631 = property on="WPSEL Value" class="DigNum (strict)"("Visible"=w1813) -> ()  [unwired: 2 in, 2 out]
        n632 = property on="gmir stat" class="Clust (strict)"("Visible"=w1814) -> ()  [unwired: 2 in, 2 out]
        n633 = property on="gfoc stat" class="Clust (strict)"("Visible"=w1814) -> ()  [unwired: 2 in, 2 out]
        n634 = property on="CALW Value" class="DigNum (strict)"("Visible"=w1813) -> ()  [unwired: 2 in, 2 out]
        n635 = property on="ASEL Value" class="DigNum (strict)"("Visible"=w1813) -> ()  [unwired: 2 in, 2 out]
        n636 = call-dynamic "Read Messenger.vi"("error in (no error)"=w1797, "ICS in"=w1796) -> ("error out"=w1791:errorcluster, "Messenger.lvclass"=w1792:refnum<class "Messenger.lvclass">, "ICS out"=w1793:refnum<class "ICS.lvclass">)  [unwired: 7 in]
        n637 = Select(t=T6."Login" ("tab menu"), s=w1818, f=T6."Stopped" ("tab menu")) -> (s? t:f=w1815:T6)
        n638 = flat-sequence {
          tunnel: w1793 -> [w1836]
          tunnel: w1792 -> [w1840]
          tunnel: w1791 -> [w1839]
          tunnel: T18 {"Message"="exit", "Message Data"=variant} ("message") -> [w1835]
          tunnel: [w1838] -> w1788
          tunnel: [w1837] -> w1787
          tunnel: [w1836] -> w1786
          tunnel: [u32 250 ("milliseconds to wait")] -> w1785
          tunnel: [w1842] -> w1790
          tunnel: [w1843] -> w1784
          tunnel: [w1844] -> w1783
          tunnel: w1788 -> [w1844]
          tunnel: w1787 -> [w1843]
          tunnel: w1786 -> [w1842]
          tunnel: w1785 -> [w1841]
          frame #0 {
            n639 = call-dynamic "Send message.vi"("error in (no error)"=w1839, "message"=w1835, "Messenger in"=w1840) -> ("error out"=w1838:errorcluster, "Messenger out"=w1837:refnum<class "Messenger.lvclass">)  [unwired: 7 in]
          }
          frame #1 {
            n640 = Wait (ms)(milliseconds to wait=w1841) -> ()  [unwired: 1 out]
          }
        }
        n641 = local write "tab menu"(w1815) -> ()
        n642 = local write "tab body"(enum32{"Motors", "Config"}."Motors" ("tab body")) -> ()
        n643 = local write "server"(FALSE) -> ()
        n644 = property on="login help" class="Bool"("DisabledEnum"=T12."Enabled" ("Disabled")) -> ()  [unwired: 2 in, 2 out]
        n645 = disable-structure shown="Disabled" {
          disable-tunnel: [w1831 w1833] -> w1795
          disable-tunnel: [w1830 w1832] -> w1794
          disable-tunnel: w1784 -> [w1829 w1832]
          disable-tunnel: w1783 -> [w1826 w1833]
          frame Disabled {
            n646 = call-dynamic "Destroy queues.vi"("error in (no error)"=w1826, "Messenger in"=w1829) -> ("error out"=w1827:errorcluster, "Messenger out"=w1828:refnum<class "Messenger.lvclass">)  [unwired: 8 in]
            n647 = call-dynamic "Stop 0mqComm.vi"("error in (no error)"=w1827, "Messenger in"=w1828) -> ("error out"=w1831:errorcluster, "Messenger out"=w1830:refnum<class "Messenger.lvclass">)  [unwired: 8 in]
          }
          frame Enabled {
            # "20240619"
          }
        }
        n648 = local read "channel"() -> (w1805:T5)
        n649 = Equal?(x=w1805, y=T5."Inner TCP/IP" ("channel")) -> (x = y?=w1804:bool)
        n650 = case shown="False" w1804 {
          tunnel: w1795 -> [w1850 w1863]
          tunnel: [w1849 w1861] -> w1801
          tunnel: [w1848 w1860] -> w1802
          tunnel: w1790 -> [w1847 w1862]
          tunnel: w1794 -> [w1846 w1859]
          tunnel: [w1845 w1859] -> w1798
          frame False {
            # "CLOSE INTERCOMM VI"
            n651 = disable-structure shown="Enabled" {
              disable-tunnel: w1850 -> [w1851 w1857]
              disable-tunnel: [w1854 w1857] -> w1849
              disable-tunnel: [w1855 w1858] -> w1848
              disable-tunnel: w1847 -> [w1855 w1858]
              disable-tunnel: w1846 -> [w1853 w1856]
              disable-tunnel: [w1852 w1856] -> w1845
              frame Enabled {
                n652 = call-dynamic "Stop InterComm.vi"("error in (no error)"=w1851, "Messenger in"=w1853) -> ("error out"=w1854:errorcluster, "Messenger out"=w1852:refnum<class "Messenger.lvclass">)  [unwired: 8 in]
              }
              frame Disabled {
              }
            }
          }
          frame True {
            # "CLOSE INNER TCP/IP CONNECTION"
            n653 = call "Read Server.vi"("error in (no error)"=w1863, "ICS in"=w1862) -> ("error out"=w1864:errorcluster, "Server"=w1866:refnum<class "TCP-Server.lvclass">, "ICS out"=w1860:refnum<class "ICS.lvclass">)  [unwired: 7 in]
            n654 = call "Read listenner.vi"("error in (no error)"=w1864, "Server in"=w1866) -> ("error out"=w1865:errorcluster, "listenner ID"=w1867:refnum<k5>)  [unwired: 7 in, 1 out]
            n655 = TCP Close Connection(connection ID=w1867, error in (no error)=w1865) -> (error out=w1861:errorcluster)  [unwired: 1 in, 1 out]
          }
        }
        n656 = call-dynamic "Write Messenger.vi"("error in (no error)"=w1801, "Messenger.lvclass"=w1798, "ICS in"=w1802) -> ("error out"=w1800:errorcluster, "ICS out"=w1799:refnum<class "ICS.lvclass">)  [unwired: 7 in]
        n657 = call-dynamic "Read motors.vi"("error in (no error)"=w1800, "ICS in"=w1799) -> ("error out"=w1812:errorcluster, "motors"=w1811:refnum<class "Motor.lvclass">[], "ICS out"=w1810:refnum<class "ICS.lvclass">)  [unwired: 7 in]
        n658 = for {
          tunnel: w1811 -> [w1868] mode=indexing
          tunnel: [w1869] -> w1808 mode=indexing
          shift-right: [w1870] -> w1809
          shift-left: w1812 -> [w1871]
          n659 = call-dynamic "Condition disabled to none.vi"("error in (no error)"=w1871, "Motor in"=w1868) -> ("error out"=w1870:errorcluster, "Motor out"=w1869:refnum<class "Motor.lvclass">)  [unwired: 8 in]
        }
        n660 = call-dynamic "Write motors.vi"("error in (no error)"=w1809, "motors"=w1808, "ICS in"=w1810) -> ("error out"=w1807:errorcluster, "ICS out"=w1806:refnum<class "ICS.lvclass">)  [unwired: 7 in]
      }
      event "start server": Value Change; User Event {
        n661 = event-data() -> ()  [unwired: 1 in, 3 out]
        n662 = local read "0mqEndpoint"() -> (w1880:string)
        n663 = local read "pubTime0mq"() -> (w1881:i32)
        n664 = call-dynamic "Read Messenger.vi"("error in (no error)"=w1897, "ICS in"=w1898) -> ("error out"=w1894:errorcluster, "Messenger.lvclass"=w1895:refnum<class "Messenger.lvclass">, "ICS out"=w1896:refnum<class "ICS.lvclass">)  [unwired: 7 in]
        n665 = Equal?(x="channel", y=T5."Inner TCP/IP" ("channel")) -> (x = y?=w1920:bool)
        n666 = Bundle(cluster=T19 {"channel"=enum."Local Panel", "address"="", "port"=0, "timeout"=0} ("channel configuration"), "channel"="channel", "address"=w1880, "port"=u16 0, "timeout"=w1881) -> (w1882:T19)
        n667 = disable-structure shown="Enabled" {
          disable-tunnel: w1895 -> [w1951 w1953]
          disable-tunnel: w1894 -> [w1950 w1952]
          disable-tunnel: "timeout" -> [w1949 _]
          disable-tunnel: [w1947 w1953] -> w1884
          disable-tunnel: [w1946 w1952] -> w1883
          disable-tunnel: w1882 -> [w1944 _]
          frame Disabled {
            n668 = call-dynamic "Create queues.vi"("error in (no error)"=w1950, "timeout"=w1949, "Messenger in"=w1951) -> ("error out"=w1945:errorcluster, "Messenger out"=w1948:refnum<class "Messenger.lvclass">)  [unwired: 7 in]
            n669 = call-dynamic "Run 0mqComm.vi"("error in (no error)"=w1945, "show FP"=FALSE, "channel configuration"=w1944, "Messenger in"=w1948) -> ("error out"=w1946:errorcluster, "Messenger out"=w1947:refnum<class "Messenger.lvclass">)  [unwired: 6 in]
          }
          frame Enabled {
            # "20240619"
          }
        }
        n670 = case shown="True" w1920 {
          tunnel: w1896 -> [w1976 w1998]
          tunnel: w1883 -> [w1975 w1999]
          tunnel: [w1974 w1997] -> w1892
          tunnel: [w1973 w2000] -> w1891
          tunnel: "address" -> [w1972 w1996]
          tunnel: "port" -> [w1971 w1995]
          tunnel: "timeout" -> [w1970 w1994]
          tunnel: "channel" -> [w1969 _]
          tunnel: w1884 -> [w1968 w1993]
          tunnel: [w1967 w1993] -> w1888
          frame False {
            # "START (RUN) INTERCOMM VI"
            n671 = disable-structure shown="Enabled" {
              disable-tunnel: w1976 -> [w1986 w1992]
              disable-tunnel: w1975 -> [w1984 w1991]
              disable-tunnel: [w1986 w1992] -> w1974
              disable-tunnel: [w1978 w1991] -> w1973
              disable-tunnel: w1972 -> [w1989 _]
              disable-tunnel: w1971 -> [w1988 _]
              disable-tunnel: w1970 -> [w1987 _]
              disable-tunnel: w1969 -> [w1982 _]
              disable-tunnel: w1968 -> [w1979 w1990]
              disable-tunnel: [w1977 w1990] -> w1967
              frame Enabled {
                n672 = Bundle(cluster=T19 {"channel"=enum."Local Panel", "address"="", "port"=0, "timeout"=0} ("channel configuration"), "channel"=w1982, "address"=w1989, "port"=w1988, "timeout"=w1987) -> (w1985:T19)
                n673 = Equal?(x=w1982, y=T5."Local Panel" ("channel")) -> (x = y?=w1980:bool)
                n674 = call-dynamic "Run InterComm.vi"("error in (no error)"=w1984, "show FP"=w1980, "channel configuration"=w1985, "Messenger in"=w1979) -> ("error out"=w1978:errorcluster, "Messenger out"=w1977:refnum<class "Messenger.lvclass">)  [unwired: 6 in]
              }
              frame Disabled {
              }
            }
          }
          frame True {
            # "CREATE LISTENNER FOR INNER TCP/IP CONNECTION"
            n675 = call "Read Server.vi"("error in (no error)"=w1999, "ICS in"=w1998) -> ("error out"=w2012:errorcluster, "Server"=w2013:refnum<class "TCP-Server.lvclass">, "ICS out"=w2011:refnum<class "ICS.lvclass">)  [unwired: 7 in]
            n676 = call "Write socket.vi"("ms timeout listening"=w1994, "error in (no error)"=w2012, "port"=w1995, "ip"=w1996, "Server in"=w2013) -> ("error out"=w2005:errorcluster, "Server out"=w2006:refnum<class "TCP-Server.lvclass">)  [unwired: 5 in]
            n677 = String To IP(1:w1996) -> (0:w2001:u32)
            n678 = call "Read timeouts.vi"("error in (no error)"=w2005, "Server in"=w2006) -> ("error out"=w2003:errorcluster, "ms create listener"=w2002:i32, "Server out"=w2004:refnum<class "TCP-Server.lvclass">)  [unwired: 4 in, 3 out]
            n679 = TCP Create Listener(7:w2001, 8:w2003, 9:w2002, 10:w1995) -> (0:w2010:errorcluster, 3:w2009:refnum<k5>)  [unwired: 1 in, 1 out]
            n680 = call "Write listenner.vi"("error in (no error)"=w2010, "listenner ID"=w2009, "Server in"=w2004) -> ("error out"=w2007:errorcluster, "Server out"=w2008:refnum<class "TCP-Server.lvclass">)  [unwired: 7 in]
            n681 = call "Write Server.vi"("error in (no error)"=w2007, "Server"=w2008, "ICS in"=w2011) -> ("error out"=w2000:errorcluster, "ICS out"=w1997:refnum<class "ICS.lvclass">)  [unwired: 7 in]
          }
        }
        n682 = local read "S4ICS password"() -> (w1938:string)
        n683 = local read "email service"() -> (w1936:string)
        n684 = local read "email enable"() -> (w1937:bool)
        n685 = local read "maint. email"() -> (w1942:string)
        n686 = local read "admin email"() -> (w1941:string)
        n687 = local read "S4ICS email"() -> (w1940:string)
        n688 = local read "S4ICS login"() -> (w1939:string)
        n689 = call-dynamic "Write Messenger.vi"("error in (no error)"=w1891, "Messenger.lvclass"=w1888, "ICS in"=w1892) -> ("error out"=w1889:errorcluster, "ICS out"=w1890:refnum<class "ICS.lvclass">)  [unwired: 7 in]
        n690 = local read "WPROT disabled"() -> (w1927:bool)
        n691 = local read "WPSEL disabled"() -> (w1928:bool)
        n692 = local read "CALW disabled"() -> (w1909:bool)
        n693 = local read "GMIR disabled"() -> (w1926:bool)
        n694 = local read "ASEL disabled"() -> (w1908:bool)
        n695 = Bundle By Name(cluster=T10 {"email service"="", "maint. email"="", "admin email"="", "S4ICS email"="", "S4ICS login"="", "S4ICS password"="", "email enabled"=FALSE} ("email cluster"), "email service"=w1936, "maint. email"=w1942, "admin email"=w1941, "S4ICS email"=w1940, "S4ICS login"=w1939, "S4ICS password"=w1938, "email enabled"=w1937) -> (w1915:T10)
        n696 = Build Array("WPROT mode", "WPSEL mode", "CALW mode", "ASEL mode", "GMIR mode", "GFOC mode") -> (w1912:string[])
        n697 = Build Array("WPROT ip", "WPSEL ip", "CALW ip", "ASEL ip", "GMIR ip", "GMIR ip") -> (w1913:string[])
        n698 = Build Array(w1927, w1928, w1909, w1908, w1926, w1926) -> (w1914:bool[])
        n699 = call-dynamic "Write configuration.vi"("disabled flags"=w1914, "email settings"=w1915, "error in (no error)"=w1889, "setup ips"=w1913, "setup modes"=w1912, "ICS in"=w1890) -> ("error out"=w1904:errorcluster, "ICS out"=w1903:refnum<class "ICS.lvclass">)  [unwired: 4 in]
        n700 = case shown="No Error" w1904 {
          selector: w1904 -> [w1964 w1965]
          tunnel: [w1964 w1965] -> w1901
          tunnel: w1903 -> [w1954 w1966]
          tunnel: [w1954 w1966] -> w1902
          frame No Error {
            w1955 = T1 {"mode"="", "condition"="", "position"="", "pos_name"="", "pos_id"=""} ("status")
            w1956 = ""
            w1959 = FALSE
            w1960 = TRUE
            n701 = local write "wprot stat"(w1955) -> ()
            n702 = local write "wpsel stat"(w1955) -> ()
            n703 = property on="GFOC Value" class="DigNum (strict)"("Visible"=w1959) -> ()  [unwired: 2 in, 2 out]
            n704 = property on="WPROT Value" class="DigNum (strict)"("Visible"=w1959) -> ()  [unwired: 2 in, 2 out]
            n705 = property on="wprot stat" class="Clust (strict)"("Visible"=w1960) -> ()  [unwired: 2 in, 2 out]
            n706 = property on="wpsel stat" class="Clust (strict)"("Visible"=w1960) -> ()  [unwired: 2 in, 2 out]
            n707 = local write "loginPW"(w1956) -> ()
            n708 = local write "loginUser"(w1956) -> ()
            n709 = local write "tab menu"(T6."Login" ("tab menu")) -> ()
            n710 = local write "tab body"(enum32{"Motors", "Config"}."Motors" ("tab body")) -> ()
            n711 = local write "asel stat"(w1955) -> ()
            n712 = local write "calw stat"(w1955) -> ()
            n713 = property on="GMIR Value" class="DigNum (strict)"("Visible"=w1959) -> ()  [unwired: 2 in, 2 out]
            n714 = property on="WPSEL Value" class="DigNum (strict)"("Visible"=w1959) -> ()  [unwired: 2 in, 2 out]
            n715 = property on="asel stat" class="Clust (strict)"("Visible"=w1960) -> ()  [unwired: 2 in, 2 out]
            n716 = property on="calw stat" class="Clust (strict)"("Visible"=w1960) -> ()  [unwired: 2 in, 2 out]
            n717 = local write "gfoc stat"(w1955) -> ()
            n718 = local write "gmir stat"(w1955) -> ()
            n719 = property on="loginUser" class="Str"("Key Focus"=TRUE) -> ()  [unwired: 2 in, 2 out]
            n720 = property on="CALW Value" class="DigNum (strict)"("Visible"=w1959) -> ()  [unwired: 2 in, 2 out]
            n721 = property on="ASEL Value" class="DigNum (strict)"("Visible"=w1959) -> ()  [unwired: 2 in, 2 out]
            n722 = property on="login help" class="Bool"("DisabledEnum"=T12."Disabled" ("Disabled")) -> ()  [unwired: 2 in, 2 out]
            n723 = property on="gmir stat" class="Clust (strict)"("Visible"=w1960) -> ()  [unwired: 2 in, 2 out]
            n724 = property on="gfoc stat" class="Clust (strict)"("Visible"=w1960) -> ()  [unwired: 2 in, 2 out]
            n725 = property on="exitLogin" class="Bool"("Visible"=FALSE) -> ()  [unwired: 2 in, 2 out]
          }
          frame Error {
          }
        }
        n726 = call-dynamic "Read motors.vi"("error in (no error)"=w1901, "ICS in"=w1902) -> ("error out"=w1925:errorcluster, "motors"=w1899:refnum<class "Motor.lvclass">[], "ICS out"=w1918:refnum<class "ICS.lvclass">)  [unwired: 7 in]
        n727 = for {
          tunnel: w1899 -> [w2023] mode=indexing
          shift-right: [w2016] -> w1924
          shift-left: w1925 -> [w2022]
          tunnel: [w2018] -> w1923 mode=indexing
          tunnel: [TRUE ("server enabled")] -> w1900
          w2014 = "2" ("current code")
          # "CHECK COMMUNICATION AND STORE\nPREDEFINED POSITIONS OF EACH MOTOR"
          n728 = call-dynamic "Read status.vi"("error in (no error)"=w2022, "Motor in"=w2023) -> ("error out"=w2028:errorcluster, "name"=w2026:string, "status"=w2025:T1, "Motor out"=w2027:refnum<class "Motor.lvclass">)  [unwired: 6 in]
          n729 = case shown="\"WPROT\"" w2026 {
            tunnel: [w2033 w2036 w2041 w2043 w2049 w2052 w2057] -> w2031
            tunnel: [w2032 w2037 w2040 w2044 w2048 w2051 w2055] -> w2030
            tunnel: w2028 -> [w2032 w2037 w2040 w2044 w2048 w2051 w2055]
            tunnel: w2027 -> [w2033 w2036 w2041 w2043 w2049 w2052 w2057]
            tunnel: [_ "WPROT positions" "WPSEL positions" "CALW positions" "ASEL positions" "GMIR positions" "GFOC positions"] -> w2029
            tunnel: w2025 -> [_ w2035 w2038 w2042 w2046 w2050 w2054]
            frame "", Default {
            }
            frame "WPROT" {
              n730 = local write "wprot stat"(w2035) -> ()
            }
            frame "WPSEL" {
              n731 = local write "wpsel stat"(w2038) -> ()
            }
            frame "CALW" {
              n732 = local write "calw stat"(w2042) -> ()
            }
            frame "ASEL" {
              n733 = local write "asel stat"(w2046) -> ()
            }
            frame "GMIR" {
              n734 = local write "gmir stat"(w2050) -> ()
            }
            frame "GFOC" {
              n735 = local write "gfoc stat"(w2054) -> ()
            }
          }
          n736 = local read "enabled log"() -> (w2015:string)
          n737 = call-dynamic "Write predef positions.vi"("error in (no error)"=w2030, "predef positions"=w2029, "Motor in"=w2031) -> ("error out"=w2020:errorcluster, "Motor out"=w2021:refnum<class "Motor.lvclass">)  [unwired: 7 in]
          n738 = call-dynamic "Validate motor.vi"("current code"=w2014, "enabled codes"=w2015, "error in (no error)"=w2020, "Motor in"=w2021) -> ("error out"=w2017:errorcluster, "Motor out"=w2019:refnum<class "Motor.lvclass">)  [unwired: 6 in]
          n739 = call-dynamic "Send positions to motor.vi"("current code"=w2014, "enabled codes"=w2015, "error in (no error)"=w2017, "Motor in"=w2019) -> ("error out"=w2016:errorcluster, "Motor out"=w2018:refnum<class "Motor.lvclass">)  [unwired: 6 in]
        }
        n740 = local write "server"(w1900) -> ()
        n741 = call-dynamic "Write motors.vi"("error in (no error)"=w1924, "motors"=w1923, "ICS in"=w1918) -> ("error out"=w1916:errorcluster, "ICS out"=w1917:refnum<class "ICS.lvclass">)  [unwired: 7 in]
      }
      event "exitLogin": Value Change {
        w2066 = "exitLogin" ("Message")
        # "THE 0MQ MANAGER EXITS WHEN A EXIT MESSAGE IS READ FROM THE QUEUE"
        n742 = event-data() -> ()  [unwired: 1 in, 6 out]
        n743 = call-dynamic "Read Messenger.vi"("error in (no error)"=w2062, "ICS in"=w2063) -> ("error out"=w2073:errorcluster, "Messenger.lvclass"=w2072:refnum<class "Messenger.lvclass">, "ICS out"=w2068:refnum<class "ICS.lvclass">)  [unwired: 7 in]
        n744 = Bundle By Name(cluster=T18 {"Message"="", "Message Data"=variant} ("message"), "Message"="exit", "Message Data"=w2066) -> (w2071:T18)
        n745 = call-dynamic "Write last status.vi"("error in (no error)"=w2073, "last status"=w2066, "Messenger in"=w2072) -> ("error out"=w2069:errorcluster, "Messenger out"=w2070:refnum<class "Messenger.lvclass">)  [unwired: 7 in]
        n746 = call-dynamic "Send message.vi"("error in (no error)"=w2069, "message"=w2071, "Messenger in"=w2070) -> ("error out"=w2067:errorcluster, "Messenger out"=w2059:refnum<class "Messenger.lvclass">)  [unwired: 7 in]
        n747 = call-dynamic "Write Messenger.vi"("error in (no error)"=w2067, "Messenger.lvclass"=w2059, "ICS in"=w2068) -> ("error out"=w2061:errorcluster, "ICS out"=w2060:refnum<class "ICS.lvclass">)  [unwired: 7 in]
      }
      event "exitStopped": Value Change {
        w2080 = "exitStopped" ("Message")
        # "THE 0MQ MANAGER EXITS WHEN A EXIT MESSAGE IS READ FROM THE QUEUE"
        n748 = event-data() -> ()  [unwired: 1 in, 1 out]
        n749 = call-dynamic "Read Messenger.vi"("error in (no error)"=w2088, "ICS in"=w2089) -> ("error out"=w2087:errorcluster, "Messenger.lvclass"=w2086:refnum<class "Messenger.lvclass">, "ICS out"=w2079:refnum<class "ICS.lvclass">)  [unwired: 7 in]
        n750 = Bundle By Name(cluster=T18 {"Message"="", "Message Data"=variant} ("message"), "Message"="exit", "Message Data"=w2080) -> (w2083:T18)
        n751 = call-dynamic "Write last status.vi"("error in (no error)"=w2087, "last status"=w2080, "Messenger in"=w2086) -> ("error out"=w2081:errorcluster, "Messenger out"=w2082:refnum<class "Messenger.lvclass">)  [unwired: 7 in]
        n752 = call-dynamic "Send message.vi"("error in (no error)"=w2081, "message"=w2083, "Messenger in"=w2082) -> ("error out"=w2078:errorcluster, "Messenger out"=w2075:refnum<class "Messenger.lvclass">)  [unwired: 7 in]
        n753 = call-dynamic "Write Messenger.vi"("error in (no error)"=w2078, "Messenger.lvclass"=w2075, "ICS in"=w2079) -> ("error out"=w2077:errorcluster, "ICS out"=w2076:refnum<class "ICS.lvclass">)  [unwired: 7 in]
      }
      event "assist": Value Change {
        n754 = event-data() -> ()  [unwired: 1 in, 6 out]
        n755 = local write "tab menu"(T6."Assist" ("tab menu")) -> ()
        n756 = local write "tab body"(enum32{"Motors", "Config"}."Motors" ("tab body")) -> ()
      }
      event "return assist": Value Change {
        # "Set assist motor selector\nto \"No selection\".\nRequired by animation."
        n757 = event-data() -> ()  [unwired: 1 in, 6 out]
        n758 = call "Write motor IP.vi"("error in (no error)"=w2098, "motor IP"="", "ICS in"=w2097) -> ("error out"=w2096:errorcluster, "ICS out"=w2095:refnum<class "ICS.lvclass">)  [unwired: 7 in]
        n759 = local write "tab menu"(T6."Stopped" ("tab menu")) -> ()
        n760 = local write "tab body"(enum32{"Motors", "Config"}."Motors" ("tab body")) -> ()
      }
      event "setup": Value Change {
        n761 = event-data() -> ()  [unwired: 1 in, 6 out]
        n762 = stacked-sequence {
          frame #0 {
            # "SET TAB PAGES AND ADJUST CONTROLS"
            n763 = local write "user name"("") -> ()
            n764 = local write "email ok"(FALSE) -> ()
            n765 = local write "tab menu"(T6."Setup" ("tab menu")) -> ()
            n766 = local write "tab body"(enum32{"Motors", "Config"}."Config" ("tab body")) -> ()
            n767 = property on="email ok" class="Bool (strict)"("DisabledEnum"=T12."Disabled and Grayed Out" ("Disabled")) -> ()  [unwired: 2 in, 2 out]
          }
          frame #1 {
            # "DISABLE PM PWR CONTROLS BASED ON MAINS STATE"
            n768 = local read "pwrPM mains"() -> (w2111:bool)
            n769 = Select(t=T12."Disabled and Grayed Out" ("Disabled"), s=w2111, f=T12."Enabled" ("Disabled")) -> (s? t:f=w2110:T12)
            n770 = property on="pwrPM ip" class="Str"("DisabledEnum"=w2110) -> ()  [unwired: 2 in, 2 out]
            n771 = property on="pwrPM port" class="DigNum (strict)"("DisabledEnum"=w2110) -> ()  [unwired: 2 in, 2 out]
            n772 = property on="pwrPM user" class="Str"("DisabledEnum"=w2110) -> ()  [unwired: 2 in, 2 out]
            n773 = property on="pwrPM password" class="Str"("DisabledEnum"=w2110) -> ()  [unwired: 2 in, 2 out]
            n774 = property on="pwrPM outlet" class="DigNum (strict)"("DisabledEnum"=w2110) -> ()  [unwired: 2 in, 2 out]
          }
          frame #2 {
            # "DISABLE GD PWR CONTROLS BASED ON MAINS STATE"
            n775 = local read "pwrGD mains"() -> (w2115:bool)
            n776 = Select(t=T12."Disabled and Grayed Out" ("Disabled"), s=w2115, f=T12."Enabled" ("Disabled")) -> (s? t:f=w2114:T12)
            n777 = property on="pwrGD ip" class="Str"("DisabledEnum"=w2114) -> ()  [unwired: 2 in, 2 out]
            n778 = property on="pwrGD port" class="DigNum (strict)"("DisabledEnum"=w2114) -> ()  [unwired: 2 in, 2 out]
            n779 = property on="pwrGD user" class="Str"("DisabledEnum"=w2114) -> ()  [unwired: 2 in, 2 out]
            n780 = property on="pwrGD password" class="Str"("DisabledEnum"=w2114) -> ()  [unwired: 2 in, 2 out]
            n781 = property on="pwrGD outlet" class="DigNum (strict)"("DisabledEnum"=w2114) -> ()  [unwired: 2 in, 2 out]
          }
        }
      }
      event "save config": Value Change {
        n782 = event-data() -> ()  [unwired: 1 in, 6 out]
        n783 = local read "user list"() -> (w2123:T4)
        n784 = local read "last cfg date"() -> (w2128:string)
        n785 = local read "cfgFile"() -> (w2121:string)
        n786 = local read "last cfg user"() -> (w2127:string)
        n787 = call "Read current user.vi"("error in (no error)"=w2132, "ICS in"=w2131) -> ("error out"=w2125:errorcluster, "current user"=w2126:string, "ICS out"=w2130:refnum<class "ICS.lvclass">)  [unwired: 7 in]
        n788 = Empty String/Path?(string/path=w2121) -> (empty?=w2120:bool)
        n789 = call "Check admin.vi"("users in"=w2123) -> ("admin user?"=w2119:bool, "users out"=w2124:T4)  [unwired: 8 in, 1 out]
        n790 = case shown="False" w2120 {
          tunnel: w2121 -> [w2134 _]
          tunnel: [w2134 w2136] -> w2117
          tunnel: [TRUE ("valid name") w2135] -> w2116
          frame False {
          }
          frame True {
            n791 = call "Input name.vi"() -> ("file name"=w2136:string, "valid name"=w2135:bool)  [unwired: 9 in, 1 out]
          }
        }
        n792 = And(x=w2119, y=w2116) -> (x .and. y?=w2118:bool)
        n793 = case shown="True" w2118 {
          tunnel: [w2138 w2166] -> w2122
          tunnel: w2130 -> [w2139 w2157]
          tunnel: [w2139 w2164] -> w2129
          tunnel: w2124 -> [_ w2155]
          tunnel: w2128 -> [_ w2163]
          tunnel: w2127 -> [_ w2156]
          tunnel: w2126 -> [_ w2154]
          tunnel: w2125 -> [w2138 w2153]
          tunnel: w2117 -> [_ w2146]
          tunnel: w2116 -> [w2137 _]
          frame False {
            n794 = case shown="True" w2137 {
              frame False {
              }
              frame True {
                n795 = local read "language"() -> (w2145:enum32{"PT", "EN", "NONE"})
                n796 = Not Equal?(x=w2145, y=enum32{"PT", "EN", "NONE"}."EN" ("language")) -> (x != y?=w2144:bool)
                n797 = Select(t="É exigido um usuário (diferente\nde S4ICS) com a permissão Admin." ("message"), s=w2144, f="There must be at least one \nuser (other than S4ICS)\nwith Admin permission." ("message")) -> (s? t:f=w2143:string)
                n798 = One Button Dialog(message=w2143) -> ()  [unwired: 1 in, 1 out]
              }
            }
          }
          frame True {
            n799 = call "Get date.vi"() -> ("date/time string"=w2150:string)  [unwired: 3 in]
            n800 = flat-sequence {
              tunnel: w2153 -> [w2170]
              tunnel: w2150 -> [w2169]
              tunnel: [w2170] -> w2158
              tunnel: w2155 -> [w2167]
              tunnel: w2154 -> [w2168]
              frame #0 {
                n801 = local write "last cfg date"(w2169) -> ()
                n802 = local write "last cfg user"(w2168) -> ()
                n803 = local write "user list"(w2167) -> ()
              }
            }
            n804 = local write "cfgFile"(w2146) -> ()
            n805 = call "Get attributes.vi"("error in (no error)"=w2158, "ICS in"=w2157) -> ("error out"=w2165:errorcluster, "email settings"=w2152:T10, "control indices"=w2160:i32[], "ICS out"=w2162:refnum<class "ICS.lvclass">)  [unwired: 6 in]
            n806 = call <vilib>:"Application Directory.vi"() -> ("Application Directory"=w2149:path)
            n807 = Get Control Values by Index(1:w2160, 3:w2165) -> (10:w2159:variant[], 11:w2151:errorcluster)  [unwired: 1 in]
            n808 = Build Path(base path=w2149, name or relative path=w2146) -> (appended path=w2148:path)
            n809 = call "Config file.vi"("path"=w2148, "access (0:read/write)"=enum16{"read/write", "read-only", "write-only"}."write-only", "error in (no error)"=w2151, "data values"=w2159, "email settings"=w2152) -> ("error out"=w2147:errorcluster)  [unwired: 5 in, 1 out]
            n810 = case shown="No Error" w2147 {
              selector: w2147 -> [w2173 w2179]
              tunnel: w2162 -> [w2174 w2189]
              tunnel: [w2174 w2189] -> w2164
              tunnel: [w2173 w2188] -> w2166
              tunnel: w2163 -> [_ w2187]
              tunnel: w2156 -> [_ w2186]
              frame No Error {
                w2178 = ""
                # "WRITE ALL CONFIG PARAMETERS"
                n811 = local read "server"() -> (w2171:bool)
                n812 = local write "loginUser"(w2178) -> ()
                n813 = local write "loginPW"(w2178) -> ()
                n814 = property on="loginUser" class="Str"("Key Focus"=TRUE) -> ()  [unwired: 2 in, 2 out]
                n815 = local write "tab menu"(T6."Login" ("tab menu")) -> ()
                n816 = local write "tab body"(enum32{"Motors", "Config"}."Motors" ("tab body")) -> ()
                n817 = Not(x=w2171) -> (.not. x?=w2176:bool)
                n818 = property on="exitLogin" class="Bool"("Visible"=w2176) -> ()  [unwired: 2 in, 2 out]
              }
              frame Error {
                n819 = local read "language"() -> (w2185:enum32{"PT", "EN", "NONE"})
                n820 = local write "last cfg user"(w2186) -> ()
                n821 = local write "last cfg date"(w2187) -> ()
                n822 = Not Equal?(x=w2185, y=enum32{"PT", "EN", "NONE"}."EN" ("language")) -> (x != y?=w2184:bool)
                n823 = Select(t="Falha ao salvar\na configuração." ("message"), s=w2184, f="Can't write the\nconfiguration." ("message")) -> (s? t:f=w2181:string)
                n824 = call <vilib>:"Clear Errors.vi"("error in (no error)"=w2179) -> ("error out"=w2188:errorcluster)  [unwired: 5 in, 1 out]
                n825 = One Button Dialog(message=w2181) -> ()  [unwired: 1 in, 1 out]
              }
            }
          }
        }
      }
      event "save as": Value Change {
        n826 = event-data() -> ()  [unwired: 1 in, 6 out]
        n827 = call "Input name.vi"() -> ("file name"=w2190:string, "valid name"=w2191:bool)  [unwired: 9 in, 1 out]
        n828 = case shown="True" w2191 {
          tunnel: w2195 -> [w2196 w2207]
          tunnel: w2194 -> [w2197 w2206]
          tunnel: [w2197 w2205] -> w2193
          tunnel: [w2196 w2204] -> w2192
          tunnel: w2190 -> [_ w2198]
          frame False {
          }
          frame True {
            n829 = local read "user list"() -> (w2209:T4)
            n830 = local read "last cfg date"() -> (w2203:string)
            n831 = local read "last cfg user"() -> (w2202:string)
            n832 = call "Read current user.vi"("error in (no error)"=w2207, "ICS in"=w2206) -> ("error out"=w2199:errorcluster, "current user"=w2201:string, "ICS out"=w2210:refnum<class "ICS.lvclass">)  [unwired: 7 in]
            n833 = call "Check admin.vi"("users in"=w2209) -> ("admin user?"=w2211:bool, "users out"=w2208:T4)  [unwired: 8 in, 1 out]
            n834 = case shown="True" w2211 {
              tunnel: [w2212 w2229] -> w2204
              tunnel: w2210 -> [w2214 w2230]
              tunnel: [w2214 w2228] -> w2205
              tunnel: w2208 -> [_ w2220]
              tunnel: w2198 -> [_ w2223]
              tunnel: w2203 -> [_ w2225]
              tunnel: w2202 -> [_ w2224]
              tunnel: w2201 -> [_ w2221]
              tunnel: "%Y-%m-%d %H:%M:%S" ("time format string (%c)") -> [_ w2219]
              tunnel: w2199 -> [w2212 w2218]
              frame False {
                n835 = One Button Dialog(message="THERE MUST BE AT LEAST ONE \nUSER (OTHER THAN S4ICS)\nWITH ADMIN PERMISSION.") -> ()  [unwired: 1 in, 1 out]
              }
              frame True {
                n836 = Format Date/Time String(time format string (%c)=w2219) -> (date/time string=w2233:string)  [unwired: 2 in]
                n837 = flat-sequence {
                  tunnel: w2218 -> [w2240]
                  tunnel: w2233 -> [w2241]
                  tunnel: [w2240] -> w2231
                  tunnel: w2221 -> [w2239]
                  tunnel: w2220 -> [w2238]
                  frame #0 {
                    n838 = local write "last cfg date"(w2241) -> ()
                    n839 = local write "last cfg user"(w2239) -> ()
                    n840 = local write "user list"(w2238) -> ()
                  }
                }
                n841 = call "Get attributes.vi"("error in (no error)"=w2231, "ICS in"=w2230) -> ("error out"=w2235:errorcluster, "email settings"=w2217:T10, "control indices"=w2232:i32[], "ICS out"=w2228:refnum<class "ICS.lvclass">)  [unwired: 6 in]
                n842 = call <vilib>:"Application Directory.vi"() -> ("Application Directory"=w2227:path)
                n843 = Build Path(base path=w2227, name or relative path=w2223) -> (appended path=w2226:path)
                n844 = Get Control Values by Index(1:w2232, 3:w2235) -> (10:w2222:variant[], 11:w2216:errorcluster)  [unwired: 1 in]
                n845 = call "Config file.vi"("path"=w2226, "access (0:read/write)"=enum16{"read/write", "read-only", "write-only"}."write-only", "error in (no error)"=w2216, "data values"=w2222, "email settings"=w2217) -> ("error out"=w2215:errorcluster)  [unwired: 5 in, 1 out]
                n846 = case shown="No Error" w2215 {
                  selector: w2215 -> [w2246 w2254]
                  tunnel: [w2246 w2253] -> w2229
                  frame No Error {
                    n847 = property on="user list" class="Arr (strict)"() -> ("Index Values"=w2243:u32[])  [unwired: 2 in, 2 out]
                    n848 = Replace Array Subset(array=w2243, new element=u32 0 ("index")) -> (w2244:u32[])  [unwired: 1 in]
                    n849 = property on="save config" class="Bool"("DisabledEnum"=T12."Enabled" ("Disabled")) -> ()  [unwired: 2 in, 2 out]
                    n850 = property on="user list" class="Arr (strict)"("Index Values"=w2244) -> ()  [unwired: 2 in, 2 out]
                  }
                  frame Error {
                    n851 = local read "language"() -> (w2250:enum32{"PT", "EN", "NONE"})
                    n852 = Not Equal?(x=w2250, y=enum32{"PT", "EN", "NONE"}."EN" ("language")) -> (x != y?=w2248:bool)
                    n853 = Select(t="Falha ao salvar\na configuração." ("message"), s=w2248, f="Can't write the\nconfiguration." ("message")) -> (s? t:f=w2249:string)
                    n854 = call <vilib>:"Clear Errors.vi"("error in (no error)"=w2254) -> ("error out"=w2253:errorcluster)  [unwired: 5 in, 1 out]
                    n855 = One Button Dialog(message=w2249) -> ()  [unwired: 1 in, 1 out]
                  }
                }
                n856 = flat-sequence {
                  tunnel: w2225 -> [w2237]
                  tunnel: w2224 -> [w2236]
                  tunnel: w2215 -> [_]
                  frame #0 {
                    # "PUT LAST NAMES BACK"
                    n857 = local write "last cfg date"(w2237) -> ()
                    n858 = local write "last cfg user"(w2236) -> ()
                  }
                }
              }
            }
          }
        }
      }
      event "config help": Value Change {
        n859 = event-data() -> ()  [unwired: 1 in, 6 out]
        n860 = call "Help setup.vi"() -> ()  [unwired: 12 in]
      }
      event "log help": Value Change {
        n861 = event-data() -> ()  [unwired: 1 in, 6 out]
        n862 = call "Help logger.vi"() -> ()  [unwired: 12 in]
      }
      event "WPROT disabled": Value Change {
        # "THIS EVENT WILL BE USED TO TURN MOTOR POWER ON/OFF"
        n863 = event-data() -> ()  [unwired: 1 in, 6 out]
      }
      event "WPSEL disabled": Value Change {
        # "THIS EVENT WILL BE USED TO TURN MOTOR POWER ON/OFF"
        n864 = event-data() -> ()  [unwired: 1 in, 6 out]
      }
      event "ASEL disabled": Value Change {
        # "THIS EVENT WILL BE USED TO TURN MOTOR POWER ON/OFF"
        n865 = event-data() -> ()  [unwired: 1 in, 6 out]
      }
      event "CALW disabled": Value Change {
        # "THIS EVENT WILL BE USED TO TURN MOTOR POWER ON/OFF"
        n866 = event-data() -> ()  [unwired: 1 in, 6 out]
      }
      event "GMIR disabled": Value Change {
        # "THIS EVENT WILL BE USED TO TURN MOTOR POWER ON/OFF"
        n867 = event-data() -> ()  [unwired: 1 in, 6 out]
      }
      event "user next": Value Change {
        n868 = event-data() -> ()  [unwired: 1 in, 6 out]
        n869 = local read "user list"() -> (w2274:T4)
        n870 = property on="user list" class="Arr (strict)"() -> ("Index Values"=w2270:u32[])  [unwired: 2 in, 2 out]
        n871 = Index Array(array=w2270) -> (element=w2273:u32)  [unwired: 1 in]
        n872 = Array Size(array=w2274) -> (size(s)=w2272:i32)
        n873 = Increment(x=w2273) -> (x+1=w2269:u32)
        n874 = Less?(x=w2269, y=w2272) -> (x < y?=w2271:bool)
        n875 = case shown="True" w2271 {
          tunnel: w2270 -> [_ w2279]
          tunnel: w2269 -> [_ w2278]
          frame False {
          }
          frame True {
            # "INCREMENT USER LIST INDEX"
            n876 = Replace Array Subset(array=w2279, new element=w2278) -> (w2277:u32[])  [unwired: 1 in]
            n877 = property on="user list" class="Arr (strict)"("Index Values"=w2277) -> ()  [unwired: 2 in, 2 out]
          }
        }
      }
      event "user previous": Value Change {
        n878 = event-data() -> ()  [unwired: 1 in, 6 out]
        n879 = property on="user list" class="Arr (strict)"() -> ("Index Values"=w2281:u32[])  [unwired: 2 in, 2 out]
        n880 = Index Array(array=w2281) -> (element=w2283:u32)  [unwired: 1 in]
        n881 = Decrement(x=w2283) -> (x-1=w2280:u32)
        n882 = Greater Or Equal To 0?(x=w2280) -> (x >= 0?=w2282:bool)
        n883 = case shown="True" w2282 {
          tunnel: w2281 -> [_ w2288]
          tunnel: w2280 -> [_ w2286]
          frame False {
          }
          frame True {
            # "DECREMENT USER LIST INDEX"
            n884 = Replace Array Subset(array=w2288, new element=w2286) -> (w2287:u32[])  [unwired: 1 in]
            n885 = property on="user list" class="Arr (strict)"("Index Values"=w2287) -> ()  [unwired: 2 in, 2 out]
          }
        }
      }
      event "user delete": Value Change {
        w2292 = 0 ("index")
        n886 = event-data() -> ()  [unwired: 1 in, 6 out]
        n887 = call "Read current user.vi"("error in (no error)"=w2304, "ICS in"=w2303) -> ("error out"=w2305:errorcluster, "current user"=w2289:string, "ICS out"=w2301:refnum<class "ICS.lvclass">)  [unwired: 7 in]
        n888 = local read "user list"() -> (w2299:T4)
        n889 = property on="user list" class="Arr (strict)"() -> ("Index Values"=w2293:u32[])  [unwired: 2 in, 2 out]
        n890 = local read "language"() -> (w2298:enum32{"PT", "EN", "NONE"})
        n891 = Index Array(array=w2293, index=w2292) -> (element=w2295:u32)
        n892 = Decrement(x=w2295) -> (x-1=w2294:u32)
        n893 = Index Array(array=w2299, index=w2295) -> (element=w2302:T20)
        n894 = Not Equal?(x=w2298, y=enum32{"PT", "EN", "NONE"}."EN" ("language")) -> (x != y?=w2297:bool)
        n895 = Unbundle By Name(w2302) -> ("name"=w2290:string)
        n896 = Replace Array Subset(array=w2293, new element=w2294, index=w2292) -> (w2291:u32[])
        n897 = Equal?(x=w2290, y=w2289) -> (x = y?=w2300:bool)
        n898 = case shown="False" w2300 {
          tunnel: w2299 -> [w2314 _]
          tunnel: w2295 -> [w2315 _]
          tunnel: w2290 -> [w2311 _]
          tunnel: w2297 -> [w2307 w2331]
          tunnel: w2291 -> [w2306 _]
          frame False {
            n899 = Concatenate Strings("O usuário \"", w2311, "\" será removido.\nContinuar?") -> (w2309:string)
            n900 = Concatenate Strings("The user \"", w2311, "\" will be removed.\nAre you sure?") -> (w2310:string)
            n901 = Select(t=w2309, s=w2307, f=w2310) -> (s? t:f=w2308:string)
            n902 = Two Button Dialog(message=w2308) -> (T button?=w2316:bool)  [unwired: 2 in]
            n903 = case shown="True" w2316 {
              tunnel: w2315 -> [_ w2322]
              tunnel: w2314 -> [_ w2321]
              tunnel: w2306 -> [_ w2320]
              frame False {
              }
              frame True {
                n904 = flat-sequence {
                  tunnel: w2322 -> [w2324]
                  tunnel: w2321 -> [w2326]
                  tunnel: w2320 -> [w2323]
                  tunnel: [w2323] -> w2319
                  tunnel: w2319 -> [w2327]
                  frame #0 {
                    n905 = Delete From Array(array=w2326, index=w2324) -> (array with subset deleted=w2325:T4)  [unwired: 1 in, 1 out]
                    n906 = local write "user list"(w2325) -> ()
                  }
                  frame #1 {
                    n907 = property on="user list" class="Arr (strict)"("Index Values"=w2327) -> ()  [unwired: 2 in, 2 out]
                  }
                }
              }
            }
          }
          frame True {
            n908 = Select(t="A auto-remoção não é permitida." ("message"), s=w2331, f="You can't delete yourself. " ("message")) -> (s? t:f=w2329:string)
            n909 = One Button Dialog(message=w2329) -> ()  [unwired: 1 in, 1 out]
          }
        }
      }
      event "change permission": Value Change {
        n910 = event-data() -> ()  [unwired: 1 in, 6 out]
        n911 = call "Read current user.vi"("error in (no error)"=w2352, "ICS in"=w2351) -> ("error out"=w2350:errorcluster, "current user"=w2332:string, "ICS out"=w2348:refnum<class "ICS.lvclass">)  [unwired: 7 in]
        n912 = local read "user list"() -> (w2343:T4)
        n913 = for {
          tunnel: w2343 -> [w2360] mode=indexing
          shift-right: [w2359] -> w2339
          shift-left: 0 ("index") -> [w2357]
          n914 = Unbundle By Name(w2360) -> ("permission"=w2355:string)
          n915 = Equal?(x="Admin", y=w2355) -> (x = y?=w2358:bool)
          n916 = Increment(x=w2357) -> (x+1=w2356:i32)
          n917 = Select(t=w2356, s=w2358, f=w2357) -> (s? t:f=w2359:i32)
        }
        n918 = property on="user list" class="Arr (strict)"() -> ("Index Values"=w2347:u32[])  [unwired: 2 in, 2 out]
        n919 = local read "user permission"() -> (w2333:string)
        n920 = Index Array(array=w2347, index=0) -> (element=w2349:u32)
        n921 = Index Array(array=w2343, index=w2349) -> (element=w2346:T20)
        n922 = Unbundle By Name(w2346) -> ("name"=w2345:string, "password"=w2344:string)  [unwired: 1 out]
        n923 = Greater?(x=w2339, y=u32 1) -> (0:w2337:bool)
        n924 = Equal?(x=w2345, y=w2332) -> (x = y?=w2334:bool)
        n925 = Equal?(x=w2333, y="Admin") -> (x = y?=w2338:bool)
        n926 = And(x=w2338, y=w2337) -> (x .and. y?=w2336:bool)
        n927 = Or(x=w2336, y=w2334) -> (x .or. y?=w2335:bool)
        n928 = case shown="True" w2335 {
          tunnel: w2346 -> [w2365 _]
          tunnel: w2344 -> [w2363 _]
          tunnel: w2345 -> [w2364 _]
          tunnel: w2343 -> [w2368 _]
          tunnel: w2349 -> [w2367 _]
          tunnel: w2333 -> [w2361 _]
          tunnel: w2334 -> [_ w2379]
          frame False {
            # "EXCHANGE PERMISSION"
            n929 = Bundle By Name(cluster=w2365, "name"=w2364, "permission"=w2361, "password"=w2363) -> (w2362:T20)
            n930 = Replace Array Subset(array=w2368, new element=w2362, index=w2367) -> (w2366:T4)
            n931 = local write "user list"(w2366) -> ()
          }
          frame True {
            # "INVALID ENTRY"
            n932 = local read "language"() -> (w2371:enum32{"PT", "EN", "NONE"})
            n933 = Not Equal?(x=w2371, y=enum32{"PT", "EN", "NONE"}."EN" ("language")) -> (x != y?=w2370:bool)
            n934 = Select(t="Você não pode mudar\nsua própria permissão. " ("message"), s=w2370, f="You can't exchange \nyour own permission. " ("message")) -> (s? t:f=w2374:string)
            n935 = Select(t="A permissão Admin é\nlimitada a 2 usuários." ("message"), s=w2370, f="Admin permission\nlimited to only 2 users." ("message")) -> (s? t:f=w2373:string)
            n936 = Select(t=w2374, s=w2379, f=w2373) -> (s? t:f=w2372:string)
            n937 = One Button Dialog(message=w2372) -> ()  [unwired: 1 in, 1 out]
          }
        }
      }
      event "user insert": Value Change {
        # "Check\nconfig \nuser qty."
        # "Check for empty name"
        # "Check for equal names"
        n938 = event-data() -> ()  [unwired: 1 in, 6 out]
        n939 = local read "user list"() -> (w2381:T4)
        n940 = for {
          tunnel: w2381 -> [w2404] mode=indexing
          tunnel: [w2407] -> w2395
          tunnel: "user name" -> [w2405]
          tunnel: [w2404] -> w2394
          stop <- w2407 stop-if-true
          n941 = Unbundle By Name(w2404) -> ("name"=w2406:string)
          n942 = Equal?(x=w2405, y=w2406) -> (x = y?=w2407:bool)
        }
        n943 = for {
          tunnel: w2381 -> [w2403] mode=indexing
          shift-right: [w2402] -> w2390
          shift-left: u32 0 ("x") -> [w2400]
          n944 = Unbundle By Name(w2403) -> ("permission"=w2398:string)
          n945 = Equal?(x="Admin", y=w2398) -> (x = y?=w2401:bool)
          n946 = Increment(x=w2400) -> (x+1=w2399:u32)
          n947 = Select(t=w2399, s=w2401, f=w2400) -> (s? t:f=w2402:u32)
        }
        n948 = Empty String/Path?(string/path="user name") -> (empty?=w2396:bool)
        n949 = Or(x=w2396, y=w2395) -> (x .or. y?=w2386:bool)
        n950 = Greater?(x=w2390, y=u32 1) -> (0:w2380:bool)
        n951 = Equal?(x="user permission", y="Admin") -> (x = y?=w2387:bool)
        n952 = And(x=w2387, y=w2380) -> (x .and. y?=w2385:bool)
        n953 = Or(x=w2385, y=w2386) -> (x .or. y?=w2384:bool)
        n954 = case shown="True" w2384 {
          tunnel: w2381 -> [w2417 _]
          tunnel: w2394 -> [w2416 _]
          tunnel: "user name" -> [w2415 _]
          tunnel: "user permission" -> [w2411 _]
          tunnel: w2380 -> [_ w2427]
          frame False {
            w2409 = ""
            # "INSERT USER INTO USER LIST"
            n955 = Array Size(array=w2417) -> (size(s)=w2413:i32)
            n956 = Bundle By Name(cluster=w2416, "name"=w2415, "permission"=w2411, "password"=w2409) -> (w2414:T20)
            n957 = local write "user name"(w2409) -> ()
            n958 = Build Array(w2413) -> (w2412:i32[])
            n959 = property on="user list" class="Arr (strict)"("Index Values"=w2412) -> ()  [unwired: 2 in, 2 out]
            n960 = Insert Into Array(array=w2417, new element=w2414) -> (w2408:T4)  [unwired: 1 in]
            n961 = property on="user name" class="Str"("Key Focus"=TRUE) -> ()  [unwired: 2 in, 2 out]
            n962 = local write "user list"(w2408) -> ()
          }
          frame True {
            # "INVALID USER NAME"
            n963 = local read "language"() -> (w2426:enum32{"PT", "EN", "NONE"})
            n964 = Not Equal?(x=w2426, y=enum32{"PT", "EN", "NONE"}."EN" ("language")) -> (x != y?=w2425:bool)
            n965 = Select(t="A permissão Admin é\nlimitada a 2 usuários." ("message"), s=w2425, f="Admin permission\nlimited to only 2 users." ("message")) -> (s? t:f=w2420:string)
            n966 = Select(t="Nome de usuário inválido" ("message"), s=w2425, f="Invalid user name." ("message")) -> (s? t:f=w2419:string)
            n967 = Select(t=w2420, s=w2427, f=w2419) -> (s? t:f=w2428:string)
            n968 = One Button Dialog(message=w2428) -> ()  [unwired: 1 in, 1 out]
          }
        }
      }
      event "check email": Value Change {
        n969 = event-data() -> ()  [unwired: 1 in, 6 out]
        n970 = local read "language"() -> (w2444:enum32{"PT", "EN", "NONE"})
        n971 = property on="email ok" class="Bool (strict)"(error in=w2433, "DisabledEnum"=T12."Enabled" ("Disabled")) -> (error out=w2447:errorcluster)  [unwired: 1 in, 1 out]
        n972 = Not Equal?(x=w2444, y=enum32{"PT", "EN", "NONE"}."EN" ("language")) -> (x != y?=w2443:bool)
        n973 = call "Get attributes.vi"("error in (no error)"=w2433, "ICS in"=w2436) -> ("error out"=w2435:errorcluster, "email settings"=w2432:T10, "ICS out"=w2434:refnum<class "ICS.lvclass">)  [unwired: 6 in, 1 out]
        n974 = Bundle By Name(cluster=w2432, "email enabled"=TRUE) -> (w2431:T10)
        n975 = property on="email ok" class="Bool (strict)"(error in=w2447, "Blinking"=TRUE) -> (error out=w2429:errorcluster)  [unwired: 1 in, 1 out]
        n976 = Select(t="O S4ICS está testando o e-mail.\nPor favor, não responda a\nesta menssagem.\n" ("menssagem:"), s=w2443, f="S4ICS is testing the email service.\nPlease do not reply to this message.\n" ("menssagem:")) -> (s? t:f=w2438:string)
        n977 = call "Send email.vi"("error in (no error)"=w2429, "message"=w2438, "email settings"=w2431) -> ("error out"=w2437:errorcluster, "fail"=w2439:bool)  [unwired: 7 in]
        n978 = Not(x=w2439) -> (.not. x?=→"email ok":bool)
        n979 = property on="email ok" class="Bool (strict)"(error in=w2437, "Blinking"=FALSE) -> ()  [unwired: 1 in, 2 out]
      }
      event "pwrPM mains": Value Change {
        n980 = event-data() -> ()  [unwired: 1 in, 6 out]
        n981 = Select(t=T12."Disabled and Grayed Out" ("Disabled"), s="pwrPM mains", f=T12."Enabled" ("Disabled")) -> (s? t:f=w2453:T12)
        n982 = property on="pwrPM ip" class="Str"("DisabledEnum"=w2453) -> ()  [unwired: 2 in, 2 out]
        n983 = property on="pwrPM port" class="DigNum (strict)"("DisabledEnum"=w2453) -> ()  [unwired: 2 in, 2 out]
        n984 = property on="pwrPM user" class="Str"("DisabledEnum"=w2453) -> ()  [unwired: 2 in, 2 out]
        n985 = property on="pwrPM password" class="Str"("DisabledEnum"=w2453) -> ()  [unwired: 2 in, 2 out]
        n986 = property on="pwrPM outlet" class="DigNum (strict)"("DisabledEnum"=w2453) -> ()  [unwired: 2 in, 2 out]
      }
      event "pwrGD mains": Value Change {
        n987 = event-data() -> ()  [unwired: 1 in, 6 out]
        n988 = Select(t=T12."Disabled and Grayed Out" ("Disabled"), s="pwrGD mains", f=T12."Enabled" ("Disabled")) -> (s? t:f=w2459:T12)
        n989 = property on="pwrGD ip" class="Str"("DisabledEnum"=w2459) -> ()  [unwired: 2 in, 2 out]
        n990 = property on="pwrGD port" class="DigNum (strict)"("DisabledEnum"=w2459) -> ()  [unwired: 2 in, 2 out]
        n991 = property on="pwrGD user" class="Str"("DisabledEnum"=w2459) -> ()  [unwired: 2 in, 2 out]
        n992 = property on="pwrGD password" class="Str"("DisabledEnum"=w2459) -> ()  [unwired: 2 in, 2 out]
        n993 = property on="pwrGD outlet" class="DigNum (strict)"("DisabledEnum"=w2459) -> ()  [unwired: 2 in, 2 out]
      }
      event "return setup": Value Change {
        # "RECOVER THE LAST CONFIGURATION FROM DATALOG FILE TO CANCEL ALL CHANGES."
        n994 = event-data() -> ()  [unwired: 1 in, 6 out]
        n995 = call "Get attributes.vi"("error in (no error)"=w2468, "ICS in"=w2480) -> ("error out"=w2471:errorcluster, "email settings"=w2466:T10, "control indices"=w2470:i32[], "ICS out"=w2473:refnum<class "ICS.lvclass">)  [unwired: 6 in]
        n996 = local read "cfgFile"() -> (w2475:string)
        n997 = call <vilib>:"Application Directory.vi"() -> ("Application Directory"=w2476:path)
        n998 = Build Array(u32 0) -> (w2478:u32[])
        n999 = Get Control Values by Index(1:w2470, 3:w2471) -> (10:w2469:variant[], 11:w2467:errorcluster)  [unwired: 1 in]
        n1000 = Build Path(base path=w2476, name or relative path=w2475) -> (appended path=w2472:path)
        n1001 = local write "tab menu"(T6."Stopped" ("tab menu")) -> ()
        n1002 = local write "tab body"(enum32{"Motors", "Config"}."Motors" ("tab body")) -> ()
        n1003 = property on="user list" class="Arr (strict)"("Index Values"=w2478) -> ()  [unwired: 2 in, 2 out]
        n1004 = call "Config file.vi"("path"=w2472, "access (0:read/write)"=enum16{"read/write", "read-only", "write-only"}."read-only", "error in (no error)"=w2467, "data values"=w2469, "email settings"=w2466) -> ("error out"=w2465:errorcluster, "data out"=w2464:variant[])  [unwired: 5 in]
        n1005 = Set Control Values by Index(1:w2470, 2:w2464, 3:w2465) -> (11:w2474:errorcluster)  [unwired: 1 in]
      }
      event "control": Value Change {
        w2483 = T12."Disabled and Grayed Out" ("Disabled")
        # "TEMPORARY. THE\nGOTO SUBROUTINES OF ALL MOTORS MUST\nBE STORED INTO MOTOR MEMORY IN ORDER TO ENABLE THE JUMP FUNCTION."
        n1006 = event-data() -> ()  [unwired: 1 in, 6 out]
        n1007 = local write "tab menu"(T6."Control" ("tab menu")) -> ()
        n1008 = local write "tab body"(enum32{"Motors", "Config"}."Motors" ("tab body")) -> ()
        n1009 = local read "WPROT disabled"() -> (w2490:bool)
        n1010 = local read "WPSEL disabled"() -> (w2491:bool)
        n1011 = local read "CALW disabled"() -> (w2489:bool)
        n1012 = local read "GMIR disabled"() -> (w2488:bool)
        n1013 = local read "ASEL disabled"() -> (w2492:bool)
        n1014 = property on="control motor sel" class="RadioBtnsControl (strict)"("Value"=T7."No Selection" ("control motor sel")) -> ()  [unwired: 2 in, 2 out]
        n1015 = property on="control motor sel" class="RadioBtnsControl (strict)"() -> ("Controls[]"=w2487:refnum<vi>[])  [unwired: 2 in, 2 out]
        n1016 = Build Array(w2490, w2491, w2492, w2489, w2488, w2488) -> (w2486:bool[])
        n1017 = for {
          tunnel: w2487 -> [w2498] mode=indexing
          tunnel: w2486 -> [w2500] mode=indexing
          tunnel: T12."Disabled" ("Disabled") -> [w2497]
          tunnel: T12."Enabled" ("Disabled") -> [w2496]
          # "APPLY CONFIG.\nDISABLE CONTROLS TO MOTOR SELECTOR"
          n1018 = Select(t=w2497, s=w2500, f=w2496) -> (s? t:f=w2499:T12)
          n1019 = property class="Ctl"(reference=w2498, "DisabledEnum"=w2499) -> ()  [unwired: 1 in, 2 out]
        }
        n1020 = property on="control send" class="Bool"("DisabledEnum"=w2483) -> ()  [unwired: 2 in, 2 out]
        n1021 = property on="control jump" class="Bool"("DisabledEnum"=w2483) -> ()  [unwired: 2 in, 2 out]
        n1022 = property on="control jump" class="Bool"("DisabledEnum"=w2483) -> ()  [unwired: 2 in, 2 out]
        n1023 = property on="control position" class="DigNum (strict)"("DisabledEnum"=w2483) -> ()  [unwired: 2 in, 2 out]
      }
      event "control motor sel": Value Change {
        n1024 = event-data() -> ()  [unwired: 1 in, 6 out]
        n1025 = Equal?(x="control motor sel", y=T7."No Selection" ("control motor sel")) -> (x = y?=w2507:bool)
        n1026 = case shown="\"No Selection\", Default" "control motor sel" {
          tunnel: [w2512 w2513 w2514 w2515 w2516 w2517 ""] -> w2502
          frame "control WPROT" {
            # "GET MOTOR IP"
            n1027 = local read "WPROT ip"() -> (w2512:string)
          }
          frame "control WPSEL" {
            # "GET MOTOR IP"
            n1028 = local read "WPSEL ip"() -> (w2513:string)
          }
          frame "control ASEL" {
            # "GET MOTOR IP"
            n1029 = local read "ASEL ip"() -> (w2514:string)
          }
          frame "control CALW" {
            # "GET MOTOR IP"
            n1030 = local read "CALW ip"() -> (w2515:string)
          }
          frame "control GFOC" {
            # "GET MOTOR IP"
            n1031 = local read "GMIR ip"() -> (w2516:string)
          }
          frame "control GMIR" {
            # "GET MOTOR IP"
            n1032 = local read "GMIR ip"() -> (w2517:string)
          }
          frame "No Selection", Default {
            # "GET MOTOR IP"
          }
        }
        n1033 = Select(t=T12."Disabled and Grayed Out" ("Disabled"), s=w2507, f=T12."Enabled" ("Disabled")) -> (s? t:f=w2509:T12)
        n1034 = call "Write motor IP.vi"("error in (no error)"=w2505, "motor IP"=w2502, "ICS in"=w2506) -> ("error out"=w2504:errorcluster, "ICS out"=w2503:refnum<class "ICS.lvclass">)  [unwired: 7 in]
        n1035 = property on="control jump" class="Bool"("DisabledEnum"=w2509) -> ()  [unwired: 2 in, 2 out]
        n1036 = property on="control send" class="Bool"("DisabledEnum"=w2509) -> ()  [unwired: 2 in, 2 out]
      }
      event "control send": Value Change {
        n1037 = event-data() -> ()  [unwired: 1 in, 6 out]
        n1038 = call-dynamic "Read motor IP.vi"("error in (no error)"=w2524, "ICS in"=w2523) -> ("error out"=w2522:errorcluster, "motor IP"=w2519:string, "ICS out"=w2521:refnum<class "ICS.lvclass">)  [unwired: 7 in]
        n1039 = Empty String/Path?(string/path="control instruction") -> (empty?=w2525:bool)
        n1040 = Empty String/Path?(string/path=w2519) -> (empty?=w2520:bool)
        n1041 = Or(x=w2525, y=w2520) -> (x .or. y?=w2526:bool)
        n1042 = case shown="False" w2526 {
          tunnel: w2522 -> [w2544 w2550]
          tunnel: "control instruction" -> [w2543 _]
          tunnel: [w2530 w2550] -> w2527
          tunnel: w2519 -> [w2529 _]
          frame False {
            # "SEND INSTRUCTION AND WAITS FOR MOTOR RESPONSE"
            n1043 = call "Send batch.vi"("error in (no error)"=w2544, "motor ip"=w2529, "instruction"=w2543) -> ("error out"=w2541:errorcluster, "ok"=w2535:bool, "response"=→"control response":string)  [unwired: 4 in, 2 out]
            n1044 = call <vilib>:"Space Constant.vi"() -> ("String"=w2542:string)
            n1045 = Search and Replace String(replace all?=TRUE ("replace all? (F)"), input string=w2543, search string=w2542, error in=w2541) -> (result string=w2539:string, error out=w2530:errorcluster)  [unwired: 4 in, 2 out]
            n1046 = Match Pattern(string=w2539, regular expression="EO=") -> (after substring=w2534:string, offset past match=w2537:i32)  [unwired: 1 in, 2 out]
            n1047 = Equal?(x="1" ("regular expression"), y=w2534) -> (x = y?=w2531:bool)
            n1048 = Greater Or Equal To 0?(x=w2537) -> (x >= 0?=w2536:bool)
            n1049 = And(x=w2535, y=w2536) -> (x .and. y?=w2532:bool)
            n1050 = case shown="True" w2532 {
              tunnel: w2531 -> [_ w2549]
              frame False {
              }
              frame True {
                # "DIS/ENABLE ACCORDING TO MOTOR EO (ENABLE OUTPUT)"
                n1051 = Select(t=T12."Disabled and Grayed Out" ("Disabled"), s=w2549, f=T12."Enabled" ("Disabled")) -> (s? t:f=w2546:T12)
                n1052 = property on="return control" class="Bool"("DisabledEnum"=w2546) -> ()  [unwired: 2 in, 2 out]
                n1053 = property on="control motor sel" class="RadioBtnsControl (strict)"("DisabledEnum"=w2546) -> ()  [unwired: 2 in, 2 out]
              }
            }
          }
          frame True {
            # "NO COMMAND, DO NOTHING"
          }
        }
      }
      event "control jump": Value Change {
        # "MECH.   RANGE    UNIT    DMX-ETH\nWPROT  0 - 360  degree  0 - 36000\nWPSEL  0 - 100     %    0 - 10000\nASEL   0 - 100     %    0 - 10000\nCALW   0 - 360  degree  0 - 36000\nGMIR   0 - 360  degree  0 - 36000\nGFOC   0 - 20     mm    0 - 20000"
        n1054 = event-data() -> ()  [unwired: 1 in, 6 out]
        n1055 = local read "control motor sel"() -> (w2555:T7)
        n1056 = Equal?(x=T7."No Selection" ("control motor sel"), y=w2555) -> (x = y?=w2554:bool)
        n1057 = case shown="False" w2554 {
          tunnel: w2555 -> [w2572 _]
          tunnel: w2553 -> [w2571 w2599]
          tunnel: [w2569 w2599] -> w2552
          frame False {
            # "CALL GOTO SUBROUTINE"
            n1058 = case shown="\"No Selection\", Default" w2572 {
              tunnel: [w2581 w2584 w2587 w2590 w2593 w2596 w2597] -> w2560
              tunnel: [100.0 ("y") 100.0 ("y") 100.0 ("y") 100.0 ("y") 100.0 ("y") 1000.0 ("y") 0.0 ("y")] -> w2567
              tunnel: ["GOSUB 12" "GOSUB 13" "GOSUB 14" "GOSUB 15" "GOSUB 16" "GOSUB 17" w2597] -> w2559
              frame "control WPROT" {
                # "MOTOR INDEX"
                n1059 = local read "WPROT ip"() -> (w2581:string)
              }
              frame "control WPSEL" {
                # "MOTOR INDEX"
                n1060 = local read "WPSEL ip"() -> (w2584:string)
              }
              frame "control ASEL" {
                # "MOTOR INDEX"
                n1061 = local read "ASEL ip"() -> (w2587:string)
              }
              frame "control CALW" {
                # "MOTOR INDEX"
                n1062 = local read "CALW ip"() -> (w2590:string)
              }
              frame "control GFOC" {
                # "MOTOR INDEX"
                n1063 = local read "GMIR ip"() -> (w2593:string)
              }
              frame "control GMIR" {
                # "MOTOR INDEX"
                n1064 = local read "GMIR ip"() -> (w2596:string)
              }
              frame "No Selection", Default {
                w2597 = ""
                # "MOTOR INDEX"
              }
            }
            n1065 = Multiply(x="control position", y=w2567) -> (x*y=w2566:dbl)
            n1066 = To Long Integer(number=w2566) -> (32bit integer=w2564:i32)
            n1067 = Number To Decimal String(number=w2564) -> (decimal integer string=w2563:string)  [unwired: 1 in]
            n1068 = Concatenate Strings(w2563, "V12=") -> (w2562:string)
            n1069 = call "Send instruction.vi"("error in (no error)"=w2571, "motor ip"=w2560, "instruction"=w2562) -> ("error out"=w2570:errorcluster, "response"=w2561:string)  [unwired: 5 in, 2 out]
            n1070 = flat-sequence {
              tunnel: w2562 -> [w2578]
              tunnel: w2561 -> [w2577]
              tunnel: [w2575] -> w2557
              frame #0 {
                n1071 = local write "control instruction"(w2578) -> ()
                n1072 = local write "control response"(w2577) -> ()
                n1073 = Wait (ms)(milliseconds to wait=u32 250) -> (millisecond timer value=w2575:u32)
              }
            }
            n1074 = call "Send instruction.vi"("error in (no error)"=w2570, "motor ip"=w2560, "instruction"=w2559) -> ("error out"=w2569:errorcluster, "response"=w2558:string)  [unwired: 5 in, 2 out]
            n1075 = flat-sequence {
              tunnel: w2559 -> [w2574]
              tunnel: w2558 -> [w2573]
              tunnel: w2557 -> [_]
              frame #0 {
                n1076 = local write "control instruction"(w2574) -> ()
                n1077 = local write "control response"(w2573) -> ()
              }
            }
          }
          frame True {
            # "NO COMMAND, DO NOTHING"
          }
        }
      }
      event "control stop": Value Change {
        n1078 = event-data() -> ()  [unwired: 1 in, 6 out]
        n1079 = local read "control motor sel"() -> (w2604:T7)
        n1080 = Equal?(x=T7."No Selection" ("control motor sel"), y=w2604) -> (x = y?=w2603:bool)
        n1081 = case shown="False" w2603 {
          tunnel: w2604 -> [w2611 _]
          tunnel: w2602 -> [w2610 w2621]
          tunnel: [w2608 w2621] -> w2601
          frame False {
            w2606 = "STOPX" ("regular expression")
            # "SEND STOP INSTRUCTION"
            n1082 = case shown="\"No Selection\", Default" w2611 {
              tunnel: [w2614 w2615 w2616 w2617 w2618 w2619 ""] -> w2609
              frame "control WPROT" {
                # "MOTOR INDEX"
                n1083 = local read "WPROT ip"() -> (w2614:string)
              }
              frame "control WPSEL" {
                # "MOTOR INDEX"
                n1084 = local read "WPSEL ip"() -> (w2615:string)
              }
              frame "control ASEL" {
                # "MOTOR INDEX"
                n1085 = local read "ASEL ip"() -> (w2616:string)
              }
              frame "control CALW" {
                # "MOTOR INDEX"
                n1086 = local read "CALW ip"() -> (w2617:string)
              }
              frame "control GFOC" {
                # "MOTOR INDEX"
                n1087 = local read "GMIR ip"() -> (w2618:string)
              }
              frame "control GMIR" {
                # "MOTOR INDEX"
                n1088 = local read "GMIR ip"() -> (w2619:string)
              }
              frame "No Selection", Default {
                # "MOTOR INDEX"
              }
            }
            n1089 = call "Send instruction.vi"("error in (no error)"=w2610, "motor ip"=w2609, "instruction"=w2606) -> ("error out"=w2608:errorcluster, "response"=w2607:string)  [unwired: 5 in, 2 out]
            n1090 = flat-sequence {
              tunnel: w2606 -> [w2613]
              tunnel: w2607 -> [w2612]
              frame #0 {
                n1091 = local write "control instruction"(w2613) -> ()
                n1092 = local write "control response"(w2612) -> ()
              }
            }
          }
          frame True {
            # "NO COMMAND, DO NOTHING"
          }
        }
      }
      event "return control": Value Change {
        w2624 = ""
        n1093 = event-data() -> ()  [unwired: 1 in, 6 out]
        n1094 = call "Write motor IP.vi"("error in (no error)"=w2629, "motor IP"="", "ICS in"=w2628) -> ("error out"=w2626:errorcluster, "ICS out"=w2627:refnum<class "ICS.lvclass">)  [unwired: 7 in]
        n1095 = local write "tab menu"(T6."Stopped" ("tab menu")) -> ()
        n1096 = local write "tab body"(enum32{"Motors", "Config"}."Motors" ("tab body")) -> ()
        n1097 = local write "control motor sel"(T7."No Selection" ("control motor sel")) -> ()
        n1098 = local write "control response"(w2624) -> ()
        n1099 = local write "control instruction"(w2624) -> ()
      }
    }
    n1100 = call-dynamic "Publish 0mq.vi"("error in (no error)"=w251, "ICS in"=w252) -> ("error out"=w250:errorcluster, "ICS out"=w249:refnum<class "ICS.lvclass">)  [unwired: 8 in]
    n1101 = case shown="True" "animation" {
      tunnel: w249 -> [w265 w271]
      tunnel: [w265 w268] -> w258
      tunnel: [w264 w267] -> w257
      tunnel: w250 -> [w264 w266]
      frame False {
      }
      frame True {
        n1102 = call-dynamic "Read motors.vi"("error in (no error)"=w266, "ICS in"=w271) -> ("error out"=w267:errorcluster, "motors"=w270:refnum<class "Motor.lvclass">[], "ICS out"=w268:refnum<class "ICS.lvclass">)  [unwired: 7 in]
        n1103 = for {
          tunnel: w270 -> [w276] mode=indexing
          tunnel: w267 -> [w277]
          shift-right: [w275] -> _
          shift-left: FALSE -> [w274]
          n1104 = call-dynamic "Get name and position.vi"("error in (no error)"=w277, "Motor in"=w276) -> ("position"=w272:dbl, "name"=w273:string)  [unwired: 6 in, 2 out]
          n1105 = case shown="\"WPSEL\", Default" w273 {
            tunnel: w272 -> [w292 w308 w321 w360 w372 w388]
            tunnel: [w291 w307 w320 w359 w373 w387] -> w275
            tunnel: w274 -> [w291 w307 w320 w359 w373 _]
            frame "WPSEL", Default {
              w278 = 160.0 ("RANGE")
              # "MAX"
              # "X0"
              # "RANGE"
              n1106 = Equal To 0?(x=w292) -> (x = 0?=w288:bool)
              "wpsel lim/2" <- w288
              n1107 = Equal?(x=w278, y=w292) -> (x = y?=w289:bool)
              "wpsel lim/4" <- w289
              n1108 = Multiply(x=182.0 ("RANGE"), y=w292) -> (x*y=w286:dbl)
              n1109 = Divide(x=w286, y=w278) -> (x/y=w285:dbl)
              n1110 = Or(x=w288, y=w289) -> (x .or. y?=w290:bool)
              n1111 = In Range and Coerce(upper limit=80.5 ("RANGE"), x=w292, lower limit=79.5 ("RANGE")) -> (In Range?=w279:bool)  [unwired: 1 out]
              n1112 = Or(x=w291, y=w279) -> (x .or. y?=→"wp home":bool)
              n1113 = property on="wprot ctl" class="Knob (strict)"("Visible"=w290) -> ()  [unwired: 2 in, 2 out]
              n1114 = Add(x=113.0 ("OFFSET"), y=w285) -> (x+y=w287:dbl)
              n1115 = property on="wpsel anime" class="Pict"("Left"=w287) -> ()  [unwired: 2 in, 2 out]
              "WPSEL Value" <- w292
            }
            frame "ASEL" {
              (unwired) 100.0 ("y")
              (unwired) 100.0 ("ASEL position")
              # "MAX"
              n1116 = local read "asel image"() -> (w306:T2)
              n1117 = Divide(x=-30.0 ("ASEL position"), y=30.0 ("ASEL position")) -> (x/y=w303:dbl)
              n1118 = Multiply(x=w303, y=w308) -> (x*y=w302:dbl)
              n1119 = Less Or Equal To 0?(x=w308) -> (x <= 0?=→"asel lim off":bool)
              n1120 = Greater Or Equal?(x=w308, y=28.0) -> (x >= y?=→"asel lim on":bool)
              n1121 = call "Picture Rotation.vi"("transparent?"=TRUE, "theta (deg)"=w302, "image data in"=w306) -> ("image data out"=w301:T2)  [unwired: 7 in, 1 out]
              n1122 = call <vilib>:"Get Image Subset.vi"("subset rect"=T14 {"left"=276, "top"=25, "right"=700, "bottom"=480}, "image data"=w301) -> ("image subset"=w299:T2)  [unwired: 4 in, 1 out]
              n1123 = call <vilib>:"Draw Flattened Pixmap.vi"("image data"=w299, "picture"=picture data[5B]) -> ("new picture"=→"asel anime":picture)  [unwired: 7 in]
              "ASEL Value" <- w308
            }
            frame "CALW" {
              n1124 = Absolute Value(x=w321) -> (abs(x)=w314:dbl)
              n1125 = Quotient & Remainder(x=w314, y=360.0) -> (x-y*floor(x/y)=w319:dbl)  [unwired: 1 out]
              n1126 = Cluster To Array(cluster=cluster{dbl, dbl, dbl, dbl, dbl} {0.0, 72.0, 144.0, 216.0, 288.0} ("Knob")) -> (array=w312:dbl[])
              n1127 = for {
                tunnel: w312 -> [w344] mode=indexing
                tunnel: [w346] -> w311 mode=indexing
                tunnel: w319 -> [w342]
                # "OFFSET"
                n1128 = Subtract(x=360.0 ("y"), y=w344) -> (x-y=w343:dbl)
                n1129 = Add(x=w342, y=10.0) -> (x+y=w341:dbl)
                n1130 = Subtract(x=w341, y=w343) -> (x-y=w347:dbl)
                n1131 = Add(x=w344, y=w341) -> (x+y=w348:dbl)
                n1132 = Greater Or Equal?(x=w348, y=360.0) -> (x >= y?=w349:bool)
                n1133 = Select(t=w347, s=w349, f=w348) -> (s? t:f=w346:dbl)
              }
              n1134 = To Word Integer(number=w319) -> (16bit integer=w315:i16)
              n1135 = Array To Cluster(array=w311) -> (cluster=w313:T21)
              n1136 = case shown="-1, Default" w315 {
                tunnel: [TRUE FALSE TRUE FALSE TRUE FALSE] -> w316
                tunnel: [FALSE FALSE FALSE TRUE TRUE FALSE] -> w317
                tunnel: [FALSE TRUE TRUE FALSE FALSE FALSE] -> w318
                frame 0 {
                }
                frame 72 {
                }
                frame 144 {
                }
                frame 216 {
                }
                frame 288 {
                }
                frame -1, Default {
                }
              }
              "calw0" <- w316
              "calw1" <- w318
              "calw2" <- w317
              n1137 = local write "calw knob"(w313) -> ()
              "CALW Value" <- w321
            }
            frame "GFOC" {
              w351 = 25.0 ("x")
              # "MAX"
              # "X0"
              # "RANGE"
              n1138 = Multiply(x=22.0, y=w360) -> (x*y=w355:dbl)
              n1139 = Equal To 0?(x=w360) -> (x = 0?=→"GFOC home":bool)
              n1140 = Equal?(x=w351, y=w360) -> (x = y?=→"GFOC limit":bool)
              n1141 = Divide(x=w355, y=w351) -> (x/y=w356:dbl)
              n1142 = Add(x=73.0, y=w356) -> (x+y=w354:dbl)
              n1143 = property on="guider cam anime" class="Pict"("Left"=w354) -> ()  [unwired: 2 in, 2 out]
              "GFOC Value" <- w360
            }
            frame "GMIR" {
              n1144 = Absolute Value(x=w372) -> (abs(x)=w366:dbl)
              n1145 = Quotient & Remainder(x=w366, y=360.0) -> (x-y*floor(x/y)=w365:dbl)  [unwired: 1 out]
              n1146 = Subtract(x=w365, y=0.0) -> (x-y=w370:dbl)
              n1147 = Add(x=0.0, y=w365) -> (x+y=w369:dbl)
              n1148 = Equal To 0?(x=w365) -> (x = 0?=→"GMIR home":bool)
              n1149 = Greater Or Equal?(x=w369, y=360.0) -> (x >= y?=w368:bool)
              n1150 = Select(t=w370, s=w368, f=w369) -> (s? t:f=→"gmir knob":dbl)
              "GMIR Value" <- w372
            }
            frame "WPROT" {
              n1151 = Absolute Value(x=w388) -> (abs(x)=w382:dbl)
              n1152 = Quotient & Remainder(x=w382, y=360.0) -> (x-y*floor(x/y)=w376:dbl)  [unwired: 1 out]
              n1153 = Subtract(x=w376, y=0.0) -> (x-y=w385:dbl)
              n1154 = Add(x=0.0, y=w376) -> (x+y=w384:dbl)
              n1155 = Greater Or Equal?(x=w384, y=360.0) -> (x >= y?=w383:bool)
              n1156 = property on="wprot ctl" class="Knob (strict)"() -> ("Visible"=w374:bool)  [unwired: 2 in, 2 out]
              n1157 = Less Or Equal?(x=w376, y=0.5) -> (x <= y?=w375:bool)
              n1158 = Select(t=w385, s=w383, f=w384) -> (s? t:f=→"wprot ctl":dbl)
              n1159 = And(x=w374, y=w375) -> (x .and. y?=w387:bool)
              "WPROT Value" <- w388
            }
          }
        }
      }
    }
    n1160 = flat-sequence {
      frame #0 {
        # "ANIMAÇÃO DO PAINEL: 100ms"
      }
    }
  }
  n1161 = Bundle By Name(cluster=T8 {"S4commandQueueName"="", "S4statusQueueName"="", "comm configuration"={"channel"=enum."Local Panel", "address"="", "port"=0, "timeout"=0}} ("intercomm configuration"), "S4commandQueueName"="S4command", "S4statusQueueName"="S4status", "comm configuration.address"="0mqEndpoint", "comm configuration.timeout"="pubTime0mq") -> (w6:T8)
  n1162 = while {
    tunnel: w6 -> [w2632]
    tunnel: [w2631] -> w1
    stop <- w2631 stop-if-true
    # "THE 0MQ MANAGER STOPS RUNNING WHEN A EXIT MESSAGE IS READ FROM THE QUEUE BUT DOES NOT DESTROY THE QUEUES."
    # "RUNS THE ZEROMQ MANAGER"
    n1163 = call "0mqManager.vi"("intercomm configuration"=w2632) -> ("exit"=w2631:bool)  [unwired: 9 in, 1 out]
  }
  n1164 = flat-sequence {
    tunnel: w10 -> [w2639]
    tunnel: w30 -> [w2640]
    tunnel: w1 -> [_]
    frame #0 {
      w2645 = ""
      n1165 = call-dynamic "Read Messenger.vi"("error in (no error)"=w2639, "ICS in"=w2640) -> ("error out"=w2636:errorcluster, "Messenger.lvclass"=w2637:refnum<class "Messenger.lvclass">, "ICS out"=w2638:refnum<class "ICS.lvclass">)  [unwired: 7 in]
      n1166 = call "Read Server.vi"("error in (no error)"=w2636, "ICS in"=w2638) -> ("error out"=w2646:errorcluster, "Server"=w2648:refnum<class "TCP-Server.lvclass">)  [unwired: 7 in, 1 out]
      n1167 = disable-structure shown="Enabled" {
        disable-tunnel: w2637 -> [w2652 w2654]
        disable-tunnel: w2636 -> [w2651 w2655]
        disable-tunnel: [w2650 w2653] -> w2633
        frame Disabled {
          n1168 = call-dynamic "Stop 0mqComm.vi"("error in (no error)"=w2651, "Messenger in"=w2652) -> ("error out"=w2650:errorcluster)  [unwired: 8 in, 1 out]
        }
        frame Enabled {
          # "20240619"
          n1169 = call-dynamic "Destroy queues.vi"("error in (no error)"=w2655, "Messenger in"=w2654) -> ("error out"=w2653:errorcluster)  [unwired: 8 in, 1 out]
        }
      }
      n1170 = call "Read listenner.vi"("error in (no error)"=w2646, "Server in"=w2648) -> ("error out"=w2647:errorcluster, "listenner ID"=w2649:refnum<k5>)  [unwired: 7 in, 1 out]
      n1171 = local write "tab menu"(T6."Login" ("tab menu")) -> ()
      n1172 = local write "tab body"(enum32{"Motors", "Config"}."Motors" ("tab body")) -> ()
      n1173 = local write "loginUser"(w2645) -> ()
      n1174 = local write "loginPW"(w2645) -> ()
      n1175 = TCP Close Connection(connection ID=w2649, error in (no error)=w2647) -> (error out=w2634:errorcluster)  [unwired: 1 in, 1 out]
      n1176 = Merge Errors(w2634, w2633) -> (w2635:errorcluster)
      n1177 = property class="App"() -> ("App.Kind"=w2644:T22)  [unwired: 2 in, 2 out]
      n1178 = call <vilib>:"Clear Errors.vi"("error in (no error)"=w2635) -> ("error out"=w2643:errorcluster)  [unwired: 5 in, 1 out]
      n1179 = case shown="\"Run Time System\"" w2644 {
        tunnel: w2643 -> [_ _]
        frame "Development System", Default {
        }
        frame "Run Time System" {
          n1180 = Quit LabVIEW(quit? (T)=TRUE) -> ()
        }
      }
    }
  }
  "version" <- "20240620" ("version")
